vi "ScriptedStateMachine.vi"(8 "ErrorArray In":errorcluster[](array[cluster]), 9 "Data in":variant, 10 "Script":string[](array[string])=["Test,1,2,3", "stop"], 11 "Bus":refnum<class "Bus.lvclass">) -> (0 "ErrorArray Out":errorcluster[](array[cluster]), 2 "Data out":variant, 3 "Bus":refnum<class "Bus.lvclass">)   [LabVIEW 2017, in "Bus_class.lvlib" / "Bus.lvclass"]
uses:
  Bus.lvclass
  Public/TypeDefs/clBusData.ctl
  FrontPanel/TypeDefs/clEventConfig.ctl
  Modules/PmuImpairPlugins/PmuImpairPluginBase_class/TypeDefs/clImpairConfig.ctl
  Modules/EventPlugins/EventPluginBaseClass/TypeDefs/clEvtReportArray.ctl
  Modules/EventPlugins/EventPluginBaseClass/TypeDefs/clEvtReport.ctl
  Modules/EventPlugins/EventPluginBaseClass/TypeDefs/dblEvtSignalArray.ctl
  Modules/NetworkImpairmentModule/PublicAPI/Arguments/Broadcasts/dblNetworkTime.ctl
  Modules/NetworkImpairmentModule/PublicAPI/Arguments/Broadcasts/dblPktLoss.ctl
  Modules/FlagImpairModule/PublicAPI/Arguments/Broadcasts/ui32FlagImpairmentArray.ctl
  Modules/OutputToFilePlugins/OutputToFileBasePlugin/Typedefs/PmuCfgOpt.ctl
  Bus.lvclass/Bus.ctl
  BdcstInfo.ctl
  ModuleType.ctl
  FrontPanel/TypeDefs/clFrontPanelControlRefs.ctl
  Modules/PmuImpairModule/PublicAPI/Arguments/Broadcasts/clErrorRpt.ctl
  Modules/EventPlugins/EventPluginBaseClass/TypeDefs/clEvtConfig.ctl
  Accessors/Read AppModuleID.vi
  Accessors/Read OutputToFileModuleID.vi
  <vilib>/Utility/error.llb/Error Cluster From Error Code.vi
  <vilib>/Analysis/1siggen.llb/Ramp Pattern by Delta.vi
  <vilib>/ErrorRing/Error Ring.xnode
  <userlib>/NIST/NISTErrorLib/NISTErrorLib.lvlib
  Framework.lvlib
  Modules/EventModule/EventModule.lvlib
  Modules/EventPlugins/EventPluginBaseClass/EventPluginBaseClass.lvclass
  <vilib>/Analysis/NI_AALBase.lvlib
  Modules/PmuImpairModule/PmuImpairModule.lvlib
  Modules/NetworkImpairmentModule/NetworkImpairmentModule.lvlib
  Modules/FlagImpairModule/FlagImpairModule.lvlib
  Modules/PmuImpairPlugins/PmuImpairPluginBase_class/PmuImpairPluginBase.lvclass
  Modules/OutputToFilePlugins/OutputToFileBasePlugin/OutputToFileBasePlugin.lvclass
  Modules/OutputToFileModule/OutputToFileModule.lvlib
  Modules/AppModule/AppModule.lvlib
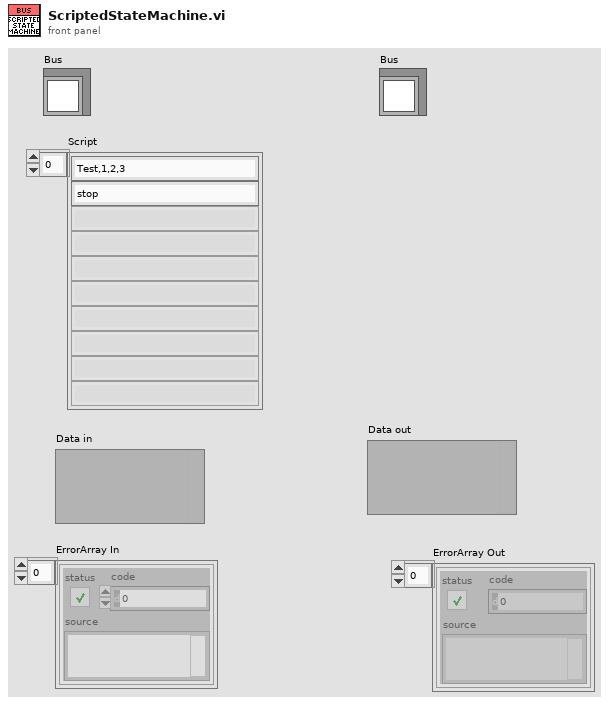
[diagram p1: front panel]
types:
  T1 = typedef "Bus_class.lvlib/Bus.lvclass/clBusData.ctl" = cluster{"BusNumber":u8, "EvtPluginINIFilePath":path, "EvtParams":string[][], "EvtConfig":T2, "Start Time":dbl, "End Time":dbl, "PmuImpairPluginINIFilePath":path, "PmuImpairParams ":string[][], "PmuImpairConfig":T3, "NetImpPluginINIFilePath":path, "NetImpParams":string[][], "FlagImpPluginINIFilePath":path, "FlagImpParams":string[][], "EvtReportArray":T4, "EventSignalArray":T6, "ImpairReportArray":T4, "NetworkTime":T7, "PktLoss":T8, "FlagImpArray":T9, "OutputToFilePluginINIFilePath":path, "Output File Path":path, "clConfigOptions":T10, "AppPluginINIFilePath":path, "AppConfig":variant, "AppOutput":variant}
  T2 = typedef "Framework.lvlib/clEventConfig.ctl" = cluster{"UTC Time 0":timestamp, "Nominal Frequency":u16, "Reporting Rate":u16, "Fsamp":u32, "PosSeq":bool}
  T3 = typedef "PmuImpairPlugins.lvlib/PmuImpairPluginBase.lvclass/clImpairConfig.ctl" = cluster{"FilterType":string, "bPosSeq":bool}
  T4 = typedef "EventPlugins.lvlib/EventPluginBaseClass.lvclass/clEvtReportArray.ctl" = T5[]
  T5 = typedef "EventPlugins.lvlib/EventPluginBaseClass.lvclass/clEvtReport.ctl" = cluster{"Timestamp":dbl, "Synx":cdb[], "Freq":dbl, "ROCOF":dbl, "ID":i16}
  T6 = typedef "EventPlugins.lvlib/EventPluginBaseClass.lvclass/dblEvtSignalArray.ctl" = dbl[][]
  T7 = typedef "NetworkImpairmentModule.lvlib/dblNetworkTime.ctl" = dbl[]
  T8 = typedef "NetworkImpairmentModule.lvlib/dblPktLoss.ctl" = dbl[]
  T9 = typedef "FlagImpairModule.lvlib/ui32FlagImpairmentArray.ctl" = u32[]
  T10 = typedef "OutputToFilePlugins.lvlib/OutputToFileBasePlugin.lvclass/PmuCfgOpt.ctl" = cluster{"TIME_BASE":u64, "STN":string, "IDCODE":u16, "rdoPolRect":enum32{"Rectangular", "Polar"}, "rdoFloatInt":enum32{"Float", "Integer"}, "PHUNIT":u64, "rdoFreqDfreq":enum32{"Float", "Integer"}, "CHNAM":string[], "chkCfg2Prefix":bool}
  T11 = typedef "Bus_class.lvlib/Bus.lvclass/ModuleType.ctl" = enum16{"PMU", "Event", "Network", "Flag", "App", "OutToFile"}
  T12 = typedef "Bus_class.lvlib/Bus.lvclass/BdcstInfo.ctl" = cluster{"ModuleType":T11, "ModuleID":i32, "UsrEvtRef":variant, "ScriptCmd":string}
  T13 = typedef "Framework.lvlib/clFrontPanelControlRefs.ctl" = cluster{"TestFilePathRef":refnum<vi>, "BusNumberRef":refnum<vi>, "NumberOfBusesRef":refnum<vi>, "EvtTypeRef":refnum<vi>, "EvtParamsRef":refnum<vi>, "EvtConfigRef":refnum<vi>, "StartTimeRef":refnum<vi>, "EndTimeRef":refnum<vi>, "PmuImpairTypeRef":refnum<vi>, "PmuImpairParamsRef":refnum<vi>, "NetImpairParamsRef":refnum<vi>, "FlagImpairTypeRef":refnum<vi>, "FlagImpairParamsRef":refnum<vi>, "NetImpairTypeRef":refnum<vi>, "OutputFileType":refnum<vi>, "PmuImpairConfigRef":refnum<vi>, "AppTypeRef":refnum<vi>, "ScriptPathRef":refnum<vi>, "ShowPanels?":refnum<vi>}
  T14 = typedef "PmuImpairModule.lvlib/clErrorRpt.ctl" = cluster{"error":errorcluster, "AdditionalInfo":string}
  T15 = typedef "EventPlugins.lvlib/EventPluginBaseClass.lvclass/clEvtConfig.ctl" = cluster{"T0(UTC)":dbl, "F0":dbl, "Fs":i32, "FSamp":u32, "bPosSeq":bool}
  T16 = typedef "EventModule.lvlib/clBroadcastEvents.ctl" = cluster{"DidInit":refnum<user-event>, "StatusUpdate":refnum<user-event>, "ErrorReport":refnum<user-event>, "DidStop":refnum<user-event>, "ReadEvtConfig":refnum<user-event>, "ReadTimeArray":refnum<user-event>, "ReadEvtParams":refnum<user-event>, "GetEvtReportArray":refnum<user-event>, "ReadPathToPlugin":refnum<user-event>, "GetEvtSignal":refnum<user-event>, "ReadBusNumber":refnum<user-event>}
  T17 = typedef "PmuImpairModule.lvlib/clBroadcastEvents.ctl" = cluster{"DidInit":refnum<user-event>, "StatusUpdate":refnum<user-event>, "ErrorReport":refnum<user-event>, "DidStop":refnum<user-event>, "ImpairConfig":refnum<user-event>, "ImpairParams":refnum<user-event>, "ImpairReports":refnum<user-event>, "PathToPlugin":refnum<user-event>, "BusNumber":refnum<user-event>}
  T18 = typedef "NetworkImpairmentModule.lvlib/clBroadcastEvents.ctl" = cluster{"DidInit":refnum<user-event>, "StatusUpdate":refnum<user-event>, "ErrorReport":refnum<user-event>, "DidStop":refnum<user-event>, "ReadNetImpParams":refnum<user-event>, "ReadLossThreshold":refnum<user-event>, "GetNetworkTime":refnum<user-event>, "GetPktLoss":refnum<user-event>, "ReadPathToPlugin":refnum<user-event>}
  T19 = typedef "FlagImpairModule.lvlib/clBroadcastEvents.ctl" = cluster{"DidInit":refnum<user-event>, "StatusUpdate":refnum<user-event>, "ErrorReport":refnum<user-event>, "DidStop":refnum<user-event>, "ReadFlagImpairConfig":refnum<user-event>, "ReadPluginINIFilePath":refnum<user-event>, "ReadFlagImpairParams":refnum<user-event>, "ReadTimeArray":refnum<user-event>, "GetFlagImpairment":refnum<user-event>}
  T20 = typedef "OutputToFileModule.lvlib/clBroadcastEvents.ctl" = cluster{"DidInit":refnum<user-event>, "StatusUpdate":refnum<user-event>, "ErrorReport":refnum<user-event>, "DidStop":refnum<user-event>, "PathToPlugin":refnum<user-event>, "PmuConfig":refnum<user-event>, "OutputPath":refnum<user-event>}
  T21 = typedef "AppModule.lvlib/clBroadcastEvents.ctl" = cluster{"DidInit":refnum<user-event>, "StatusUpdate":refnum<user-event>, "ErrorReport":refnum<user-event>, "DidStop":refnum<user-event>, "PathToINI":refnum<user-event>, "InputData":refnum<user-event>, "OutputData":refnum<user-event>, "BcAppInfo":refnum<user-event>, "ConfigData":refnum<user-event>}
  T22 = typedef "Framework.lvlib/clFrameworkData.ctl" = cluster{"EvtINIFilePaths":path[], "BusClassInstances":refnum<class "Bus.lvclass">[], "PmuImpairINIFilePaths":path[], "FlagImpairINIFilePaths":path[], "NetImpairINIFilePaths":path[], "OutputToFileINIFilePaths":path[], "AppINIFilePaths":path[], "AppModuleID":i32, "OutputToFileID":i32}
  T23 = typedef "Framework.lvlib/QueRef.ctl" = refnum<queue>
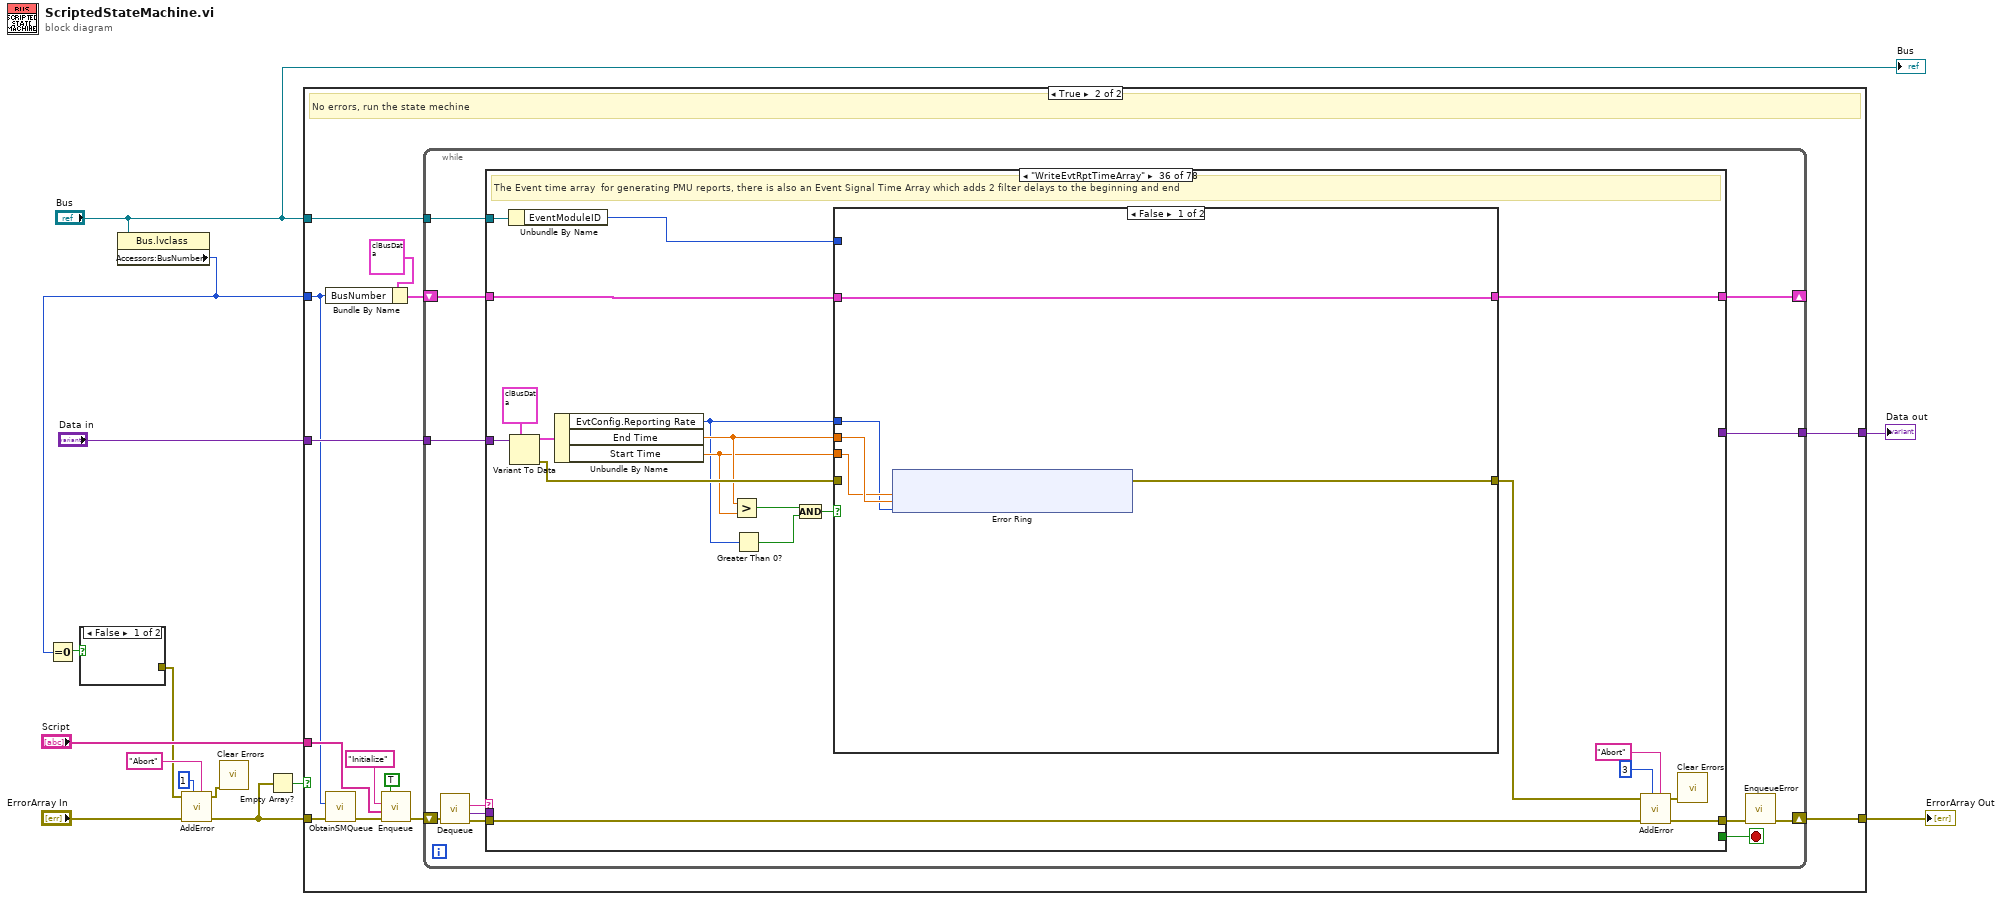
[diagram p0: block diagram]
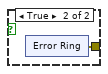
[diagram p2: hidden frame]
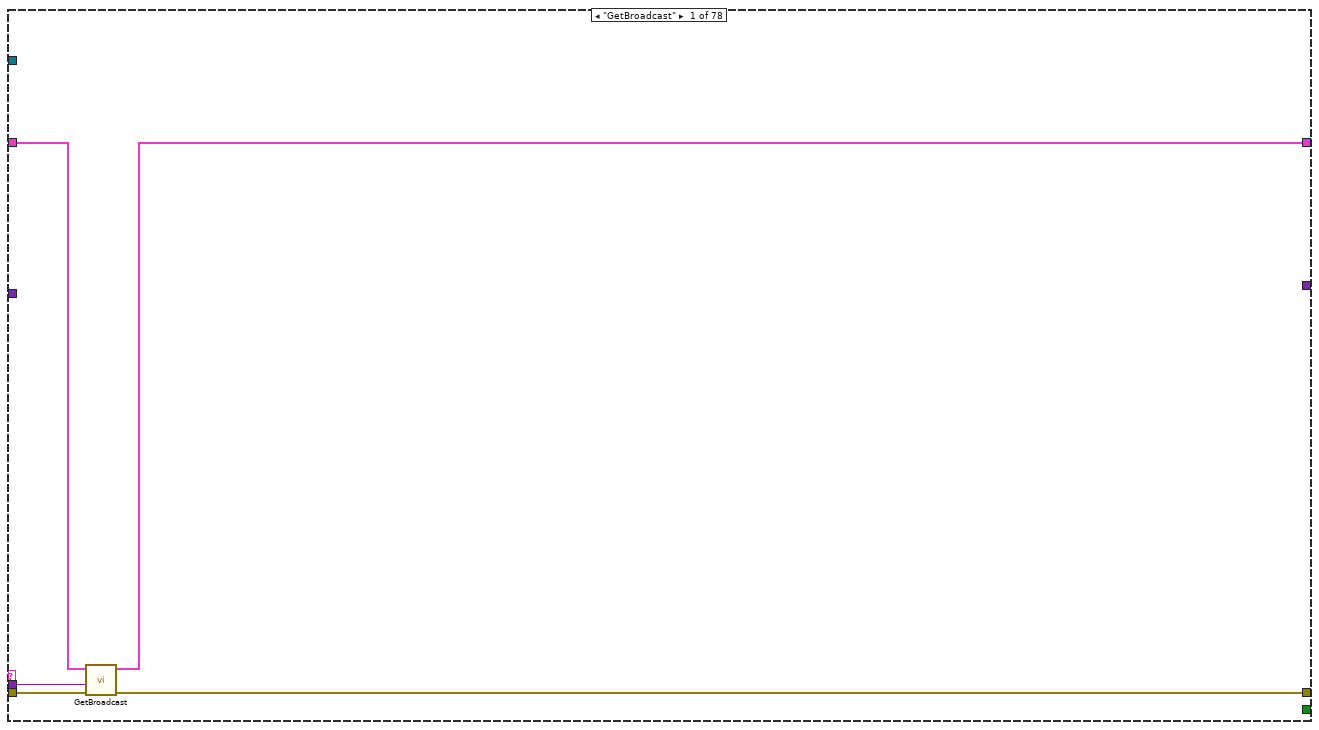
[diagram p4: hidden frame]
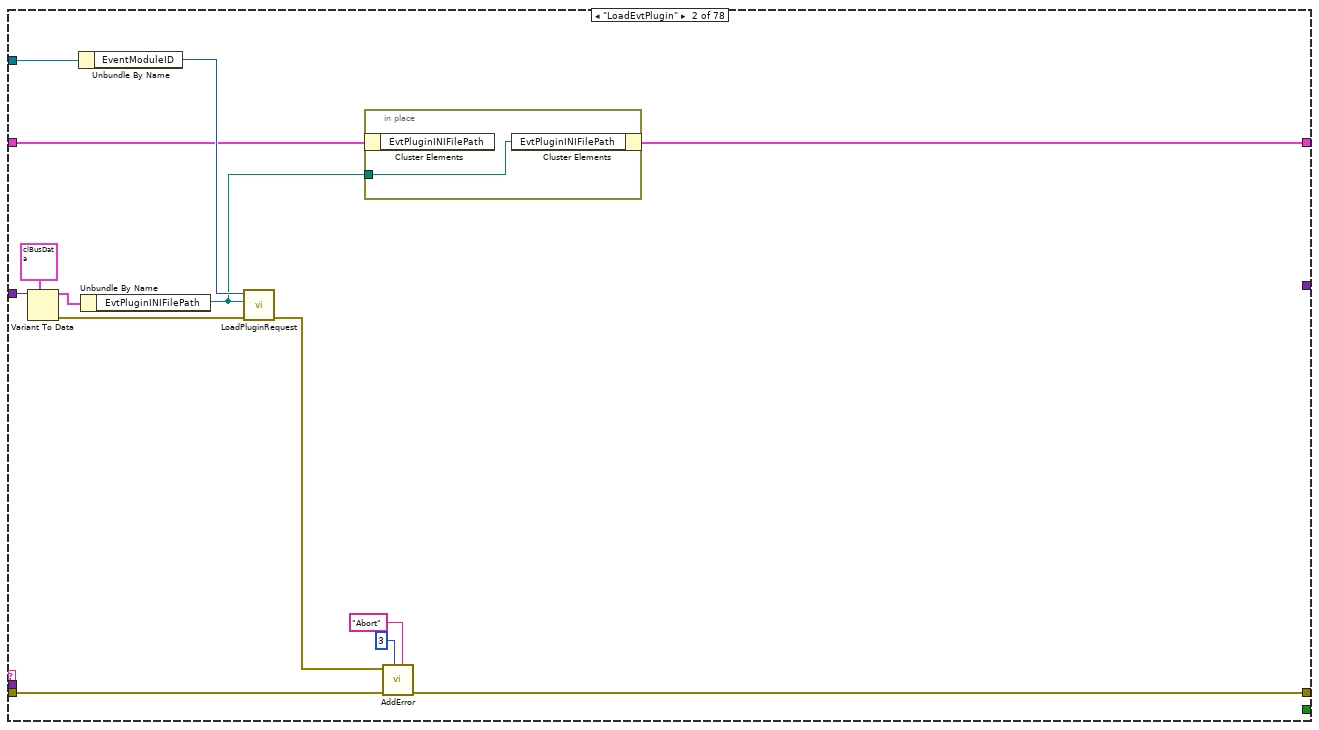
[diagram p5: hidden frame]
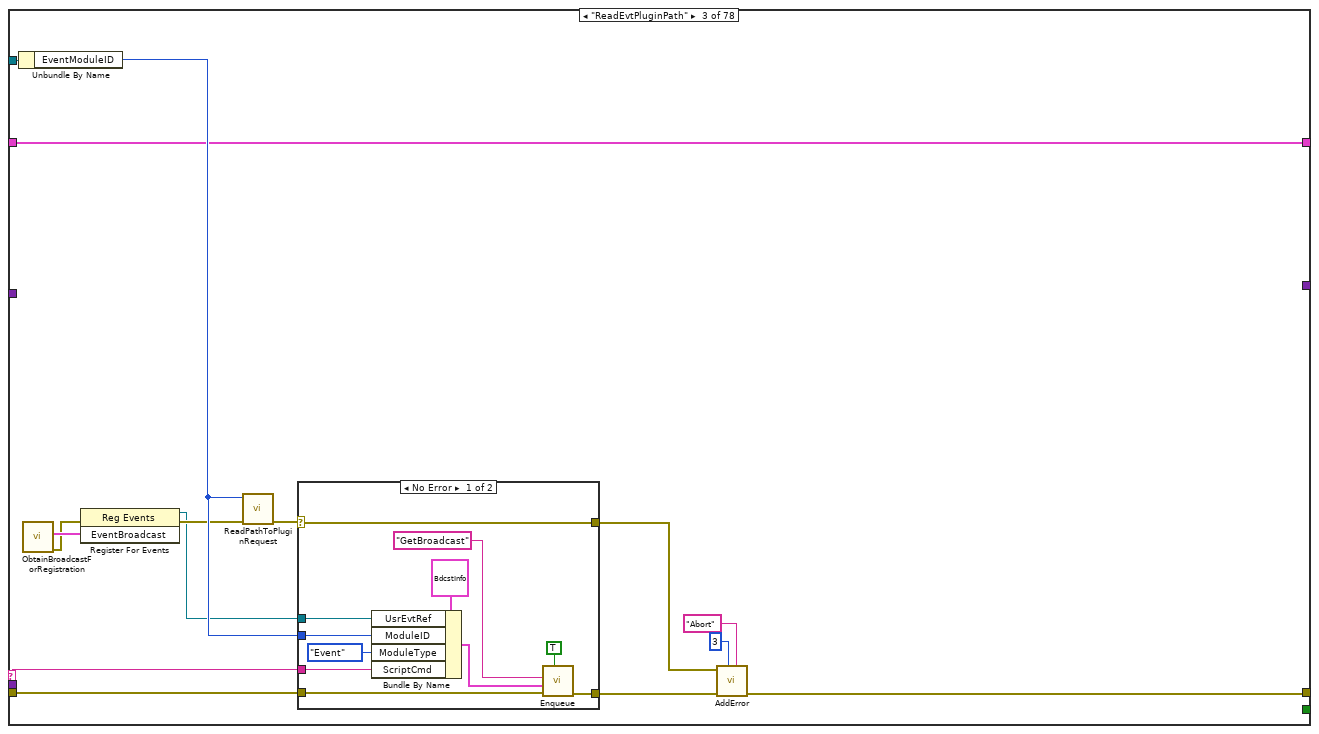
[diagram p6: hidden frame]
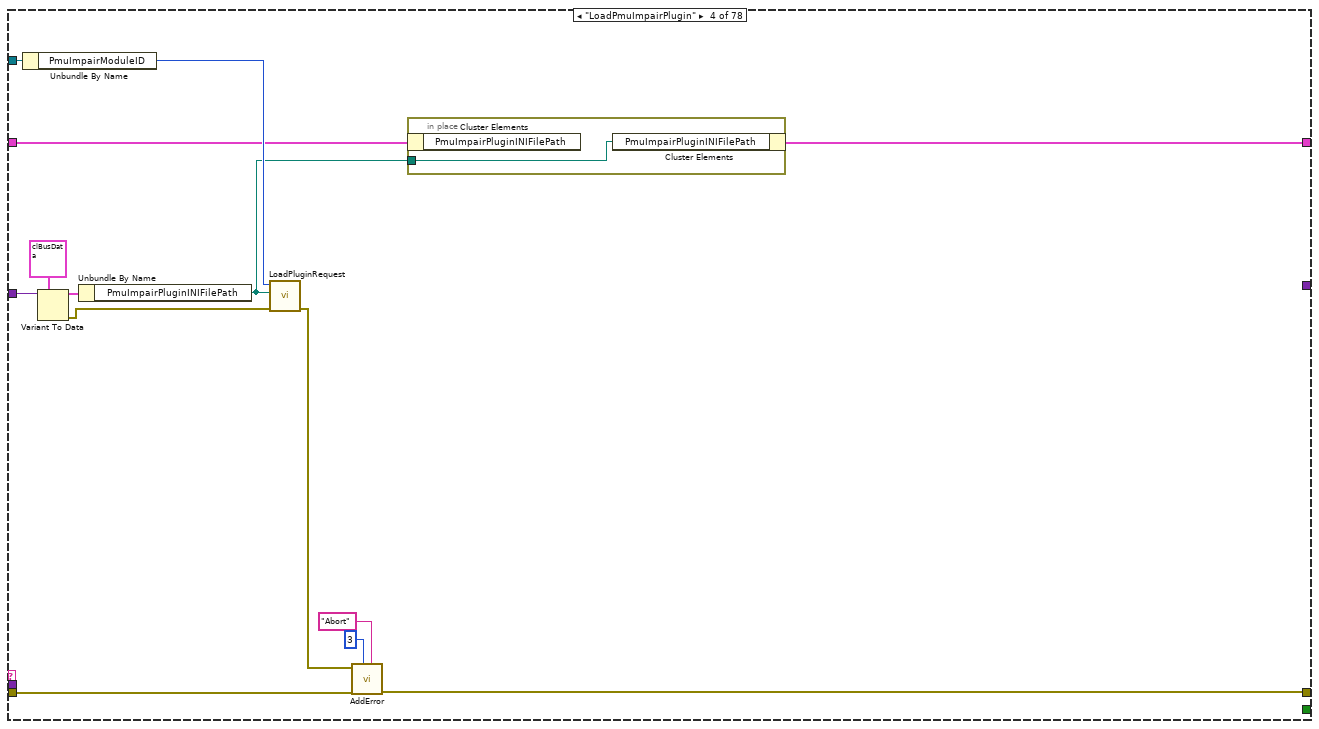
[diagram p8: hidden frame]
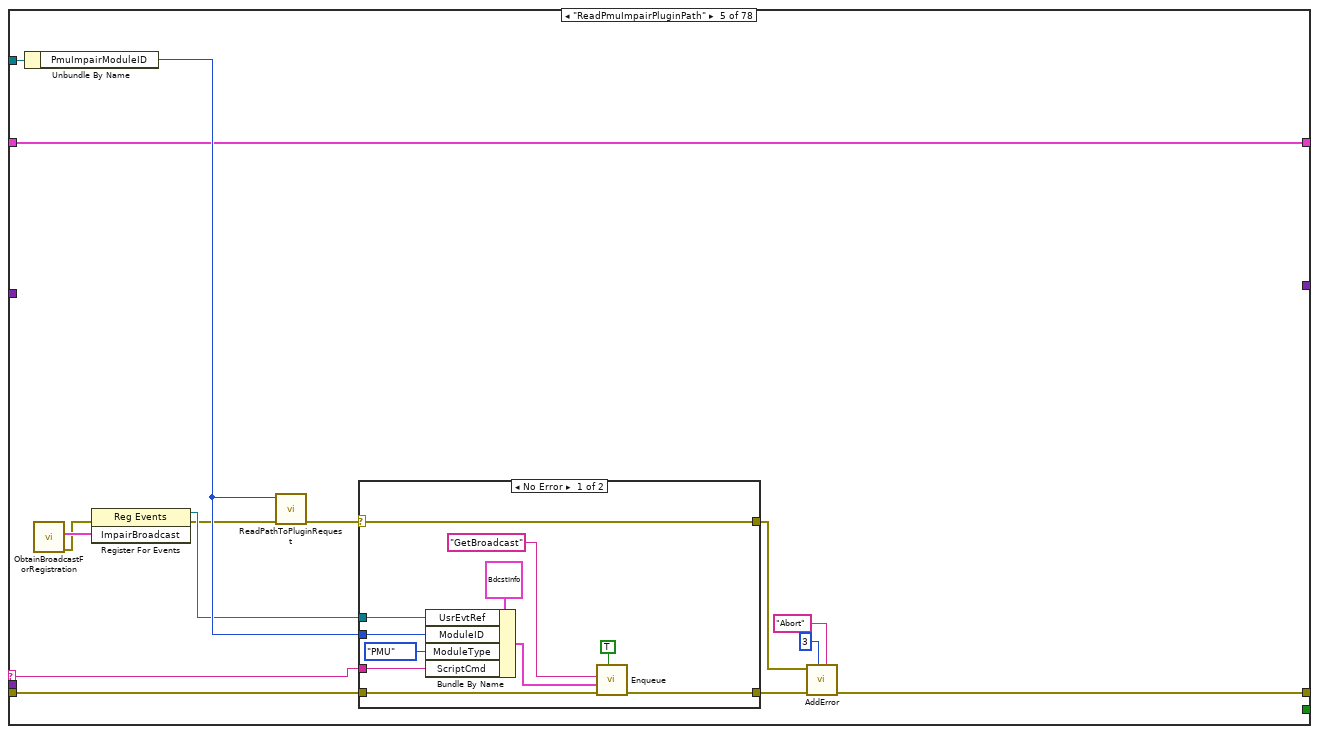
[diagram p9: hidden frame]
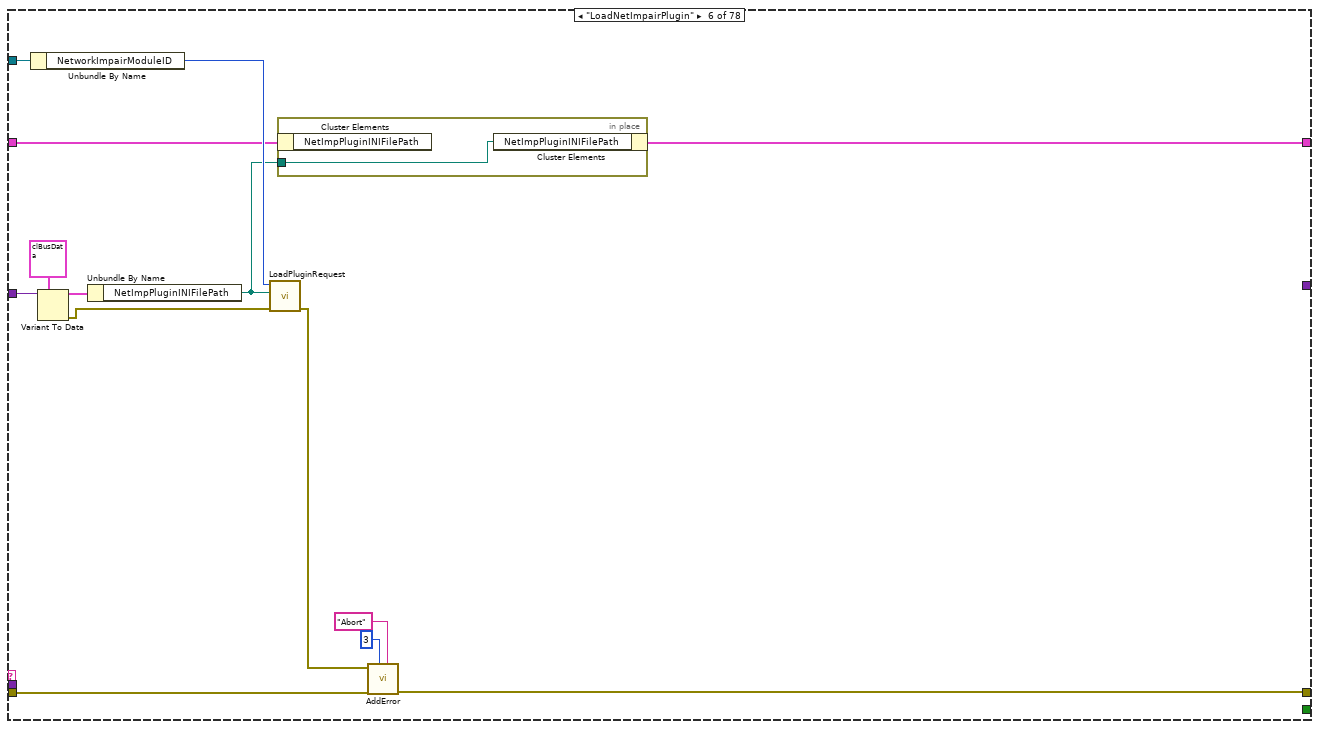
[diagram p11: hidden frame]
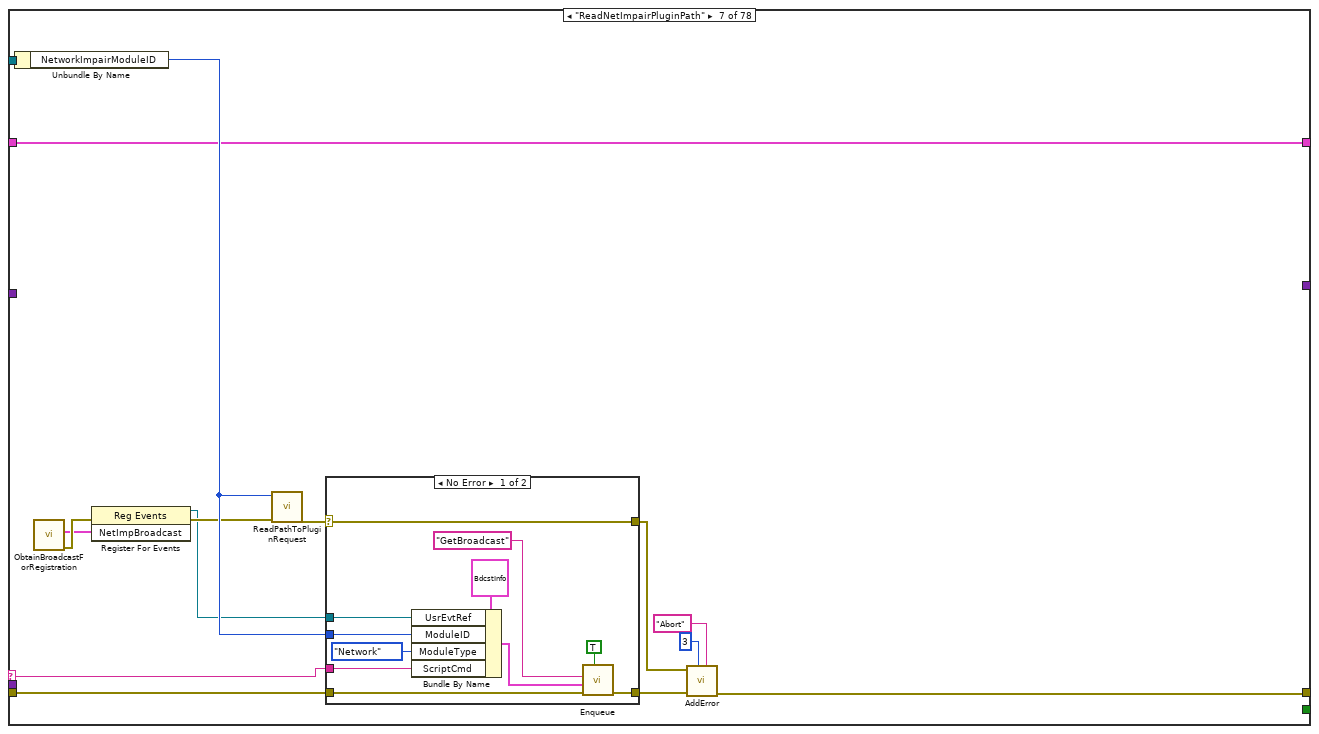
[diagram p12: hidden frame]
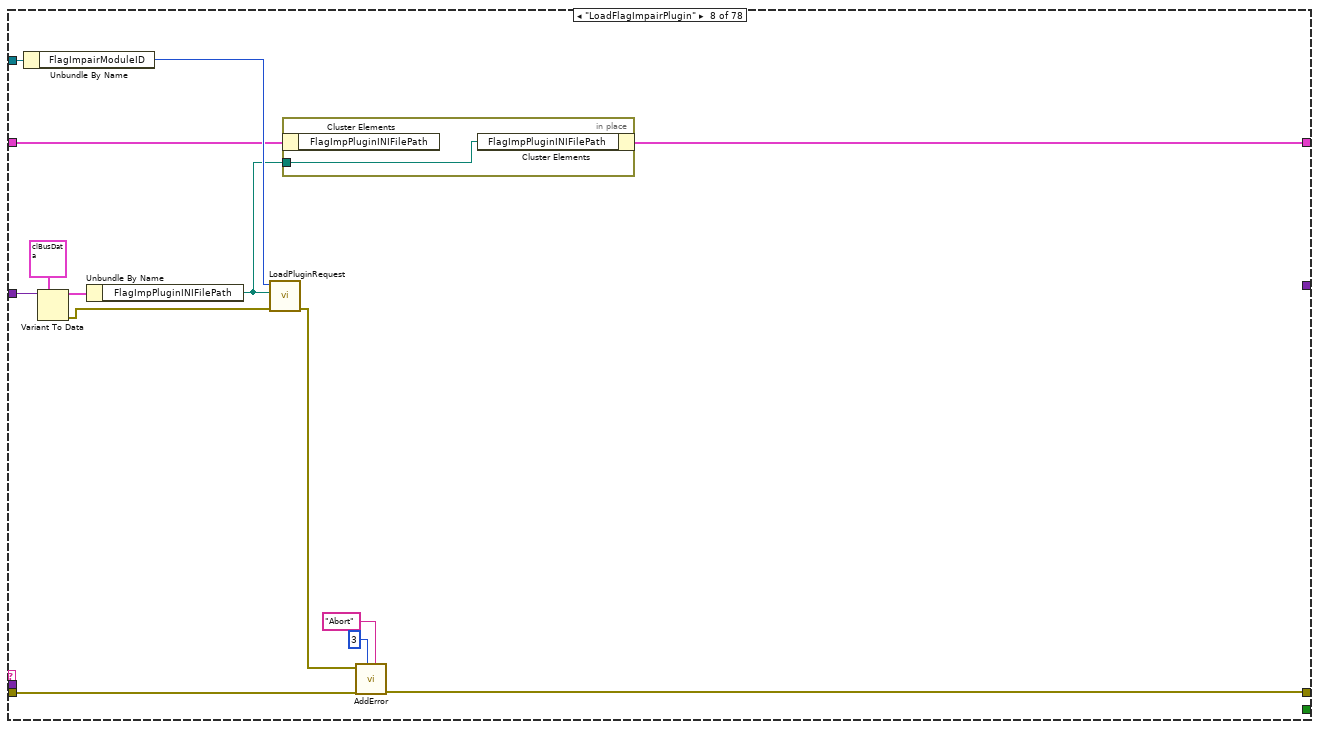
[diagram p14: hidden frame]
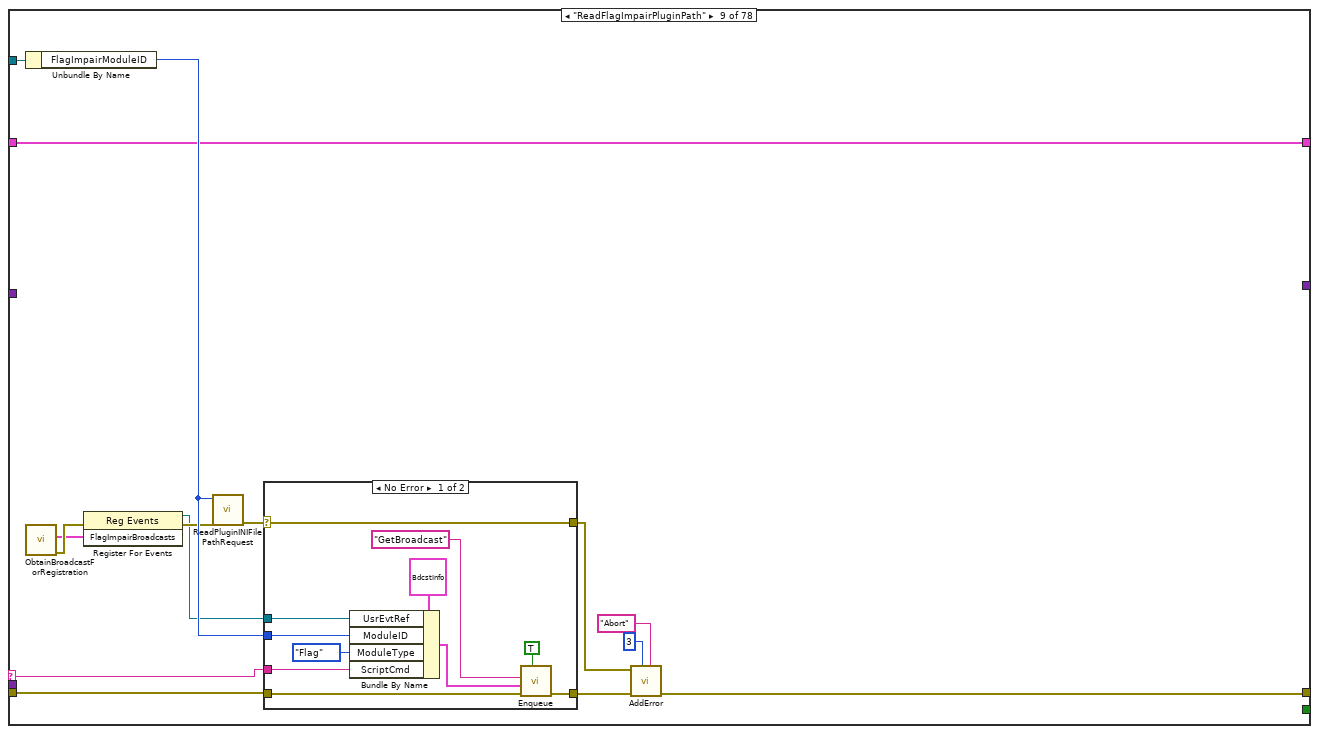
[diagram p15: hidden frame]
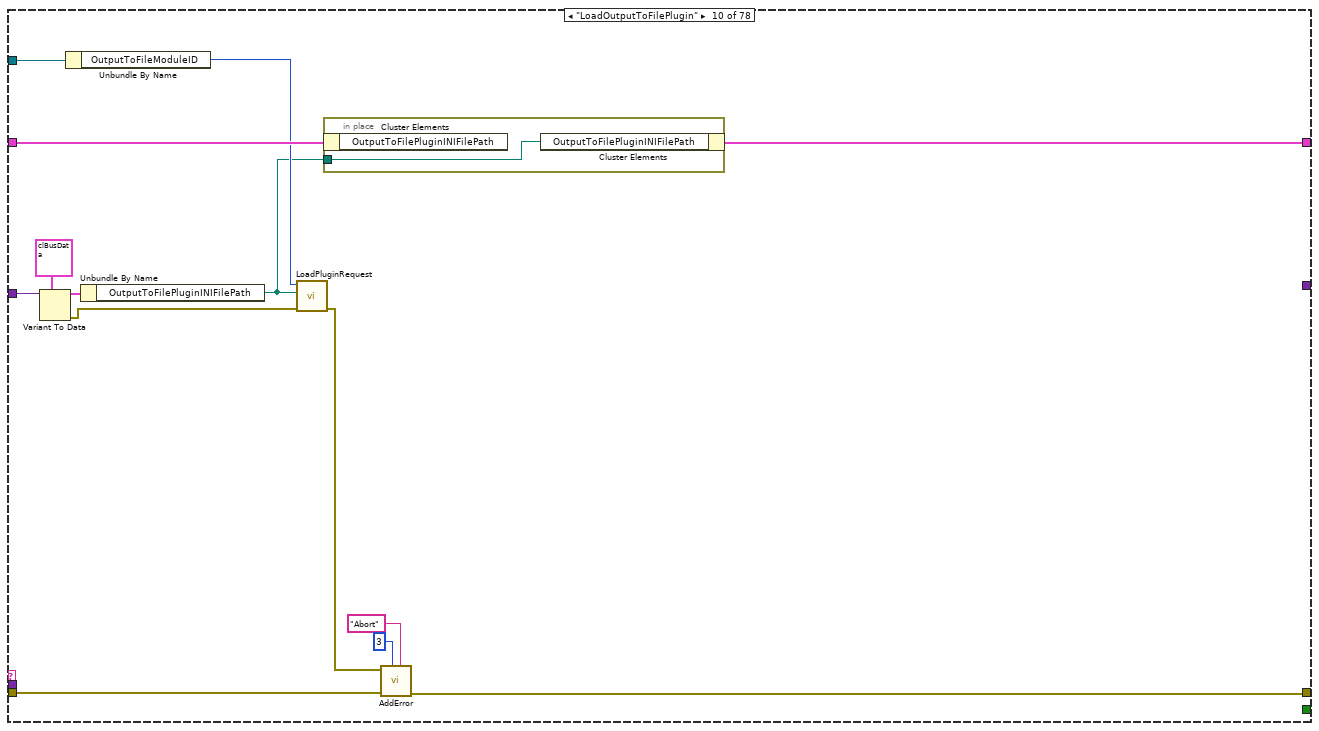
[diagram p17: hidden frame]
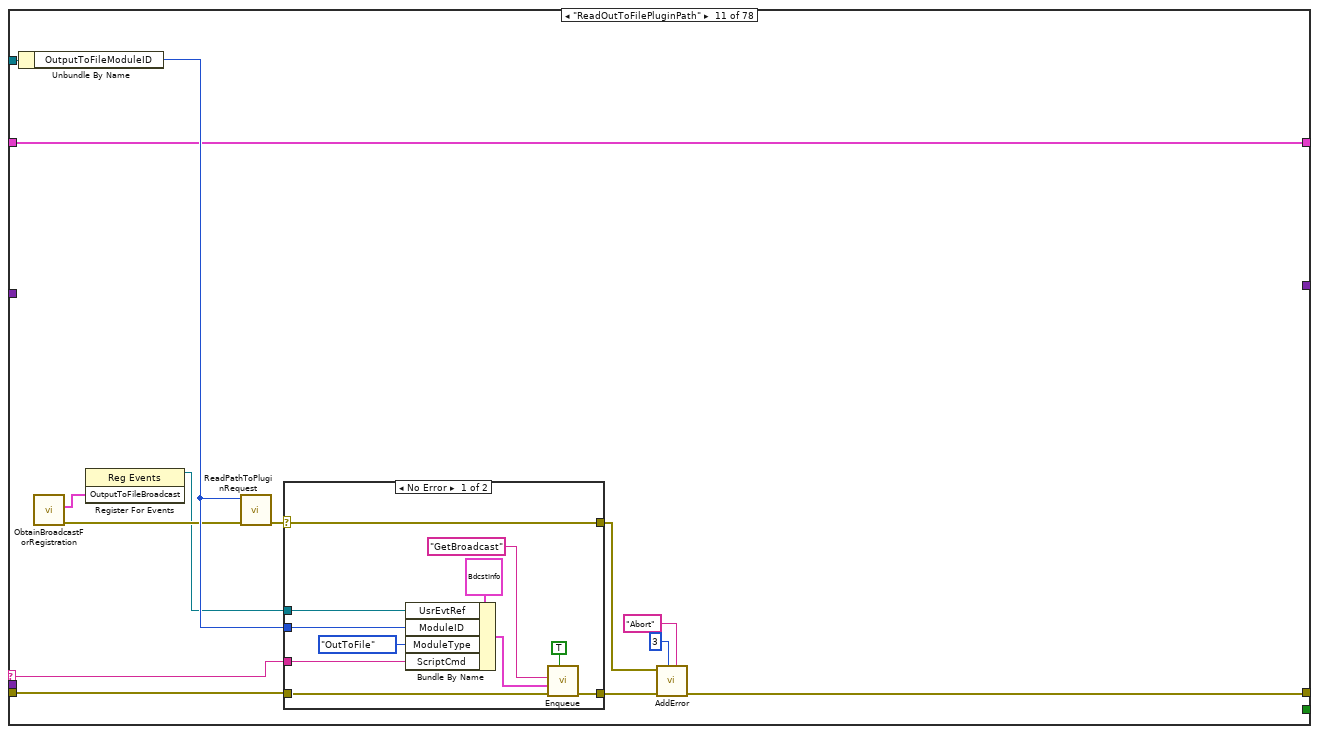
[diagram p18: hidden frame]
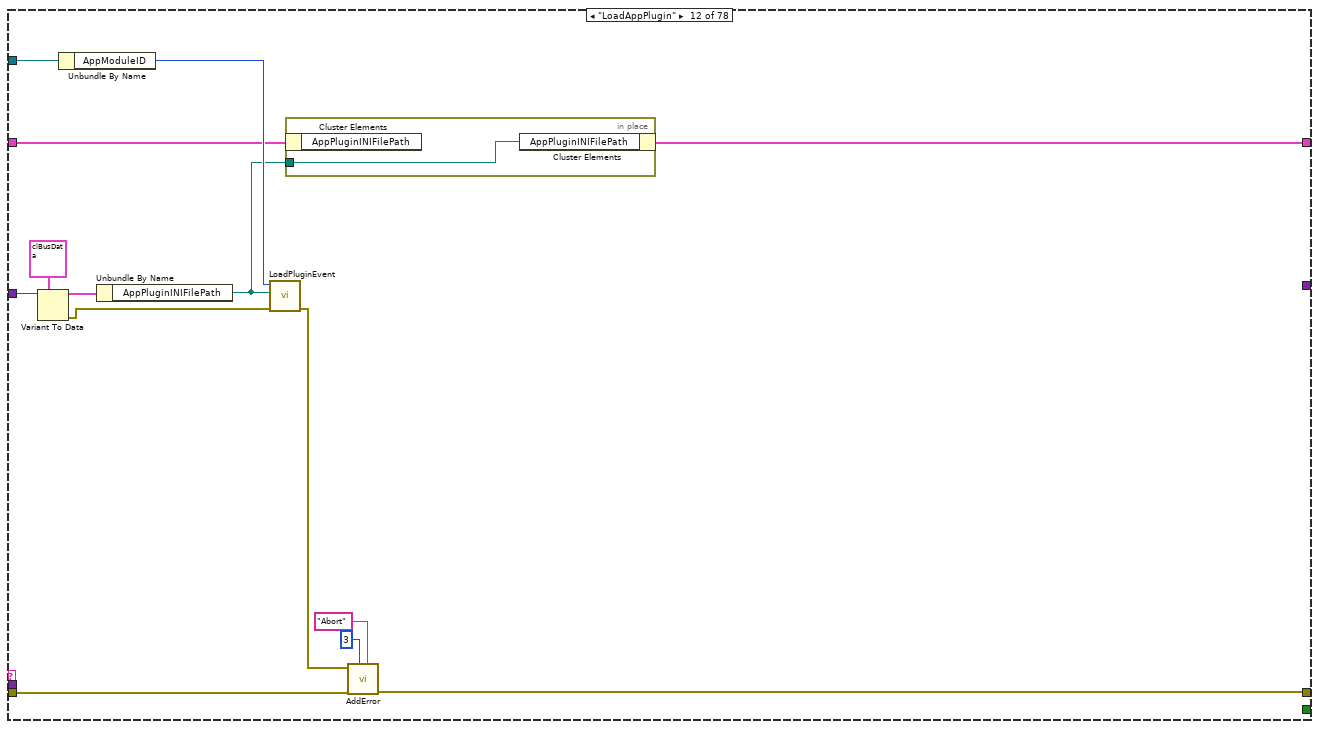
[diagram p20: hidden frame]
diagram:
  n1 = property class="Bus.lvclass"(reference="Bus") -> ("Accessors:BusNumber"=w2:u8)  [unwired: 1 in, 2 out]
  n2 = Equal To 0?(x=w2) -> (x = 0?=w5:bool)
  n3 = case shown="False" w5 {
    tunnel: [_ w15] -> w4
    frame False {
    }
    frame True {
      n4 = xnode "Error Ring"() -> ("error out"=w15:errorcluster)
    }
  }
  n5 = call <userlib>:"AddError.vi"("Severity"="Abort" ("String"), "Priority"=u8 1, "ErrorArray"="ErrorArray In", "error in (no error)"=w4) -> ("ErrorArray"=w8:errorcluster[], "error out"=w3:errorcluster)  [unwired: 6 in]
  n6 = call <vilib>:"Clear Errors.vi"("error in (no error)"=w3) -> ()  [unwired: 5 in, 2 out]
  n7 = Empty Array?(array=w8) -> (empty?=w14:bool)
  n8 = case shown="True" w14 {
    tunnel: w8 -> [w17 w30]
    tunnel: [w17 w25] -> w13
    tunnel: "Bus" -> [_ w24]
    tunnel: "Script" -> [_ w23]
    tunnel: "Data in" -> [_ w22]
    tunnel: [_ w21] -> w10
    tunnel: w2 -> [_ w18]
    frame False {
      # "Errors coming into the state machine, don't run it."
    }
    frame True {
      # "No errors, run the state mechine"
      n9 = Bundle By Name(cluster=T1 {"BusNumber"=0, "EvtPluginINIFilePath"=path "", "EvtParams"=[], "EvtConfig"={"UTC Time 0"=timestamp(0 s since 1904-01-01), "Nominal Frequency"=60, "Reporting Rate"=60, "Fsamp"=960, "PosSeq"=FALSE}, "Start Time"=0.0, "End Time"=0.0, "PmuImpairPluginINIFilePath"=path "", "PmuImpairParams "=[["960"], ["8.19"], ["164"]], "PmuImpairConfig"={"FilterType"="", "bPosSeq"=TRUE}, "NetImpPluginINIFilePath"=path "", "NetImpParams"=[], "FlagImpPluginINIFilePath"=path "", "FlagImpParams"=[], "EvtReportArray"=[], "EventSignalArray"=[], "ImpairReportArray"=[], "NetworkTime"=[], "PktLoss"=[], "FlagImpArray"=[], "OutputToFilePluginINIFilePath"=path "", "Output File Path"=path "", "clConfigOptions"={"TIME_BASE"=1000000, "STN"="Bus_1", "IDCODE"=0, "rdoPolRect"=enum."Rectangular", "rdoFloatInt"=enum."Float", "PHUNIT"=1000000, "rdoFreqDfreq"=enum."Float", "CHNAM"=["VA", "VB", "VC", "V+", "IA", "IB", "IC", "I+"], "chkCfg2Prefix"=TRUE}, "AppPluginINIFilePath"=path "", "AppConfig"=variant, "AppOutput"=variant} ("clBusData"), "BusNumber"=w18) -> (w19:T1)
      n10 = call "ObtainSMQueue.vi"("ErrorArray"=w30, "BusNumber"=w18) -> ("ErrorArray"=w29:errorcluster[])  [unwired: 8 in, 1 out]
      n11 = call "Enqueue.vi"("Priority (f)"=TRUE, "ErrorArray"=w29, "Data"=w23, "Msg"="Initialize") -> ("ErrorArray"=w26:errorcluster[])  [unwired: 7 in]
      n12 = while {
        shift-right: [w37] -> w25
        shift-left: w26 -> [w42]
        tunnel: w24 -> [w35]
        tunnel: w22 -> [w34]
        tunnel: [w33] -> w21
        shift-right: [w32] -> _
        shift-left: w19 -> [w31]
        stop <- w38 stop-if-true
        n13 = call "Dequeue.vi"("ErrorArray"=w42) -> ("ErrorArray"=w40:errorcluster[], "Data"=w39:variant, "Msg"=w41:string)  [unwired: 8 in]
        n14 = case shown="\"WriteEvtRptTimeArray\"" w41 {
          selector: w41 -> [_ _ w70 _ w114 _ w156 _ w199 _ w241 _ w283 _ _ _ _ _ _ _ w480 _ w524 w556 _ w602 w629 _ w671 _ w708 _ w754 _ w808 _ w883 w913 _ _ _ w998 _ w1048 _ w1093 _ _ w1149 _ _ _ _ _ _ _ _ _ _ _ _ w1359 _ _ w1420 _ _ _ _ _ w1543 _ w1594 w1623 _ w1666 w1714 w1751]
          tunnel: w40 -> [w44 w53 w69 w96 w112 w139 w155 w182 w198 w221 w240 w267 w282 w331 w339 w369 w385 w404 w416 w429 w478 w520 w529 w555 w586 w601 w628 w652 w670 w701 w715 w742 w761 w796 w815 w845 w890 w918 w957 w973 w984 w1005 w1033 w1046 w1073 w1091 w1119 w1133 w1147 w1227 w1237 w1247 w1257 w1267 w1278 w1288 w1298 w1314 w1323 w1333 w1347 w1367 w1389 w1408 w1428 w1450 w1467 w1485 w1521 w1536 w1542 _ w1599 w1628 w1652 w1672 w1711 w1757]
          tunnel: w39 -> [w43 _ _ _ _ _ _ _ _ _ _ _ _ _ _ _ _ _ _ _ _ _ _ _ _ _ _ _ _ _ _ _ _ _ _ _ _ _ _ _ _ _ _ _ _ _ _ _ _ _ _ _ _ _ _ _ _ _ _ _ _ _ _ _ _ _ _ w1483 _ _ _ w1562 _ _ _ _ _ _]
          tunnel: [w45 w55 w73 w97 w116 w140 w159 w183 w202 w223 w244 w268 w286 w305 w343 w376 w386 w407 w419 w429 w474 w515 w531 w559 w588 w605 w632 w654 w674 w703 w717 w744 w763 w798 w817 w846 w894 w920 w940 w974 w986 w1007 w1035 w1049 w1075 w1094 w1121 w1141 w1150 w1233 w1239 w1249 w1259 w1269 w1280 w1290 w1300 w1316 w1325 w1335 w1349 w1369 w1390 w1410 w1430 w1452 w1470 w1486 w1524 w1528 w1541 w1556 w1603 w1632 w1653 w1676 w1696 w1761] -> w36
          tunnel: [_ _ _ _ _ _ _ _ _ _ _ _ _ _ _ _ _ _ _ _ _ _ _ _ _ _ _ _ _ _ _ _ _ _ _ _ _ _ _ _ _ _ _ _ _ _ _ _ _ _ _ _ _ _ _ _ _ _ _ _ _ _ _ _ _ _ _ _ _ TRUE _ _ _ _ _ _ _ _] -> w38
          tunnel: w35 -> [_ w59 w77 w104 w120 w147 w163 w190 w206 w233 w248 w275 w290 _ _ _ _ _ _ _ w486 w522 w536 w563 w585 w609 w636 w659 w678 w700 w721 w741 w767 w805 w822 w855 w897 w925 _ w983 _ w1010 w1032 w1054 w1083 w1099 w1128 w1140 w1157 w1232 w1245 w1255 w1265 w1275 w1285 w1295 w1305 w1321 w1330 w1340 w1357 w1373 w1400 w1418 w1434 w1458 w1473 _ _ _ _ w1555 w1608 w1637 w1663 w1681 _ w1766]
          tunnel: w34 -> [_ w61 _ w102 _ w145 _ w188 _ w231 _ w273 _ w337 w361 w382 w402 w414 w426 _ _ _ _ _ w593 _ _ w663 _ w698 _ w750 _ w803 _ w854 _ _ _ _ _ _ w1028 _ w1081 _ w1126 w1138 _ w1230 _ _ _ _ _ _ _ _ _ _ w1355 _ _ w1416 _ w1463 _ _ _ _ _ _ _ _ _ _ _ _]
          tunnel: [_ _ _ _ _ _ _ _ _ _ _ _ _ _ _ _ _ _ _ _ _ _ _ _ _ _ _ _ _ _ _ _ _ _ _ _ _ _ _ _ _ _ _ _ _ _ _ _ _ _ _ _ _ _ _ _ _ _ _ _ _ _ _ _ _ _ _ _ _ w1526 variant ("Data in") _ _ _ _ _ _ _] -> w33
          tunnel: [w46 w48 w71 w91 w115 w134 w157 w178 w200 w226 w242 w262 w284 w304 w341 w374 w384 w406 w418 w427 w479 w516 w530 w557 w582 w603 w630 w651 w672 w692 w716 w736 w762 w783 w816 w842 w892 w919 w939 w960 w990 w1006 w1025 w1052 w1068 w1097 w1115 w1130 w1154 w1215 w1246 w1256 w1266 w1276 w1286 w1296 w1306 w1322 w1331 w1341 w1343 w1368 w1399 w1404 w1429 w1449 w1472 w1474 w1520 w1525 w1538 w1554 w1600 w1631 w1662 w1675 w1708 w1760] -> w32
          tunnel: w31 -> [w47 w49 w71 w92 w115 w136 w157 w179 w200 w232 w242 w264 w284 w304 w341 w374 w384 w406 w418 w428 w479 w516 w530 w557 w583 w603 w630 w661 w672 w694 w716 w737 w762 w784 w816 w843 w892 w919 w939 w960 w990 w1006 w1027 w1052 w1069 w1097 w1116 w1132 w1155 w1215 w1246 w1256 w1266 w1276 w1286 w1296 w1306 w1322 w1331 w1341 w1344 w1368 w1399 w1405 w1429 w1461 w1472 w1474 w1520 w1525 w1538 w1554 w1600 w1631 w1662 w1675 w1709 w1760]
          frame "GetBroadcast" {
            n15 = call "GetBroadcast.vi"("Error In"=w44, "BdcstInfo"=w43, "clBusData In"=w47) -> ("Error Out"=w45:errorcluster[], "clBusData Out"=w46:T1)  [unwired: 7 in]
          }
          frame "LoadEvtPlugin" {
            n16 = Variant To Data(type=T1 {"BusNumber"=0, "EvtPluginINIFilePath"=path "", "EvtParams"=[], "EvtConfig"={"UTC Time 0"=timestamp(0 s since 1904-01-01), "Nominal Frequency"=60, "Reporting Rate"=60, "Fsamp"=960, "PosSeq"=FALSE}, "Start Time"=0.0, "End Time"=0.0, "PmuImpairPluginINIFilePath"=path "", "PmuImpairParams "=[["960"], ["8.19"], ["164"]], "PmuImpairConfig"={"FilterType"="", "bPosSeq"=TRUE}, "NetImpPluginINIFilePath"=path "", "NetImpParams"=[], "FlagImpPluginINIFilePath"=path "", "FlagImpParams"=[], "EvtReportArray"=[], "EventSignalArray"=[], "ImpairReportArray"=[], "NetworkTime"=[], "PktLoss"=[], "FlagImpArray"=[], "OutputToFilePluginINIFilePath"=path "", "Output File Path"=path "", "clConfigOptions"={"TIME_BASE"=1000000, "STN"="Bus_1", "IDCODE"=0, "rdoPolRect"=enum."Rectangular", "rdoFloatInt"=enum."Float", "PHUNIT"=1000000, "rdoFreqDfreq"=enum."Float", "CHNAM"=["VA", "VB", "VC", "V+", "IA", "IB", "IC", "I+"], "chkCfg2Prefix"=TRUE}, "AppPluginINIFilePath"=path "", "AppConfig"=variant, "AppOutput"=variant} ("clBusData"), Variant=w61) -> (data=w51:T1, error out=w52:errorcluster)  [unwired: 1 in]
            n17 = Unbundle By Name(w59) -> ("EventModuleID"=w58:i32)
            n18 = Unbundle By Name(w51) -> ("EvtPluginINIFilePath"=w50:path)
            n19 = call "LoadPluginRequest.vi"("error in (no error)"=w52, "PathToPlugin"=w50, "ModuleID"=w58) -> ("error out"=w54:errorcluster)  [unwired: 8 in]
            n20 = in-place {
              in-place-border: w50 -> [w62]
              n21 = in-place-cluster #1(w49) -> ()  [unwired: 1 out]
              n22 = in-place-cluster #1("EvtPluginINIFilePath"=w62) -> (w48:T1)
            }
            n23 = call <userlib>:"AddError.vi"("Severity"="Abort" ("String"), "Priority"=u8 3, "ErrorArray"=w53, "error in (no error)"=w54) -> ("ErrorArray"=w55:errorcluster[])  [unwired: 6 in, 1 out]
          }
          frame "ReadEvtPluginPath" {
            n24 = Unbundle By Name(w77) -> ("EventModuleID"=w76:i32)
            n25 = call "ObtainBroadcastForRegistration.vi"() -> ("error out"=w65:errorcluster, "EventBroadcast"=w66:T16)  [unwired: 10 in]
            n26 = register-events(error in=w65, w66) -> (reference out=w63:refnum<event-registration>, error out=w64:errorcluster)  [unwired: 1 in]
            n27 = call "ReadPathToPluginRequest.vi"("error in (no error)"=w64, "ModuleID"=w76) -> ("error out"=w67:errorcluster)  [unwired: 9 in]
            n28 = case shown="No Error" w67 {
              selector: w67 -> [w80 w89]
              tunnel: w69 -> [w88 w90]
              tunnel: w76 -> [w85 _]
              tunnel: [w83 w90] -> w68
              tunnel: [w80 w89] -> w72
              tunnel: w70 -> [w79 _]
              tunnel: w63 -> [w78 _]
              frame No Error {
                n29 = Bundle By Name(cluster=T12 {"ModuleType"=enum."PMU", "ModuleID"=0, "UsrEvtRef"=variant, "ScriptCmd"=""} ("GetBdcstData"), "UsrEvtRef"=w78, "ModuleID"=w85, "ModuleType"=ModuleType."Event", "ScriptCmd"=w79) -> (w84:T12)
                n30 = call "Enqueue.vi"("Priority (f)"=TRUE, "ErrorArray"=w88, "Data"=w84, "Msg"="GetBroadcast") -> ("ErrorArray"=w83:errorcluster[])  [unwired: 7 in]
              }
              frame Error {
              }
            }
            n31 = call <userlib>:"AddError.vi"("Severity"="Abort" ("String"), "Priority"=u8 3, "ErrorArray"=w68, "error in (no error)"=w72) -> ("ErrorArray"=w73:errorcluster[])  [unwired: 6 in, 1 out]
          }
          frame "LoadPmuImpairPlugin" {
            n32 = Unbundle By Name(w104) -> ("PmuImpairModuleID"=w100:i32)
            n33 = Variant To Data(type=T1 {"BusNumber"=0, "EvtPluginINIFilePath"=path "", "EvtParams"=[], "EvtConfig"={"UTC Time 0"=timestamp(0 s since 1904-01-01), "Nominal Frequency"=60, "Reporting Rate"=60, "Fsamp"=960, "PosSeq"=FALSE}, "Start Time"=0.0, "End Time"=0.0, "PmuImpairPluginINIFilePath"=path "", "PmuImpairParams "=[["960"], ["8.19"], ["164"]], "PmuImpairConfig"={"FilterType"="", "bPosSeq"=TRUE}, "NetImpPluginINIFilePath"=path "", "NetImpParams"=[], "FlagImpPluginINIFilePath"=path "", "FlagImpParams"=[], "EvtReportArray"=[], "EventSignalArray"=[], "ImpairReportArray"=[], "NetworkTime"=[], "PktLoss"=[], "FlagImpArray"=[], "OutputToFilePluginINIFilePath"=path "", "Output File Path"=path "", "clConfigOptions"={"TIME_BASE"=1000000, "STN"="Bus_1", "IDCODE"=0, "rdoPolRect"=enum."Rectangular", "rdoFloatInt"=enum."Float", "PHUNIT"=1000000, "rdoFreqDfreq"=enum."Float", "CHNAM"=["VA", "VB", "VC", "V+", "IA", "IB", "IC", "I+"], "chkCfg2Prefix"=TRUE}, "AppPluginINIFilePath"=path "", "AppConfig"=variant, "AppOutput"=variant} ("clBusData"), Variant=w102) -> (data=w101:T1, error out=w95:errorcluster)  [unwired: 1 in]
            n34 = Unbundle By Name(w101) -> ("PmuImpairPluginINIFilePath"=w93:path)
            n35 = call "LoadPluginRequest.vi"("error in (no error)"=w95, "PathToPlugin"=w93, "ModuleID"=w100) -> ("error out"=w94:errorcluster)  [unwired: 8 in]
            n36 = call <userlib>:"AddError.vi"("Severity"="Abort" ("String"), "Priority"=u8 3, "ErrorArray"=w96, "error in (no error)"=w94) -> ("ErrorArray"=w97:errorcluster[])  [unwired: 6 in, 1 out]
            n37 = in-place {
              in-place-border: w93 -> [w105]
              n38 = in-place-cluster #2(w92) -> ()  [unwired: 1 out]
              n39 = in-place-cluster #2("PmuImpairPluginINIFilePath"=w105) -> (w91:T1)
            }
          }
          frame "ReadPmuImpairPluginPath" {
            n40 = Unbundle By Name(w120) -> ("PmuImpairModuleID"=w119:i32)
            n41 = call "ObtainBroadcastForRegistration.vi"() -> ("error out"=w108:errorcluster, "ImpairBroadcast"=w109:T17)  [unwired: 10 in]
            n42 = register-events(error in=w108, w109) -> (reference out=w107:refnum<event-registration>, error out=w106:errorcluster)  [unwired: 1 in]
            n43 = call "ReadPathToPluginRequest.vi"("error in (no error)"=w106, "ModuleID"=w119) -> ("error out"=w110:errorcluster)  [unwired: 9 in]
            n44 = case shown="No Error" w110 {
              selector: w110 -> [w125 w133]
              tunnel: [w128 w132] -> w111
              tunnel: [w125 w133] -> w113
              tunnel: w112 -> [w124 w132]
              tunnel: w119 -> [w123 _]
              tunnel: w114 -> [w122 _]
              tunnel: w107 -> [w121 _]
              frame No Error {
                n45 = Bundle By Name(cluster=T12 {"ModuleType"=enum."PMU", "ModuleID"=0, "UsrEvtRef"=variant, "ScriptCmd"=""} ("GetBdcstData"), "UsrEvtRef"=w121, "ModuleID"=w123, "ModuleType"=ModuleType."PMU", "ScriptCmd"=w122) -> (w129:T12)
                n46 = call "Enqueue.vi"("Priority (f)"=TRUE, "ErrorArray"=w124, "Data"=w129, "Msg"="GetBroadcast") -> ("ErrorArray"=w128:errorcluster[])  [unwired: 7 in]
              }
              frame Error {
              }
            }
            n47 = call <userlib>:"AddError.vi"("Severity"="Abort" ("String"), "Priority"=u8 3, "ErrorArray"=w111, "error in (no error)"=w113) -> ("ErrorArray"=w116:errorcluster[])  [unwired: 6 in, 1 out]
          }
          frame "LoadNetImpairPlugin" {
            n48 = Unbundle By Name(w147) -> ("NetworkImpairModuleID"=w143:i32)
            n49 = Variant To Data(type=T1 {"BusNumber"=0, "EvtPluginINIFilePath"=path "", "EvtParams"=[], "EvtConfig"={"UTC Time 0"=timestamp(0 s since 1904-01-01), "Nominal Frequency"=60, "Reporting Rate"=60, "Fsamp"=960, "PosSeq"=FALSE}, "Start Time"=0.0, "End Time"=0.0, "PmuImpairPluginINIFilePath"=path "", "PmuImpairParams "=[["960"], ["8.19"], ["164"]], "PmuImpairConfig"={"FilterType"="", "bPosSeq"=TRUE}, "NetImpPluginINIFilePath"=path "", "NetImpParams"=[], "FlagImpPluginINIFilePath"=path "", "FlagImpParams"=[], "EvtReportArray"=[], "EventSignalArray"=[], "ImpairReportArray"=[], "NetworkTime"=[], "PktLoss"=[], "FlagImpArray"=[], "OutputToFilePluginINIFilePath"=path "", "Output File Path"=path "", "clConfigOptions"={"TIME_BASE"=1000000, "STN"="Bus_1", "IDCODE"=0, "rdoPolRect"=enum."Rectangular", "rdoFloatInt"=enum."Float", "PHUNIT"=1000000, "rdoFreqDfreq"=enum."Float", "CHNAM"=["VA", "VB", "VC", "V+", "IA", "IB", "IC", "I+"], "chkCfg2Prefix"=TRUE}, "AppPluginINIFilePath"=path "", "AppConfig"=variant, "AppOutput"=variant} ("clBusData"), Variant=w145) -> (data=w144:T1, error out=w138:errorcluster)  [unwired: 1 in]
            n50 = Unbundle By Name(w144) -> ("NetImpPluginINIFilePath"=w135:path)
            n51 = call "LoadPluginRequest.vi"("error in (no error)"=w138, "PathToPlugin"=w135, "ModuleID"=w143) -> ("error out"=w137:errorcluster)  [unwired: 8 in]
            n52 = in-place {
              in-place-border: w135 -> [w148]
              n53 = in-place-cluster #3(w136) -> ()  [unwired: 1 out]
              n54 = in-place-cluster #3("NetImpPluginINIFilePath"=w148) -> (w134:T1)
            }
            n55 = call <userlib>:"AddError.vi"("Severity"="Abort" ("String"), "Priority"=u8 3, "ErrorArray"=w139, "error in (no error)"=w137) -> ("ErrorArray"=w140:errorcluster[])  [unwired: 6 in, 1 out]
          }
          frame "ReadNetImpairPluginPath" {
            n56 = Unbundle By Name(w163) -> ("NetworkImpairModuleID"=w162:i32)
            n57 = call "ObtainBroadcastForRegistration.vi"() -> ("error out"=w152:errorcluster, "NetImpBroadcast"=w151:T18)  [unwired: 10 in]
            n58 = register-events(error in=w152, w151) -> (reference out=w149:refnum<event-registration>, error out=w150:errorcluster)  [unwired: 1 in]
            n59 = call "ReadPathToPluginRequest.vi"("error in (no error)"=w150, "ModuleID"=w162) -> ("error out"=w153:errorcluster)  [unwired: 9 in]
            n60 = case shown="No Error" w153 {
              selector: w153 -> [w168 w176]
              tunnel: [w171 w175] -> w154
              tunnel: [w168 w176] -> w158
              tunnel: w155 -> [w167 w175]
              tunnel: w162 -> [w166 _]
              tunnel: w156 -> [w165 _]
              tunnel: w149 -> [w164 _]
              frame No Error {
                n61 = Bundle By Name(cluster=T12 {"ModuleType"=enum."PMU", "ModuleID"=0, "UsrEvtRef"=variant, "ScriptCmd"=""} ("GetBdcstData"), "UsrEvtRef"=w164, "ModuleID"=w166, "ModuleType"=ModuleType."Network", "ScriptCmd"=w165) -> (w172:T12)
                n62 = call "Enqueue.vi"("Priority (f)"=TRUE, "ErrorArray"=w167, "Data"=w172, "Msg"="GetBroadcast") -> ("ErrorArray"=w171:errorcluster[])  [unwired: 7 in]
              }
              frame Error {
              }
            }
            n63 = call <userlib>:"AddError.vi"("Severity"="Abort" ("String"), "Priority"=u8 3, "ErrorArray"=w154, "error in (no error)"=w158) -> ("ErrorArray"=w159:errorcluster[])  [unwired: 6 in, 1 out]
          }
          frame "LoadFlagImpairPlugin" {
            n64 = Unbundle By Name(w190) -> ("FlagImpairModuleID"=w186:i32)
            n65 = Variant To Data(type=T1 {"BusNumber"=0, "EvtPluginINIFilePath"=path "", "EvtParams"=[], "EvtConfig"={"UTC Time 0"=timestamp(0 s since 1904-01-01), "Nominal Frequency"=60, "Reporting Rate"=60, "Fsamp"=960, "PosSeq"=FALSE}, "Start Time"=0.0, "End Time"=0.0, "PmuImpairPluginINIFilePath"=path "", "PmuImpairParams "=[["960"], ["8.19"], ["164"]], "PmuImpairConfig"={"FilterType"="", "bPosSeq"=TRUE}, "NetImpPluginINIFilePath"=path "", "NetImpParams"=[], "FlagImpPluginINIFilePath"=path "", "FlagImpParams"=[], "EvtReportArray"=[], "EventSignalArray"=[], "ImpairReportArray"=[], "NetworkTime"=[], "PktLoss"=[], "FlagImpArray"=[], "OutputToFilePluginINIFilePath"=path "", "Output File Path"=path "", "clConfigOptions"={"TIME_BASE"=1000000, "STN"="Bus_1", "IDCODE"=0, "rdoPolRect"=enum."Rectangular", "rdoFloatInt"=enum."Float", "PHUNIT"=1000000, "rdoFreqDfreq"=enum."Float", "CHNAM"=["VA", "VB", "VC", "V+", "IA", "IB", "IC", "I+"], "chkCfg2Prefix"=TRUE}, "AppPluginINIFilePath"=path "", "AppConfig"=variant, "AppOutput"=variant} ("clBusData"), Variant=w188) -> (data=w187:T1, error out=w181:errorcluster)  [unwired: 1 in]
            n66 = Unbundle By Name(w187) -> ("FlagImpPluginINIFilePath"=w177:path)
            n67 = call "LoadPluginRequest.vi"("error in (no error)"=w181, "PathToPlugin"=w177, "ModuleID"=w186) -> ("error out"=w180:errorcluster)  [unwired: 8 in]
            n68 = in-place {
              in-place-border: w177 -> [w191]
              n69 = in-place-cluster #4(w179) -> ()  [unwired: 1 out]
              n70 = in-place-cluster #4("FlagImpPluginINIFilePath"=w191) -> (w178:T1)
            }
            n71 = call <userlib>:"AddError.vi"("Severity"="Abort" ("String"), "Priority"=u8 3, "ErrorArray"=w182, "error in (no error)"=w180) -> ("ErrorArray"=w183:errorcluster[])  [unwired: 6 in, 1 out]
          }
          frame "ReadFlagImpairPluginPath" {
            n72 = Unbundle By Name(w206) -> ("FlagImpairModuleID"=w205:i32)
            n73 = call "ObtainBroadcastForRegistration.vi"() -> ("error out"=w195:errorcluster, "FlagImpairBroadcasts"=w194:T19)  [unwired: 10 in]
            n74 = register-events(error in=w195, w194) -> (reference out=w192:refnum<event-registration>, error out=w193:errorcluster)  [unwired: 1 in]
            n75 = call "ReadPluginINIFilePathRequest.vi"("error in (no error)"=w193, "ModuleID"=w205) -> ("error out"=w196:errorcluster)  [unwired: 9 in]
            n76 = case shown="No Error" w196 {
              selector: w196 -> [w211 w219]
              tunnel: [w214 w218] -> w197
              tunnel: [w211 w219] -> w201
              tunnel: w198 -> [w210 w218]
              tunnel: w205 -> [w209 _]
              tunnel: w199 -> [w208 _]
              tunnel: w192 -> [w207 _]
              frame No Error {
                n77 = Bundle By Name(cluster=T12 {"ModuleType"=enum."PMU", "ModuleID"=0, "UsrEvtRef"=variant, "ScriptCmd"=""} ("GetBdcstData"), "UsrEvtRef"=w207, "ModuleID"=w209, "ModuleType"=ModuleType."Flag", "ScriptCmd"=w208) -> (w215:T12)
                n78 = call "Enqueue.vi"("Priority (f)"=TRUE, "ErrorArray"=w210, "Data"=w215, "Msg"="GetBroadcast") -> ("ErrorArray"=w214:errorcluster[])  [unwired: 7 in]
              }
              frame Error {
              }
            }
            n79 = call <userlib>:"AddError.vi"("Severity"="Abort" ("String"), "Priority"=u8 3, "ErrorArray"=w197, "error in (no error)"=w201) -> ("ErrorArray"=w202:errorcluster[])  [unwired: 6 in, 1 out]
          }
          frame "LoadOutputToFilePlugin" {
            n80 = Variant To Data(type=T1 {"BusNumber"=0, "EvtPluginINIFilePath"=path "", "EvtParams"=[], "EvtConfig"={"UTC Time 0"=timestamp(0 s since 1904-01-01), "Nominal Frequency"=60, "Reporting Rate"=60, "Fsamp"=960, "PosSeq"=FALSE}, "Start Time"=0.0, "End Time"=0.0, "PmuImpairPluginINIFilePath"=path "", "PmuImpairParams "=[["960"], ["8.19"], ["164"]], "PmuImpairConfig"={"FilterType"="", "bPosSeq"=TRUE}, "NetImpPluginINIFilePath"=path "", "NetImpParams"=[], "FlagImpPluginINIFilePath"=path "", "FlagImpParams"=[], "EvtReportArray"=[], "EventSignalArray"=[], "ImpairReportArray"=[], "NetworkTime"=[], "PktLoss"=[], "FlagImpArray"=[], "OutputToFilePluginINIFilePath"=path "", "Output File Path"=path "", "clConfigOptions"={"TIME_BASE"=1000000, "STN"="Bus_1", "IDCODE"=0, "rdoPolRect"=enum."Rectangular", "rdoFloatInt"=enum."Float", "PHUNIT"=1000000, "rdoFreqDfreq"=enum."Float", "CHNAM"=["VA", "VB", "VC", "V+", "IA", "IB", "IC", "I+"], "chkCfg2Prefix"=TRUE}, "AppPluginINIFilePath"=path "", "AppConfig"=variant, "AppOutput"=variant} ("clBusData"), Variant=w231) -> (data=w229:T1, error out=w227:errorcluster)  [unwired: 1 in]
            n81 = Unbundle By Name(w233) -> ("OutputToFileModuleID"=w228:i32)
            n82 = Unbundle By Name(w229) -> ("OutputToFilePluginINIFilePath"=w220:path)
            n83 = call "LoadPluginRequest.vi"("error in (no error)"=w227, "PathToPlugin"=w220, "Numeric"=w228) -> ("error out"=w222:errorcluster)  [unwired: 8 in]
            n84 = in-place {
              in-place-border: w220 -> [w234]
              n85 = in-place-cluster #5(w232) -> ()  [unwired: 1 out]
              n86 = in-place-cluster #5("OutputToFilePluginINIFilePath"=w234) -> (w226:T1)
            }
            n87 = call <userlib>:"AddError.vi"("Severity"="Abort" ("String"), "Priority"=u8 3, "ErrorArray"=w221, "error in (no error)"=w222) -> ("ErrorArray"=w223:errorcluster[])  [unwired: 6 in, 1 out]
          }
          frame "ReadOutToFilePluginPath" {
            n88 = Unbundle By Name(w248) -> ("OutputToFileModuleID"=w247:i32)
            n89 = call "ObtainBroadcastForRegistration.vi"() -> ("error out"=w237:errorcluster, "OutputToFileBroadcast"=w236:T20)  [unwired: 10 in]
            n90 = register-events(w236) -> (reference out=w235:refnum<event-registration>)  [unwired: 2 in, 1 out]
            n91 = call "ReadPathToPluginRequest.vi"("error in (no error)"=w237, "ModuleID"=w247) -> ("error out"=w238:errorcluster)  [unwired: 9 in]
            n92 = case shown="No Error" w238 {
              selector: w238 -> [w253 w261]
              tunnel: [w256 w260] -> w239
              tunnel: [w253 w261] -> w243
              tunnel: w240 -> [w252 w260]
              tunnel: w247 -> [w251 _]
              tunnel: w235 -> [w250 _]
              tunnel: w241 -> [w249 _]
              frame No Error {
                n93 = Bundle By Name(cluster=T12 {"ModuleType"=enum."PMU", "ModuleID"=0, "UsrEvtRef"=variant, "ScriptCmd"=""} ("GetBdcstData"), "UsrEvtRef"=w250, "ModuleID"=w251, "ModuleType"=ModuleType."OutToFile", "ScriptCmd"=w249) -> (w257:T12)
                n94 = call "Enqueue.vi"("Priority (f)"=TRUE, "ErrorArray"=w252, "Data"=w257, "Msg"="GetBroadcast") -> ("ErrorArray"=w256:errorcluster[])  [unwired: 7 in]
              }
              frame Error {
              }
            }
            n95 = call <userlib>:"AddError.vi"("Severity"="Abort" ("String"), "Priority"=u8 3, "ErrorArray"=w239, "error in (no error)"=w243) -> ("ErrorArray"=w244:errorcluster[])  [unwired: 6 in, 1 out]
          }
          frame "LoadAppPlugin" {
            n96 = Variant To Data(type=T1 {"BusNumber"=0, "EvtPluginINIFilePath"=path "", "EvtParams"=[], "EvtConfig"={"UTC Time 0"=timestamp(0 s since 1904-01-01), "Nominal Frequency"=60, "Reporting Rate"=60, "Fsamp"=960, "PosSeq"=FALSE}, "Start Time"=0.0, "End Time"=0.0, "PmuImpairPluginINIFilePath"=path "", "PmuImpairParams "=[["960"], ["8.19"], ["164"]], "PmuImpairConfig"={"FilterType"="", "bPosSeq"=TRUE}, "NetImpPluginINIFilePath"=path "", "NetImpParams"=[], "FlagImpPluginINIFilePath"=path "", "FlagImpParams"=[], "EvtReportArray"=[], "EventSignalArray"=[], "ImpairReportArray"=[], "NetworkTime"=[], "PktLoss"=[], "FlagImpArray"=[], "OutputToFilePluginINIFilePath"=path "", "Output File Path"=path "", "clConfigOptions"={"TIME_BASE"=1000000, "STN"="Bus_1", "IDCODE"=0, "rdoPolRect"=enum."Rectangular", "rdoFloatInt"=enum."Float", "PHUNIT"=1000000, "rdoFreqDfreq"=enum."Float", "CHNAM"=["VA", "VB", "VC", "V+", "IA", "IB", "IC", "I+"], "chkCfg2Prefix"=TRUE}, "AppPluginINIFilePath"=path "", "AppConfig"=variant, "AppOutput"=variant} ("clBusData"), Variant=w273) -> (data=w272:T1, error out=w266:errorcluster)  [unwired: 1 in]
            n97 = Unbundle By Name(w275) -> ("AppModuleID"=w271:i32)
            n98 = Unbundle By Name(w272) -> ("AppPluginINIFilePath"=w263:path)
            n99 = call "LoadPluginEvent.vi"("error in (no error)"=w266, "PathToPlugin"=w263, "ModuleID"=w271) -> ("error out"=w265:errorcluster)  [unwired: 8 in]
            n100 = in-place {
              in-place-border: w263 -> [w276]
              n101 = in-place-cluster #6(w264) -> ()  [unwired: 1 out]
              n102 = in-place-cluster #6("AppPluginINIFilePath"=w276) -> (w262:T1)
            }
            n103 = call <userlib>:"AddError.vi"("Severity"="Abort" ("String"), "Priority"=u8 3, "ErrorArray"=w267, "error in (no error)"=w265) -> ("ErrorArray"=w268:errorcluster[])  [unwired: 6 in, 1 out]
          }
          frame "ReadAppPluginPath" {
            n104 = call "ObtainBroadcastForRegistration.vi"() -> ("error out"=w279:errorcluster, "AppModuleBroadcast"=w278:T21)  [unwired: 10 in]
            n105 = Unbundle By Name(w290) -> ("AppModuleID"=w289:i32)
            n106 = register-events(w278) -> (reference out=w277:refnum<event-registration>)  [unwired: 2 in, 1 out]
            n107 = call "ReadPathToIniRequest.vi"("error in (no error)"=w279, "ModuleID"=w289) -> ("error out"=w280:errorcluster)  [unwired: 9 in]
            n108 = case shown="No Error" w280 {
              selector: w280 -> [w295 w303]
              tunnel: [w298 w302] -> w281
              tunnel: [w295 w303] -> w285
              tunnel: w282 -> [w294 w302]
              tunnel: w289 -> [w293 _]
              tunnel: w277 -> [w292 _]
              tunnel: w283 -> [w291 _]
              frame No Error {
                n109 = Bundle By Name(cluster=T12 {"ModuleType"=enum."PMU", "ModuleID"=0, "UsrEvtRef"=variant, "ScriptCmd"=""} ("GetBdcstData"), "UsrEvtRef"=w292, "ModuleID"=w293, "ModuleType"=ModuleType."App", "ScriptCmd"=w291) -> (w299:T12)
                n110 = call "Enqueue.vi"("Priority (f)"=TRUE, "ErrorArray"=w294, "Data"=w299, "Msg"="GetBroadcast") -> ("ErrorArray"=w298:errorcluster[])  [unwired: 7 in]
              }
              frame Error {
              }
            }
            n111 = call <userlib>:"AddError.vi"("Severity"="Abort" ("String"), "Priority"=u8 3, "ErrorArray"=w281, "error in (no error)"=w285) -> ("ErrorArray"=w286:errorcluster[])  [unwired: 6 in, 1 out]
          }
          frame "PopulateEvtFrontPanel" {
            n112 = Unbundle By Name(w304) -> ("EvtPluginINIFilePath"=w326:path)
            n113 = Variant To Data(type=T13 {"TestFilePathRef"=refnum, "BusNumberRef"=refnum, "NumberOfBusesRef"=refnum, "EvtTypeRef"=refnum, "EvtParamsRef"=refnum, "EvtConfigRef"=refnum, "StartTimeRef"=refnum, "EndTimeRef"=refnum, "PmuImpairTypeRef"=refnum, "PmuImpairParamsRef"=refnum, "NetImpairParamsRef"=refnum, "FlagImpairTypeRef"=refnum, "FlagImpairParamsRef"=refnum, "NetImpairTypeRef"=refnum, "OutputFileType"=refnum, "PmuImpairConfigRef"=refnum, "AppTypeRef"=refnum, "ScriptPathRef"=refnum, "ShowPanels?"=refnum} ("clFrontPanelControlRefs"), Variant=w337) -> (data=w318:T13, error out=w332:errorcluster)  [unwired: 1 in]
            n114 = Unbundle By Name(w318) -> ("EvtParamsRef"=w328:refnum<vi>, "EvtTypeRef"=w335:refnum<vi>)
            n115 = call <userlib>:"AddError.vi"("Severity"="Abort" ("String"), "Priority"=u8 3, "ErrorArray"=w331, "error in (no error)"=w332) -> ("ErrorArray"=w330:errorcluster[])  [unwired: 6 in, 1 out]
            n116 = call "GetSetFrameworkData.vi"("Set (F)"=FALSE ("Set/Get")) -> ("clFrameworkData Out"=w324:T22)  [unwired: 10 in]
            n117 = Unbundle By Name(w324) -> ("EvtINIFilePaths"=w323:path[])
            n118 = Unbundle By Name(w304) -> ("EvtParams"=w322:string[][])
            n119 = call "SetFrontPanelTypeRingFromPluginINIFile.vi"("ErrorArray In"=w330, "INIFilePath"=w326, "TypeRef In"=w335) -> ("ErrorArray Out"=w327:errorcluster[], "TypeRef Out"=w329:refnum<vi>)  [unwired: 7 in]
            n120 = call "UpdateParamsHeaders.vi"("ErrorArray In"=w327, "INIFilePaths (from Framework Data)"=w323, "ParamsRef In"=w328, "TypeRef"=w329) -> ("ErrorArray Out"=w307:errorcluster[], "ParamsRef Out"=w321:refnum<vi>)  [unwired: 6 in]
            n121 = Unbundle By Name(w304) -> ("EvtConfig"=w319:T2)
            n122 = Unbundle By Name(w318) -> ("EvtConfigRef"=w320:refnum<vi>)
            n123 = property class="Tbl (strict)"(reference=w321, "Value"=w322) -> (error out=w310:errorcluster)  [unwired: 1 in, 1 out]
            n124 = property class="Clust (strict)"(reference=w320, "Value"=w319) -> (error out=w311:errorcluster)  [unwired: 1 in, 1 out]
            n125 = Unbundle By Name(w318) -> ("StartTimeRef"=w317:refnum<vi>, "EndTimeRef"=w316:refnum<vi>)
            n126 = Unbundle By Name(w304) -> ("Start Time"=w315:dbl, "End Time"=w314:dbl)
            n127 = property class="DigNum (strict)"(reference=w317, "Value"=w315) -> (error out=w312:errorcluster)  [unwired: 1 in, 1 out]
            n128 = property class="DigNum (strict)"(reference=w316, "Value"=w314) -> (error out=w313:errorcluster)  [unwired: 1 in, 1 out]
            n129 = Merge Errors(w312, w313, w311, w310) -> (w306:errorcluster)
            n130 = call <userlib>:"AddError.vi"("Severity"="Abort" ("String"), "Priority"=u8 3, "ErrorArray"=w307, "error in (no error)"=w306) -> ("ErrorArray"=w305:errorcluster[])  [unwired: 6 in, 1 out]
          }
          frame "PopulatePmuImpairFrontPanel" {
            # "Get the path to the module's plugin's .ini file.\nThen, set the event type from the .ini file and\nupdate the Params row and column headers."
            n131 = Unbundle By Name(w341) -> ("PmuImpairConfig"=w349:T3, "PmuImpairParams"=w351:string[][], "PmuImpairPluginINIFilePath"=w357:path)
            n132 = Variant To Data(type=T13 {"TestFilePathRef"=refnum, "BusNumberRef"=refnum, "NumberOfBusesRef"=refnum, "EvtTypeRef"=refnum, "EvtParamsRef"=refnum, "EvtConfigRef"=refnum, "StartTimeRef"=refnum, "EndTimeRef"=refnum, "PmuImpairTypeRef"=refnum, "PmuImpairParamsRef"=refnum, "NetImpairParamsRef"=refnum, "FlagImpairTypeRef"=refnum, "FlagImpairParamsRef"=refnum, "NetImpairTypeRef"=refnum, "OutputFileType"=refnum, "PmuImpairConfigRef"=refnum, "AppTypeRef"=refnum, "ScriptPathRef"=refnum, "ShowPanels?"=refnum} ("clFrontPanelControlRefs"), Variant=w361) -> (data=w359:T13, error out=w348:errorcluster)  [unwired: 1 in]
            n133 = Unbundle By Name(w359) -> ("PmuImpairConfigRef"=w350:refnum<vi>, "PmuImpairTypeRef"=w358:refnum<vi>, "PmuImpairParamsRef"=w353:refnum<vi>)
            n134 = call "GetSetFrameworkData.vi"("Set (F)"=FALSE ("Set/Get")) -> ("clFrameworkData Out"=w356:T22)  [unwired: 10 in]
            n135 = Unbundle By Name(w356) -> ("PmuImpairINIFilePaths"=w354:path[])
            n136 = call "SetFrontPanelTypeRingFromPluginINIFile.vi"("ErrorArray In"=w339, "INIFilePath"=w357, "TypeRef In"=w358) -> ("ErrorArray Out"=w340:errorcluster[], "TypeRef Out"=w355:refnum<vi>)  [unwired: 7 in]
            n137 = call "UpdateParamsHeaders.vi"("ErrorArray In"=w340, "INIFilePaths (from Framework Data)"=w354, "ParamsRef In"=w353, "TypeRef"=w355) -> ("ErrorArray Out"=w338:errorcluster[], "ParamsRef Out"=w352:refnum<vi>)  [unwired: 6 in]
            n138 = property class="Tbl (strict)"(reference=w352, error in=w348, "Value"=w351) -> (error out=w347:errorcluster)  [unwired: 1 out]
            n139 = property class="Clust (strict)"(reference=w350, error in=w347, "Value"=w349) -> (error out=w342:errorcluster)  [unwired: 1 out]
            n140 = call <userlib>:"AddError.vi"("Severity"="Abort" ("String"), "Priority"=u8 3, "ErrorArray"=w338, "error in (no error)"=w342) -> ("ErrorArray"=w343:errorcluster[])  [unwired: 6 in, 1 out]
          }
          frame "PopulateNetImpairFrontPanel" {
            n141 = Unbundle By Name(w374) -> ("NetImpParams"=w379:string[][], "NetImpPluginINIFilePath"=w371:path)
            n142 = Variant To Data(type=T13 {"TestFilePathRef"=refnum, "BusNumberRef"=refnum, "NumberOfBusesRef"=refnum, "EvtTypeRef"=refnum, "EvtParamsRef"=refnum, "EvtConfigRef"=refnum, "StartTimeRef"=refnum, "EndTimeRef"=refnum, "PmuImpairTypeRef"=refnum, "PmuImpairParamsRef"=refnum, "NetImpairParamsRef"=refnum, "FlagImpairTypeRef"=refnum, "FlagImpairParamsRef"=refnum, "NetImpairTypeRef"=refnum, "OutputFileType"=refnum, "PmuImpairConfigRef"=refnum, "AppTypeRef"=refnum, "ScriptPathRef"=refnum, "ShowPanels?"=refnum} ("clFrontPanelControlRefs"), Variant=w382) -> (data=w380:T13, error out=w370:errorcluster)  [unwired: 1 in]
            n143 = call "GetSetFrameworkData.vi"("Set (F)"=FALSE) -> ("clFrameworkData Out"=w373:T22)  [unwired: 10 in]
            n144 = Unbundle By Name(w380) -> ("NetImpairParamsRef"=w364:refnum<vi>, "NetImpairTypeRef"=w372:refnum<vi>)
            n145 = Unbundle By Name(w373) -> ("NetImpairINIFilePaths"=w365:path[])
            n146 = call "SetFrontPanelTypeRingFromPluginINIFile.vi"("ErrorArray In"=w369, "INIFilePath"=w371, "TypeRef In"=w372) -> ("ErrorArray Out"=w367:errorcluster[], "TypeRef Out"=w368:refnum<vi>)  [unwired: 7 in]
            n147 = call "UpdateParamsHeaders.vi"("ErrorArray In"=w367, "INIFilePaths (from Framework Data)"=w365, "ParamsRef In"=w364, "TypeRef"=w368) -> ("ErrorArray Out"=w366:errorcluster[], "ParamsRef Out"=w363:refnum<vi>)  [unwired: 6 in]
            n148 = property class="Tbl (strict)"(reference=w363, error in=w370, "Value"=w379) -> (error out=w375:errorcluster)  [unwired: 1 out]
            n149 = call <userlib>:"AddError.vi"("Severity"="Abort" ("String"), "Priority"=u8 3, "ErrorArray"=w366, "error in (no error)"=w375) -> ("ErrorArray"=w376:errorcluster[])  [unwired: 6 in, 1 out]
          }
          frame "PopulateFlagImpairFrontPanel" {
            # "Get the path to the module's plugin's .ini file.\nThen, set the event type from the .ini file and\nupdate the Params row and column headers."
            n150 = Variant To Data(type=T13 {"TestFilePathRef"=refnum, "BusNumberRef"=refnum, "NumberOfBusesRef"=refnum, "EvtTypeRef"=refnum, "EvtParamsRef"=refnum, "EvtConfigRef"=refnum, "StartTimeRef"=refnum, "EndTimeRef"=refnum, "PmuImpairTypeRef"=refnum, "PmuImpairParamsRef"=refnum, "NetImpairParamsRef"=refnum, "FlagImpairTypeRef"=refnum, "FlagImpairParamsRef"=refnum, "NetImpairTypeRef"=refnum, "OutputFileType"=refnum, "PmuImpairConfigRef"=refnum, "AppTypeRef"=refnum, "ScriptPathRef"=refnum, "ShowPanels?"=refnum} ("clFrontPanelControlRefs"), Variant=w402) -> (data=w400:T13, error out=w391:errorcluster)  [unwired: 1 in]
            n151 = Unbundle By Name(w384) -> ("FlagImpParams"=w392:string[][], "FlagImpPluginINIFilePath"=w398:path)
            n152 = Unbundle By Name(w400) -> ("FlagImpairTypeRef"=w399:refnum<vi>, "FlagImpairParamsRef"=w394:refnum<vi>)
            n153 = call "GetSetFrameworkData.vi"("Set (F)"=FALSE ("Set/Get")) -> ("clFrameworkData Out"=w397:T22)  [unwired: 10 in]
            n154 = Unbundle By Name(w397) -> ("FlagImpairINIFilePaths"=w395:path[])
            n155 = call "SetFrontPanelTypeRingFromPluginINIFile.vi"("INIFilePath"=w398, "TypeRef In"=w399) -> ("TypeRef Out"=w396:refnum<vi>)  [unwired: 8 in, 1 out]
            n156 = call "UpdateParamsHeaders.vi"("INIFilePaths (from Framework Data)"=w395, "ParamsRef In"=w394, "TypeRef"=w396) -> ("ParamsRef Out"=w393:refnum<vi>)  [unwired: 7 in, 1 out]
            n157 = property class="Tbl (strict)"(reference=w393, error in=w391, "Value"=w392) -> (error out=w383:errorcluster)  [unwired: 1 out]
            n158 = call <userlib>:"AddError.vi"("Severity"="Abort" ("String"), "Priority"=u8 3, "ErrorArray"=w385, "error in (no error)"=w383) -> ("ErrorArray"=w386:errorcluster[], "error out"=w387:errorcluster)  [unwired: 6 in]
            n159 = call <vilib>:"Clear Errors.vi"("error in (no error)"=w387) -> ()  [unwired: 5 in, 2 out]
          }
          frame "PopulateAppFrontPanel" {
            n160 = Variant To Data(type=T13 {"TestFilePathRef"=refnum, "BusNumberRef"=refnum, "NumberOfBusesRef"=refnum, "EvtTypeRef"=refnum, "EvtParamsRef"=refnum, "EvtConfigRef"=refnum, "StartTimeRef"=refnum, "EndTimeRef"=refnum, "PmuImpairTypeRef"=refnum, "PmuImpairParamsRef"=refnum, "NetImpairParamsRef"=refnum, "FlagImpairTypeRef"=refnum, "FlagImpairParamsRef"=refnum, "NetImpairTypeRef"=refnum, "OutputFileType"=refnum, "PmuImpairConfigRef"=refnum, "AppTypeRef"=refnum, "ScriptPathRef"=refnum, "ShowPanels?"=refnum} ("clFrontPanelControlRefs"), Variant=w414) -> (data=w412:T13, error out=w405:errorcluster)  [unwired: 1 in]
            n161 = Unbundle By Name(w406) -> ("AppPluginINIFilePath"=w410:path)
            n162 = Unbundle By Name(w412) -> ("AppTypeRef"=w411:refnum<vi>)
            n163 = call "SetFrontPanelTypeRingFromPluginINIFile.vi"("ErrorArray In"=w404, "INIFilePath"=w410, "TypeRef In"=w411) -> ("ErrorArray Out"=w403:errorcluster[])  [unwired: 7 in, 1 out]
            n164 = call <userlib>:"AddError.vi"("Severity"="Abort" ("String"), "Priority"=u8 3, "ErrorArray"=w403, "error in (no error)"=w405) -> ("ErrorArray"=w407:errorcluster[])  [unwired: 6 in, 1 out]
          }
          frame "PopulateOutToFileFrontPanel" {
            n165 = Unbundle By Name(w418) -> ("OutputToFilePluginINIFilePath"=w422:path)
            n166 = Variant To Data(type=T13 {"TestFilePathRef"=refnum, "BusNumberRef"=refnum, "NumberOfBusesRef"=refnum, "EvtTypeRef"=refnum, "EvtParamsRef"=refnum, "EvtConfigRef"=refnum, "StartTimeRef"=refnum, "EndTimeRef"=refnum, "PmuImpairTypeRef"=refnum, "PmuImpairParamsRef"=refnum, "NetImpairParamsRef"=refnum, "FlagImpairTypeRef"=refnum, "FlagImpairParamsRef"=refnum, "NetImpairTypeRef"=refnum, "OutputFileType"=refnum, "PmuImpairConfigRef"=refnum, "AppTypeRef"=refnum, "ScriptPathRef"=refnum, "ShowPanels?"=refnum} ("clFrontPanelControlRefs"), Variant=w426) -> (data=w424:T13, error out=w417:errorcluster)  [unwired: 1 in]
            n167 = Unbundle By Name(w424) -> ("OutputFileType"=w423:refnum<vi>)
            n168 = call "SetFrontPanelTypeRingFromPluginINIFile.vi"("ErrorArray In"=w416, "INIFilePath"=w422, "TypeRef In"=w423) -> ("ErrorArray Out"=w415:errorcluster[])  [unwired: 7 in, 1 out]
            n169 = call <userlib>:"AddError.vi"("Severity"="Abort" ("String"), "Priority"=u8 3, "ErrorArray"=w415, "error in (no error)"=w417) -> ("ErrorArray"=w419:errorcluster[])  [unwired: 6 in, 1 out]
          }
          frame "StripIniPaths" {
            n170 = in-place {
              n171 = in-place-cluster #7(w428) -> ("EvtPluginINIFilePath"=w459:path, "PmuImpairPluginINIFilePath"=w461:path, "NetImpPluginINIFilePath"=w463:path, "FlagImpPluginINIFilePath"=w465:path, "OutputToFilePluginINIFilePath"=w471:path, "AppPluginINIFilePath"=w434:path)
              n172 = Strip Path(path=w471) -> (stripped path=w469:path, name=w467:string)
              n173 = Strip Path(path=w434) -> (stripped path=w430:path, name=w436:string)
              n174 = Strip Path(path=w459) -> (stripped path=w460:path, name=w442:string)
              n175 = Strip Path(path=w465) -> (stripped path=w466:path, name=w448:string)
              n176 = Strip Path(path=w461) -> (stripped path=w462:path, name=w444:string)
              n177 = Strip Path(path=w463) -> (stripped path=w464:path, name=w446:string)
              n178 = Strip Path(path=w469) -> (name=w458:string)  [unwired: 1 out]
              n179 = Strip Path(path=w430) -> (name=w433:string)  [unwired: 1 out]
              n180 = Strip Path(path=w460) -> (name=w441:string)  [unwired: 1 out]
              n181 = Strip Path(path=w466) -> (name=w447:string)  [unwired: 1 out]
              n182 = Strip Path(path=w462) -> (name=w443:string)  [unwired: 1 out]
              n183 = Strip Path(path=w464) -> (name=w445:string)  [unwired: 1 out]
              n184 = Concatenate Strings(w458, "\\" ("string"), w467) -> (w468:string)
              n185 = Concatenate Strings(w433, "\\" ("string"), w436) -> (w435:string)
              n186 = Concatenate Strings(w445, "\\" ("string"), w446) -> (w454:string)
              n187 = Concatenate Strings(w447, "\\" ("string"), w448) -> (w455:string)
              n188 = Concatenate Strings(w443, "\\" ("string"), w444) -> (w451:string)
              n189 = Concatenate Strings(w441, "\\" ("string"), w442) -> (w450:string)
              n190 = String To Path(string=w468) -> (path=w470:path)
              n191 = String To Path(string=w435) -> (path=w432:path)
              n192 = String To Path(string=w454) -> (path=w439:path)
              n193 = String To Path(string=w455) -> (path=w440:path)
              n194 = String To Path(string=w451) -> (path=w438:path)
              n195 = String To Path(string=w450) -> (path=w437:path)
              n196 = in-place-cluster #7("EvtPluginINIFilePath"=w437, "PmuImpairPluginINIFilePath"=w438, "NetImpPluginINIFilePath"=w439, "FlagImpPluginINIFilePath"=w440, "OutputToFilePluginINIFilePath"=w470, "AppPluginINIFilePath"=w432) -> (w427:T1)
            }
          }
          frame "Aggregate" {
            n197 = call "ObtainBroadcastForRegistration.vi"() -> ("error out"=w485:errorcluster, "AppModuleBroadcast"=w484:T21)  [unwired: 10 in]
            n198 = Unbundle By Name(w486) -> ("AppModuleID"=w481:i32)
            n199 = register-events(w484) -> (reference out=w483:refnum<event-registration>)  [unwired: 2 in, 1 out]
            n200 = call "AggregateRequest.vi"("error in (no error)"=w485, "ModuleID"=w481) -> ("error out"=w482:errorcluster)  [unwired: 9 in]
            n201 = while {
              tunnel: w483 -> [w497]
              tunnel: w480 -> [w494]
              tunnel: w482 -> [w496]
              shift-right: [w489] -> w476
              shift-left: w478 -> [w491]
              tunnel: [w487] -> w477
              stop <- w488 stop-if-true
              # "Loop waits for Errors, Completion Msg, or Timeout"
              n202 = event shown="[0] <AppModuleBroadcast.StatusUpdate>: User Event" {
                selector: w497 -> [_ _ _]
                dyn-events: [_ _ _] -> w487
                timeout: 10000 -> [_ _ _]
                tunnel: w496 -> [_ _ w504]
                tunnel: [_ w499 w505] -> w490
                tunnel: w494 -> [_ _ w506]
                tunnel: [TRUE _ TRUE] -> w488
                event User Event {
                  n203 = event-data() -> ()  [unwired: 1 in, 1 out]
                }
                event User Event {
                  n204 = event-data() -> ("Data"=w500:variant)  [unwired: 1 in]
                  n205 = Variant To Data(type=T14 {"error"={"status"=FALSE, "code"=0, "source"=""}, "AdditionalInfo"=""} ("Cluster"), Variant=w500) -> (data=w501:T14)  [unwired: 1 in, 1 out]
                  n206 = Unbundle By Name(w501) -> ("error"=w499:errorcluster)
                }
                event Timeout {
                  n207 = event-data() -> ()  [unwired: 1 in, 1 out]
                  n208 = xnode "Error Ring"("parameter 0"=w506) -> ("error out"=w507:errorcluster)
                  n209 = Merge Errors(w504, w507) -> (w505:errorcluster)
                }
              }
              n210 = call <userlib>:"AddError.vi"("Severity"="Abort" ("String"), "Priority"=u8 3, "ErrorArray"=w491, "error in (no error)"=w490) -> ("ErrorArray"=w489:errorcluster[])  [unwired: 6 in, 1 out]
            }
            n211 = Unregister For Events(event registration refnum=w477) -> (error out=w475:errorcluster)  [unwired: 1 in]
            n212 = call <userlib>:"AddError.vi"("Severity"="Inform", "Priority"=u8 4, "ErrorArray"=w476, "error in (no error)"=w475) -> ("ErrorArray"=w474:errorcluster[])  [unwired: 6 in, 1 out]
          }
          frame "CalcAppOutput" {
            n213 = property class="Bus.lvclass"(reference=w522) -> ("Accessors:AppModuleID"=w521:i32)  [unwired: 1 in, 2 out]
            n214 = call "CalcAppOutputRequest.vi"("ModuleID"=w521) -> ("error out"=w519:errorcluster)  [unwired: 10 in]
            n215 = call <userlib>:"AddError.vi"("Severity"="Abort", "Priority"=u8 3, "ErrorArray"=w520, "error in (no error)"=w519) -> ("ErrorArray"=w515:errorcluster[])  [unwired: 6 in, 1 out]
          }
          frame "GetAppOutput" {
            n216 = call "ObtainBroadcastForRegistration.vi"() -> ("error out"=w535:errorcluster, "AppModuleBroadcast"=w534:T21)  [unwired: 10 in]
            n217 = Unbundle By Name(w536) -> ("AppModuleID"=w525:i32)
            n218 = register-events(w534) -> (reference out=w526:refnum<event-registration>)  [unwired: 2 in, 1 out]
            n219 = call "GetAppOutputRequest.vi"("error in (no error)"=w535, "ModuleID"=w525) -> ("error out"=w527:errorcluster)  [unwired: 9 in]
            n220 = case shown="No Error" w527 {
              selector: w527 -> [w541 w549]
              tunnel: [w544 w548] -> w528
              tunnel: [w541 w549] -> w523
              tunnel: w529 -> [w540 w548]
              tunnel: w525 -> [w539 _]
              tunnel: w526 -> [w538 _]
              tunnel: w524 -> [w537 _]
              frame No Error {
                n221 = Bundle By Name(cluster=T12 {"ModuleType"=enum."PMU", "ModuleID"=0, "UsrEvtRef"=variant, "ScriptCmd"=""} ("GetBdcstData"), "UsrEvtRef"=w538, "ModuleID"=w539, "ModuleType"=ModuleType."App", "ScriptCmd"=w537) -> (w545:T12)
                n222 = call "Enqueue.vi"("Priority (f)"=TRUE, "ErrorArray"=w540, "Data"=w545, "Msg"="GetBroadcast") -> ("ErrorArray"=w544:errorcluster[])  [unwired: 7 in]
              }
              frame Error {
              }
            }
            n223 = call <userlib>:"AddError.vi"("Severity"="Abort" ("String"), "Priority"=u8 3, "ErrorArray"=w528, "error in (no error)"=w523) -> ("ErrorArray"=w531:errorcluster[])  [unwired: 6 in, 1 out]
          }
          frame "ReadAppInputData" {
            n224 = Unbundle By Name(w563) -> ("AppModuleID"=w562:i32)
            n225 = call "ObtainBroadcastForRegistration.vi"() -> ("error out"=w552:errorcluster, "AppModuleBroadcast"=w551:T21)  [unwired: 10 in]
            n226 = register-events(w551) -> (reference out=w550:refnum<event-registration>)  [unwired: 2 in, 1 out]
            n227 = call "ReadAppInputDataRequest.vi"("error in (no error)"=w552, "ModuleID"=w562) -> ("error out"=w553:errorcluster)  [unwired: 9 in]
            n228 = case shown="No Error" w553 {
              selector: w553 -> [w568 w576]
              tunnel: [w571 w575] -> w554
              tunnel: [w568 w576] -> w558
              tunnel: w555 -> [w567 w575]
              tunnel: w562 -> [w566 _]
              tunnel: w550 -> [w565 _]
              tunnel: w556 -> [w564 _]
              frame No Error {
                n229 = Bundle By Name(cluster=T12 {"ModuleType"=enum."PMU", "ModuleID"=0, "UsrEvtRef"=variant, "ScriptCmd"=""} ("GetBdcstData"), "UsrEvtRef"=w565, "ModuleID"=w566, "ModuleType"=ModuleType."App", "ScriptCmd"=w564) -> (w572:T12)
                n230 = call "Enqueue.vi"("Priority (f)"=TRUE, "ErrorArray"=w567, "Data"=w572, "Msg"="GetBroadcast") -> ("ErrorArray"=w571:errorcluster[])  [unwired: 7 in]
              }
              frame Error {
              }
            }
            n231 = call <userlib>:"AddError.vi"("Severity"="Abort" ("String"), "Priority"=u8 3, "ErrorArray"=w554, "error in (no error)"=w558) -> ("ErrorArray"=w559:errorcluster[])  [unwired: 6 in, 1 out]
          }
          frame "WriteAppConfig" {
            # "Write the App Config XML to the App"
            n232 = Variant To Data(type=T1 {"BusNumber"=0, "EvtPluginINIFilePath"=path "", "EvtParams"=[], "EvtConfig"={"UTC Time 0"=timestamp(0 s since 1904-01-01), "Nominal Frequency"=60, "Reporting Rate"=60, "Fsamp"=960, "PosSeq"=FALSE}, "Start Time"=0.0, "End Time"=0.0, "PmuImpairPluginINIFilePath"=path "", "PmuImpairParams "=[["960"], ["8.19"], ["164"]], "PmuImpairConfig"={"FilterType"="", "bPosSeq"=TRUE}, "NetImpPluginINIFilePath"=path "", "NetImpParams"=[], "FlagImpPluginINIFilePath"=path "", "FlagImpParams"=[], "EvtReportArray"=[], "EventSignalArray"=[], "ImpairReportArray"=[], "NetworkTime"=[], "PktLoss"=[], "FlagImpArray"=[], "OutputToFilePluginINIFilePath"=path "", "Output File Path"=path "", "clConfigOptions"={"TIME_BASE"=1000000, "STN"="Bus_1", "IDCODE"=0, "rdoPolRect"=enum."Rectangular", "rdoFloatInt"=enum."Float", "PHUNIT"=1000000, "rdoFreqDfreq"=enum."Float", "CHNAM"=["VA", "VB", "VC", "V+", "IA", "IB", "IC", "I+"], "chkCfg2Prefix"=TRUE}, "AppPluginINIFilePath"=path "", "AppConfig"=variant, "AppOutput"=variant} ("clBusData"), Variant=w593) -> (data=w592:T1, error out=w580:errorcluster)  [unwired: 1 in]
            n233 = Unbundle By Name(w585) -> ("AppModuleID"=w584:i32)
            n234 = Unbundle By Name(w592) -> ("AppConfig"=w577:variant)
            n235 = Variant To Data(error in=w580, type="", Variant=w577) -> (data=w581:string, error out=w579:errorcluster)
            n236 = call "WriteAppConfigRequest.vi"("error in (no error)"=w579, "AppConfigXML"=w581, "ModuleID"=w584) -> ("error out"=w587:errorcluster)  [unwired: 8 in]
            n237 = in-place {
              in-place-border: w577 -> [w595]
              n238 = in-place-cluster #8(w583) -> ()  [unwired: 1 out]
              n239 = in-place-cluster #8("AppConfig"=w595) -> (w582:T1)
            }
            n240 = call <userlib>:"AddError.vi"("Severity"="Abort" ("String"), "Priority"=u8 3, "ErrorArray"=w586, "error in (no error)"=w587) -> ("ErrorArray"=w588:errorcluster[], "error out"=w589:errorcluster)  [unwired: 6 in]
            n241 = call <vilib>:"Clear Errors.vi"("error in (no error)"=w589) -> ()  [unwired: 5 in, 2 out]
          }
          frame "ReadAppConfig" {
            n242 = Unbundle By Name(w609) -> ("AppModuleID"=w608:i32)
            n243 = call "ObtainBroadcastForRegistration.vi"() -> ("error out"=w598:errorcluster, "AppModuleBroadcast"=w597:T21)  [unwired: 10 in]
            n244 = register-events(w597) -> (reference out=w596:refnum<event-registration>)  [unwired: 2 in, 1 out]
            n245 = call "ReadAppConfigRequest.vi"("error in (no error)"=w598, "ModuleID"=w608) -> ("error out"=w599:errorcluster)  [unwired: 9 in]
            n246 = case shown="No Error" w599 {
              selector: w599 -> [w614 w622]
              tunnel: [w617 w621] -> w600
              tunnel: [w614 w622] -> w604
              tunnel: w601 -> [w613 w621]
              tunnel: w608 -> [w612 _]
              tunnel: w596 -> [w611 _]
              tunnel: w602 -> [w610 _]
              frame No Error {
                n247 = Bundle By Name(cluster=T12 {"ModuleType"=enum."PMU", "ModuleID"=0, "UsrEvtRef"=variant, "ScriptCmd"=""} ("GetBdcstData"), "UsrEvtRef"=w611, "ModuleID"=w612, "ModuleType"=ModuleType."App", "ScriptCmd"=w610) -> (w618:T12)
                n248 = call "Enqueue.vi"("Priority (f)"=TRUE, "ErrorArray"=w613, "Data"=w618, "Msg"="GetBroadcast") -> ("ErrorArray"=w617:errorcluster[])  [unwired: 7 in]
              }
              frame Error {
              }
            }
            n249 = call <userlib>:"AddError.vi"("Severity"="Abort" ("String"), "Priority"=u8 3, "ErrorArray"=w600, "error in (no error)"=w604) -> ("ErrorArray"=w605:errorcluster[])  [unwired: 6 in, 1 out]
          }
          frame "ReadOutputFilePath" {
            n250 = Unbundle By Name(w636) -> ("OutputToFileModuleID"=w635:i32)
            n251 = call "ObtainBroadcastForRegistration.vi"() -> ("error out"=w625:errorcluster, "OutputToFileBroadcast"=w624:T20)  [unwired: 10 in]
            n252 = register-events(w624) -> (reference out=w623:refnum<event-registration>)  [unwired: 2 in, 1 out]
            n253 = call "ReadOutputPathRequest.vi"("error in (no error)"=w625, "ModuleID"=w635) -> ("error out"=w626:errorcluster)  [unwired: 9 in]
            n254 = case shown="No Error" w626 {
              selector: w626 -> [w641 w649]
              tunnel: [w644 w648] -> w627
              tunnel: [w641 w649] -> w631
              tunnel: w628 -> [w640 w648]
              tunnel: w635 -> [w639 _]
              tunnel: w623 -> [w638 _]
              tunnel: w629 -> [w637 _]
              frame No Error {
                n255 = Bundle By Name(cluster=T12 {"ModuleType"=enum."PMU", "ModuleID"=0, "UsrEvtRef"=variant, "ScriptCmd"=""} ("GetBdcstData"), "UsrEvtRef"=w638, "ModuleID"=w639, "ModuleType"=ModuleType."OutToFile", "ScriptCmd"=w637) -> (w645:T12)
                n256 = call "Enqueue.vi"("Priority (f)"=TRUE, "ErrorArray"=w640, "Data"=w645, "Msg"="GetBroadcast") -> ("ErrorArray"=w644:errorcluster[])  [unwired: 7 in]
              }
              frame Error {
              }
            }
            n257 = call <userlib>:"AddError.vi"("Severity"="Abort" ("String"), "Priority"=u8 3, "ErrorArray"=w627, "error in (no error)"=w631) -> ("ErrorArray"=w632:errorcluster[])  [unwired: 6 in, 1 out]
          }
          frame "WriteOutputFilePath" {
            n258 = property class="Bus.lvclass"(reference=w659) -> ("Accessors:OutputToFileModuleID"=w658:i32)  [unwired: 1 in, 2 out]
            n259 = Variant To Data(type=T1 {"BusNumber"=0, "EvtPluginINIFilePath"=path "", "EvtParams"=[], "EvtConfig"={"UTC Time 0"=timestamp(0 s since 1904-01-01), "Nominal Frequency"=60, "Reporting Rate"=60, "Fsamp"=960, "PosSeq"=FALSE}, "Start Time"=0.0, "End Time"=0.0, "PmuImpairPluginINIFilePath"=path "", "PmuImpairParams "=[["960"], ["8.19"], ["164"]], "PmuImpairConfig"={"FilterType"="", "bPosSeq"=TRUE}, "NetImpPluginINIFilePath"=path "", "NetImpParams"=[], "FlagImpPluginINIFilePath"=path "", "FlagImpParams"=[], "EvtReportArray"=[], "EventSignalArray"=[], "ImpairReportArray"=[], "NetworkTime"=[], "PktLoss"=[], "FlagImpArray"=[], "OutputToFilePluginINIFilePath"=path "", "Output File Path"=path "", "clConfigOptions"={"TIME_BASE"=1000000, "STN"="Bus_1", "IDCODE"=0, "rdoPolRect"=enum."Rectangular", "rdoFloatInt"=enum."Float", "PHUNIT"=1000000, "rdoFreqDfreq"=enum."Float", "CHNAM"=["VA", "VB", "VC", "V+", "IA", "IB", "IC", "I+"], "chkCfg2Prefix"=TRUE}, "AppPluginINIFilePath"=path "", "AppConfig"=variant, "AppOutput"=variant} ("clBusData"), Variant=w663) -> (data=w660:T1, error out=w657:errorcluster)  [unwired: 1 in]
            n260 = Unbundle By Name(w660) -> ("Output File Path"=w650:path)
            n261 = in-place {
              in-place-border: w650 -> [w664]
              n262 = in-place-cluster #9(w661) -> ()  [unwired: 1 out]
              n263 = in-place-cluster #9("Output File Path"=w664) -> (w651:T1)
            }
            n264 = call "WriteOutputPathRequest.vi"("error in (no error)"=w657, "OutPath"=w650, "ModuleID"=w658) -> ("error out"=w653:errorcluster)  [unwired: 8 in]
            n265 = call <userlib>:"AddError.vi"("Severity"="Abort" ("String"), "Priority"=u8 3, "ErrorArray"=w652, "error in (no error)"=w653) -> ("ErrorArray"=w654:errorcluster[])  [unwired: 6 in, 1 out]
          }
          frame "ReadOutToFileConfig" {
            n266 = Unbundle By Name(w678) -> ("OutputToFileModuleID"=w677:i32)
            n267 = call "ObtainBroadcastForRegistration.vi"() -> ("error out"=w667:errorcluster, "OutputToFileBroadcast"=w666:T20)  [unwired: 10 in]
            n268 = register-events(w666) -> (reference out=w665:refnum<event-registration>)  [unwired: 2 in, 1 out]
            n269 = call "ReadPmuConfigRequest.vi"("error in (no error)"=w667, "ModuleID"=w677) -> ("error out"=w668:errorcluster)  [unwired: 9 in]
            n270 = case shown="No Error" w668 {
              selector: w668 -> [w683 w691]
              tunnel: [w686 w690] -> w669
              tunnel: [w683 w691] -> w673
              tunnel: w670 -> [w682 w690]
              tunnel: w677 -> [w681 _]
              tunnel: w665 -> [w680 _]
              tunnel: w671 -> [w679 _]
              frame No Error {
                n271 = Bundle By Name(cluster=T12 {"ModuleType"=enum."PMU", "ModuleID"=0, "UsrEvtRef"=variant, "ScriptCmd"=""} ("GetBdcstData"), "UsrEvtRef"=w680, "ModuleID"=w681, "ModuleType"=ModuleType."OutToFile", "ScriptCmd"=w679) -> (w687:T12)
                n272 = call "Enqueue.vi"("Priority (f)"=TRUE, "ErrorArray"=w682, "Data"=w687, "Msg"="GetBroadcast") -> ("ErrorArray"=w686:errorcluster[])  [unwired: 7 in]
              }
              frame Error {
              }
            }
            n273 = call <userlib>:"AddError.vi"("Severity"="Abort" ("String"), "Priority"=u8 3, "ErrorArray"=w669, "error in (no error)"=w673) -> ("ErrorArray"=w674:errorcluster[])  [unwired: 6 in, 1 out]
          }
          frame "WriteEvtBusNumber" {
            # "Write the event parameters to the event module"
            n274 = Variant To Data(type=T1 {"BusNumber"=0, "EvtPluginINIFilePath"=path "", "EvtParams"=[], "EvtConfig"={"UTC Time 0"=timestamp(0 s since 1904-01-01), "Nominal Frequency"=60, "Reporting Rate"=60, "Fsamp"=960, "PosSeq"=FALSE}, "Start Time"=0.0, "End Time"=0.0, "PmuImpairPluginINIFilePath"=path "", "PmuImpairParams "=[["960"], ["8.19"], ["164"]], "PmuImpairConfig"={"FilterType"="", "bPosSeq"=TRUE}, "NetImpPluginINIFilePath"=path "", "NetImpParams"=[], "FlagImpPluginINIFilePath"=path "", "FlagImpParams"=[], "EvtReportArray"=[], "EventSignalArray"=[], "ImpairReportArray"=[], "NetworkTime"=[], "PktLoss"=[], "FlagImpArray"=[], "OutputToFilePluginINIFilePath"=path "", "Output File Path"=path "", "clConfigOptions"={"TIME_BASE"=1000000, "STN"="Bus_1", "IDCODE"=0, "rdoPolRect"=enum."Rectangular", "rdoFloatInt"=enum."Float", "PHUNIT"=1000000, "rdoFreqDfreq"=enum."Float", "CHNAM"=["VA", "VB", "VC", "V+", "IA", "IB", "IC", "I+"], "chkCfg2Prefix"=TRUE}, "AppPluginINIFilePath"=path "", "AppConfig"=variant, "AppOutput"=variant} ("clBusData"), Variant=w698) -> (data=w696:T1, error out=w695:errorcluster)  [unwired: 1 in]
            n275 = Unbundle By Name(w700) -> ("EventModuleID"=w699:i32)
            n276 = Unbundle By Name(w696) -> ("BusNumber"=w693:u8)
            n277 = call "WriteBusNumberRequest.vi"("error in (no error)"=w695, "BusNumber"=w693, "ModuleID"=w699) -> ("error out"=w702:errorcluster)  [unwired: 8 in]
            n278 = in-place {
              in-place-border: w693 -> [w706]
              n279 = in-place-cluster #10(w694) -> ()  [unwired: 1 out]
              n280 = in-place-cluster #10("BusNumber"=w706) -> (w692:T1)
            }
            n281 = call <userlib>:"AddError.vi"("Severity"="Abort" ("String"), "Priority"=u8 3, "ErrorArray"=w701, "error in (no error)"=w702) -> ("ErrorArray"=w703:errorcluster[])  [unwired: 6 in, 1 out]
          }
          frame "ReadEvtBusNumber" {
            n282 = call "ObtainBroadcastForRegistration.vi"() -> ("error out"=w713:errorcluster, "EventBroadcast"=w722:T16)  [unwired: 10 in]
            n283 = Unbundle By Name(w721) -> ("EventModuleID"=w709:i32)
            n284 = register-events(error in=w713, w722) -> (reference out=w710:refnum<event-registration>, error out=w712:errorcluster)  [unwired: 1 in]
            n285 = call "ReadBusNumberRequest.vi"("error in (no error)"=w712, "ModuleID"=w709) -> ("error out"=w711:errorcluster)  [unwired: 9 in]
            n286 = case shown="No Error" w711 {
              selector: w711 -> [w727 w735]
              tunnel: [w730 w734] -> w714
              tunnel: [w727 w735] -> w707
              tunnel: w715 -> [w726 w734]
              tunnel: w710 -> [w725 _]
              tunnel: w709 -> [w724 _]
              tunnel: w708 -> [w723 _]
              frame No Error {
                n287 = Bundle By Name(cluster=T12 {"ModuleType"=enum."PMU", "ModuleID"=0, "UsrEvtRef"=variant, "ScriptCmd"=""} ("GetBdcstData"), "UsrEvtRef"=w725, "ModuleID"=w724, "ModuleType"=ModuleType."Event", "ScriptCmd"=w723) -> (w731:T12)
                n288 = call "Enqueue.vi"("Priority (f)"=TRUE, "ErrorArray"=w726, "Data"=w731, "Msg"="GetBroadcast") -> ("ErrorArray"=w730:errorcluster[])  [unwired: 7 in]
              }
              frame Error {
              }
            }
            n289 = call <userlib>:"AddError.vi"("Severity"="Abort" ("String"), "Priority"=u8 3, "ErrorArray"=w714, "error in (no error)"=w707) -> ("ErrorArray"=w717:errorcluster[], "error out"=w718:errorcluster)  [unwired: 6 in]
            n290 = call <vilib>:"Clear Errors.vi"("error in (no error)"=w718) -> ()  [unwired: 5 in, 2 out]
          }
          frame "WriteEvtParams" {
            # "Write the event parameters to the event module"
            n291 = Variant To Data(type=T1 {"BusNumber"=0, "EvtPluginINIFilePath"=path "", "EvtParams"=[], "EvtConfig"={"UTC Time 0"=timestamp(0 s since 1904-01-01), "Nominal Frequency"=60, "Reporting Rate"=60, "Fsamp"=960, "PosSeq"=FALSE}, "Start Time"=0.0, "End Time"=0.0, "PmuImpairPluginINIFilePath"=path "", "PmuImpairParams "=[["960"], ["8.19"], ["164"]], "PmuImpairConfig"={"FilterType"="", "bPosSeq"=TRUE}, "NetImpPluginINIFilePath"=path "", "NetImpParams"=[], "FlagImpPluginINIFilePath"=path "", "FlagImpParams"=[], "EvtReportArray"=[], "EventSignalArray"=[], "ImpairReportArray"=[], "NetworkTime"=[], "PktLoss"=[], "FlagImpArray"=[], "OutputToFilePluginINIFilePath"=path "", "Output File Path"=path "", "clConfigOptions"={"TIME_BASE"=1000000, "STN"="Bus_1", "IDCODE"=0, "rdoPolRect"=enum."Rectangular", "rdoFloatInt"=enum."Float", "PHUNIT"=1000000, "rdoFreqDfreq"=enum."Float", "CHNAM"=["VA", "VB", "VC", "V+", "IA", "IB", "IC", "I+"], "chkCfg2Prefix"=TRUE}, "AppPluginINIFilePath"=path "", "AppConfig"=variant, "AppOutput"=variant} ("clBusData"), Variant=w750) -> (data=w749:T1, error out=w739:errorcluster)  [unwired: 1 in]
            n292 = Unbundle By Name(w741) -> ("EventModuleID"=w740:i32)
            n293 = Unbundle By Name(w749) -> ("EvtParams"=w738:string[][])
            n294 = call "2DstrTableTodblArray.vi"("strTable"=w738) -> ("dbl2DArray"=w748:dbl[][])  [unwired: 10 in]
            n295 = call "WriteEvtParamsRequest.vi"("error in (no error)"=w739, "EvtParams"=w748, "ModuleID"=w740) -> ("error out"=w743:errorcluster)  [unwired: 8 in]
            n296 = in-place {
              in-place-border: w738 -> [w752]
              n297 = in-place-cluster #11(w737) -> ()  [unwired: 1 out]
              n298 = in-place-cluster #11("EvtParams"=w752) -> (w736:T1)
            }
            n299 = call <userlib>:"AddError.vi"("Severity"="Abort" ("String"), "Priority"=u8 3, "ErrorArray"=w742, "error in (no error)"=w743) -> ("ErrorArray"=w744:errorcluster[], "error out"=w745:errorcluster)  [unwired: 6 in]
            n300 = call <vilib>:"Clear Errors.vi"("error in (no error)"=w745) -> ()  [unwired: 5 in, 2 out]
          }
          frame "ReadEvtParams" {
            n301 = call "ObtainBroadcastForRegistration.vi"() -> ("error out"=w759:errorcluster, "EventBroadcast"=w768:T16)  [unwired: 10 in]
            n302 = Unbundle By Name(w767) -> ("EventModuleID"=w755:i32)
            n303 = register-events(error in=w759, w768) -> (reference out=w756:refnum<event-registration>, error out=w758:errorcluster)  [unwired: 1 in]
            n304 = call "ReadEvtParamsRequest.vi"("error in (no error)"=w758, "ModuleID"=w755) -> ("error out"=w757:errorcluster)  [unwired: 9 in]
            n305 = case shown="No Error" w757 {
              selector: w757 -> [w773 w781]
              tunnel: [w776 w780] -> w760
              tunnel: [w773 w781] -> w753
              tunnel: w761 -> [w772 w780]
              tunnel: w756 -> [w771 _]
              tunnel: w755 -> [w770 _]
              tunnel: w754 -> [w769 _]
              frame No Error {
                n306 = Bundle By Name(cluster=T12 {"ModuleType"=enum."PMU", "ModuleID"=0, "UsrEvtRef"=variant, "ScriptCmd"=""} ("GetBdcstData"), "UsrEvtRef"=w771, "ModuleID"=w770, "ModuleType"=ModuleType."Event", "ScriptCmd"=w769) -> (w777:T12)
                n307 = call "Enqueue.vi"("Priority (f)"=TRUE, "ErrorArray"=w772, "Data"=w777, "Msg"="GetBroadcast") -> ("ErrorArray"=w776:errorcluster[])  [unwired: 7 in]
              }
              frame Error {
              }
            }
            n308 = call <userlib>:"AddError.vi"("Severity"="Abort" ("String"), "Priority"=u8 3, "ErrorArray"=w760, "error in (no error)"=w753) -> ("ErrorArray"=w763:errorcluster[], "error out"=w764:errorcluster)  [unwired: 6 in]
            n309 = call <vilib>:"Clear Errors.vi"("error in (no error)"=w764) -> ()  [unwired: 5 in, 2 out]
          }
          frame "WriteEvtConfig" {
            # "Write the event parameters to the event module"
            n310 = Variant To Data(type=T1 {"BusNumber"=0, "EvtPluginINIFilePath"=path "", "EvtParams"=[], "EvtConfig"={"UTC Time 0"=timestamp(0 s since 1904-01-01), "Nominal Frequency"=60, "Reporting Rate"=60, "Fsamp"=960, "PosSeq"=FALSE}, "Start Time"=0.0, "End Time"=0.0, "PmuImpairPluginINIFilePath"=path "", "PmuImpairParams "=[["960"], ["8.19"], ["164"]], "PmuImpairConfig"={"FilterType"="", "bPosSeq"=TRUE}, "NetImpPluginINIFilePath"=path "", "NetImpParams"=[], "FlagImpPluginINIFilePath"=path "", "FlagImpParams"=[], "EvtReportArray"=[], "EventSignalArray"=[], "ImpairReportArray"=[], "NetworkTime"=[], "PktLoss"=[], "FlagImpArray"=[], "OutputToFilePluginINIFilePath"=path "", "Output File Path"=path "", "clConfigOptions"={"TIME_BASE"=1000000, "STN"="Bus_1", "IDCODE"=0, "rdoPolRect"=enum."Rectangular", "rdoFloatInt"=enum."Float", "PHUNIT"=1000000, "rdoFreqDfreq"=enum."Float", "CHNAM"=["VA", "VB", "VC", "V+", "IA", "IB", "IC", "I+"], "chkCfg2Prefix"=TRUE}, "AppPluginINIFilePath"=path "", "AppConfig"=variant, "AppOutput"=variant} ("clBusData"), Variant=w803) -> (data=w785:T1, error out=w786:errorcluster)  [unwired: 1 in]
            n311 = Unbundle By Name(w805) -> ("EventModuleID"=w802:i32)
            n312 = Unbundle By Name(w785) -> ("EvtConfig.UTC Time 0"=w793:timestamp, "EvtConfig.Nominal Frequency"=w791:u16, "EvtConfig.Reporting Rate"=w789:u16, "EvtConfig.Fsamp"=w788:u32, "EvtConfig.PosSeq"=w782:bool)
            n313 = To Double Precision Float(number=w793) -> (double precision float=w792:dbl)
            n314 = To Double Precision Float(number=w791) -> (double precision float=w790:dbl)
            n315 = To Long Integer(number=w789) -> (32bit integer=w794:i32)
            n316 = Bundle By Name(cluster=T15 {"T0(UTC)"=0.0, "F0"=0.0, "Fs"=0, "FSamp"=0, "bPosSeq"=FALSE} ("clEvtConfig"), "T0(UTC)"=w792, "F0"=w790, "Fs"=w794, "FSamp"=w788, "bPosSeq"=w782) -> (w787:T15)
            n317 = call "WriteEvtConfigRequest.vi"("error in (no error)"=w786, "clEvtConfig"=w787, "ModuleID"=w802) -> ("error out"=w797:errorcluster)  [unwired: 8 in]
            n318 = in-place {
              n319 = in-place-cluster #12(w784) -> ()  [unwired: 1 out]
              n320 = in-place-cluster #13(w785) -> ("EvtConfig"=w806:T2)
              n321 = in-place-cluster #12("EvtConfig"=w806) -> (w783:T1)
              n322 = in-place-cluster #13("EvtConfig"=w806) -> ()  [unwired: 1 out]
            }
            n323 = call <userlib>:"AddError.vi"("Severity"="Abort" ("String"), "Priority"=u8 3, "ErrorArray"=w796, "error in (no error)"=w797) -> ("ErrorArray"=w798:errorcluster[], "error out"=w799:errorcluster)  [unwired: 6 in]
            n324 = call <vilib>:"Clear Errors.vi"("error in (no error)"=w799) -> ()  [unwired: 5 in, 2 out]
          }
          frame "ReadEvtConfig" {
            n325 = Unbundle By Name(w822) -> ("EventModuleID"=w810:i32)
            n326 = call "ObtainBroadcastForRegistration.vi"() -> ("error out"=w813:errorcluster, "EventBroadcast"=w821:T16)  [unwired: 10 in]
            n327 = register-events(error in=w813, w821) -> (reference out=w809:refnum<event-registration>, error out=w812:errorcluster)  [unwired: 1 in]
            n328 = call "ReadEvtConfigRequest.vi"("error in (no error)"=w812, "ModuleID"=w810) -> ("error out"=w811:errorcluster)  [unwired: 9 in]
            n329 = case shown="No Error" w811 {
              selector: w811 -> [w827 w835]
              tunnel: [w830 w834] -> w814
              tunnel: [w827 w835] -> w807
              tunnel: w815 -> [w826 w834]
              tunnel: w809 -> [w825 _]
              tunnel: w810 -> [w824 _]
              tunnel: w808 -> [w823 _]
              frame No Error {
                n330 = Bundle By Name(cluster=T12 {"ModuleType"=enum."PMU", "ModuleID"=0, "UsrEvtRef"=variant, "ScriptCmd"=""} ("GetBdcstData"), "UsrEvtRef"=w825, "ModuleID"=w824, "ModuleType"=ModuleType."Event", "ScriptCmd"=w823) -> (w831:T12)
                n331 = call "Enqueue.vi"("Priority (f)"=TRUE, "ErrorArray"=w826, "Data"=w831, "Msg"="GetBroadcast") -> ("ErrorArray"=w830:errorcluster[])  [unwired: 7 in]
              }
              frame Error {
              }
            }
            n332 = call <userlib>:"AddError.vi"("Severity"="Abort" ("String"), "Priority"=u8 3, "ErrorArray"=w814, "error in (no error)"=w807) -> ("ErrorArray"=w817:errorcluster[], "error out"=w818:errorcluster)  [unwired: 6 in]
            n333 = call <vilib>:"Clear Errors.vi"("error in (no error)"=w818) -> ()  [unwired: 5 in, 2 out]
          }
          frame "WriteEvtRptTimeArray" {
            # "The Event time array  for generating PMU reports, there is also an Event Signal Time Array which adds 2 filter delays to the beginning and end"
            n334 = Unbundle By Name(w855) -> ("EventModuleID"=w851:i32)
            n335 = Variant To Data(type=T1 {"BusNumber"=0, "EvtPluginINIFilePath"=path "", "EvtParams"=[], "EvtConfig"={"UTC Time 0"=timestamp(0 s since 1904-01-01), "Nominal Frequency"=60, "Reporting Rate"=60, "Fsamp"=960, "PosSeq"=FALSE}, "Start Time"=0.0, "End Time"=0.0, "PmuImpairPluginINIFilePath"=path "", "PmuImpairParams "=[["960"], ["8.19"], ["164"]], "PmuImpairConfig"={"FilterType"="", "bPosSeq"=TRUE}, "NetImpPluginINIFilePath"=path "", "NetImpParams"=[], "FlagImpPluginINIFilePath"=path "", "FlagImpParams"=[], "EvtReportArray"=[], "EventSignalArray"=[], "ImpairReportArray"=[], "NetworkTime"=[], "PktLoss"=[], "FlagImpArray"=[], "OutputToFilePluginINIFilePath"=path "", "Output File Path"=path "", "clConfigOptions"={"TIME_BASE"=1000000, "STN"="Bus_1", "IDCODE"=0, "rdoPolRect"=enum."Rectangular", "rdoFloatInt"=enum."Float", "PHUNIT"=1000000, "rdoFreqDfreq"=enum."Float", "CHNAM"=["VA", "VB", "VC", "V+", "IA", "IB", "IC", "I+"], "chkCfg2Prefix"=TRUE}, "AppPluginINIFilePath"=path "", "AppConfig"=variant, "AppOutput"=variant} ("clBusData"), Variant=w854) -> (data=w853:T1, error out=w850:errorcluster)  [unwired: 1 in]
            n336 = Unbundle By Name(w853) -> ("EvtConfig.Reporting Rate"=w839:u16, "End Time"=w841:dbl, "Start Time"=w840:dbl)
            n337 = Greater?(x=w841, y=w840) -> (0:w837:bool)
            n338 = Greater Than 0?(x=w839) -> (x > 0?=w836:bool)
            n339 = And(x=w837, y=w836) -> (x .and. y?=w838:bool)
            n340 = case shown="False" w838 {
              tunnel: w839 -> [w856 w880]
              tunnel: w851 -> [_ w879]
              tunnel: w850 -> [_ w877]
              tunnel: [w857 w876] -> w844
              tunnel: w841 -> [w859 w875]
              tunnel: w840 -> [w858 w874]
              tunnel: w843 -> [w860 w873]
              tunnel: [w860 w872] -> w842
              frame False {
                n341 = xnode "Error Ring"("parameter 0"=w858, "parameter 1"=w859, "parameter 2"=w856) -> ("error out"=w857:errorcluster)
              }
              frame True {
                n342 = in-place {
                  in-place-border: w875 -> [w881]
                  in-place-border: w874 -> [w882]
                  n343 = in-place-cluster #14(w873) -> ()  [unwired: 2 out]
                  n344 = in-place-cluster #14("End Time"=w881, "Start Time"=w882) -> (w872:T1)
                }
                n345 = To Double Precision Float(number=w880) -> (double precision float=w871:dbl)
                n346 = Reciprocal(x=w871) -> (1/x=w870:dbl)
                n347 = call-poly <vilib>:"Ramp Pattern.vi"("start"=w874, "end"=w875, "delta"=w870) -> ("Ramp Pattern"=w878:dbl[])  [unwired: 6 in, 2 out]
                n348 = call "WriteTimeArrayRequest.vi"("error in (no error)"=w877, "TimeArray"=w878, "ModuleID"=w879) -> ("error out"=w876:errorcluster)  [unwired: 8 in]
              }
            }
            n349 = call <userlib>:"AddError.vi"("Severity"="Abort" ("String"), "Priority"=u8 3, "ErrorArray"=w845, "error in (no error)"=w844) -> ("ErrorArray"=w846:errorcluster[], "error out"=w847:errorcluster)  [unwired: 6 in]
            n350 = call <vilib>:"Clear Errors.vi"("error in (no error)"=w847) -> ()  [unwired: 5 in, 2 out]
          }
          frame "ReadEvtTime" {
            n351 = Unbundle By Name(w897) -> ("EventModuleID"=w884:i32)
            n352 = call "ObtainBroadcastForRegistration.vi"() -> ("error out"=w891:errorcluster, "EventBroadcast"=w898:T16)  [unwired: 10 in]
            n353 = register-events(error in=w891, w898) -> (reference out=w885:refnum<event-registration>, error out=w887:errorcluster)  [unwired: 1 in]
            n354 = call "ReadTimeArrayRequest.vi"("error in (no error)"=w887, "ModuleID"=w884) -> ("error out"=w886:errorcluster)  [unwired: 9 in]
            n355 = case shown="No Error" w886 {
              selector: w886 -> [w903 w911]
              tunnel: [w906 w910] -> w889
              tunnel: [w903 w911] -> w888
              tunnel: w890 -> [w902 w910]
              tunnel: w885 -> [w901 _]
              tunnel: w884 -> [w900 _]
              tunnel: w883 -> [w899 _]
              frame No Error {
                n356 = Bundle By Name(cluster=T12 {"ModuleType"=enum."PMU", "ModuleID"=0, "UsrEvtRef"=variant, "ScriptCmd"=""} ("GetBdcstData"), "UsrEvtRef"=w901, "ModuleID"=w900, "ModuleType"=ModuleType."Event", "ScriptCmd"=w899) -> (w907:T12)
                n357 = call "Enqueue.vi"("Priority (f)"=TRUE, "ErrorArray"=w902, "Data"=w907, "Msg"="GetBroadcast") -> ("ErrorArray"=w906:errorcluster[])  [unwired: 7 in]
              }
              frame Error {
              }
            }
            n358 = call <userlib>:"AddError.vi"("Severity"="Abort" ("String"), "Priority"=u8 3, "ErrorArray"=w889, "error in (no error)"=w888) -> ("ErrorArray"=w894:errorcluster[], "error out"=w893:errorcluster)  [unwired: 6 in]
            n359 = call <vilib>:"Clear Errors.vi"("error in (no error)"=w893) -> ()  [unwired: 5 in, 2 out]
          }
          frame "GetEvtReports" {
            n360 = call "ObtainBroadcastForRegistration.vi"() -> ("error out"=w923:errorcluster, "EventBroadcast"=w924:T16)  [unwired: 10 in]
            n361 = Unbundle By Name(w925) -> ("EventModuleID"=w914:i32)
            n362 = register-events(w924) -> (reference out=w915:refnum<event-registration>)  [unwired: 2 in, 1 out]
            n363 = call "GetEvtReportsRequest.vi"("error in (no error)"=w923, "ModuleID"=w914) -> ("error out"=w916:errorcluster)  [unwired: 9 in]
            n364 = case shown="No Error" w916 {
              selector: w916 -> [w930 w938]
              tunnel: [w933 w937] -> w917
              tunnel: [w930 w938] -> w912
              tunnel: w918 -> [w929 w937]
              tunnel: w915 -> [w928 _]
              tunnel: w914 -> [w927 _]
              tunnel: w913 -> [w926 _]
              frame No Error {
                n365 = Bundle By Name(cluster=T12 {"ModuleType"=enum."PMU", "ModuleID"=0, "UsrEvtRef"=variant, "ScriptCmd"=""} ("GetBdcstData"), "UsrEvtRef"=w928, "ModuleID"=w927, "ModuleType"=ModuleType."Event", "ScriptCmd"=w926) -> (w934:T12)
                n366 = call "Enqueue.vi"("Priority (f)"=TRUE, "ErrorArray"=w929, "Data"=w934, "Msg"="GetBroadcast") -> ("ErrorArray"=w933:errorcluster[])  [unwired: 7 in]
              }
              frame Error {
              }
            }
            n367 = call <userlib>:"AddError.vi"("Severity"="Abort" ("String"), "Priority"=u8 3, "ErrorArray"=w917, "error in (no error)"=w912) -> ("ErrorArray"=w920:errorcluster[])  [unwired: 6 in, 1 out]
          }
          frame "GetEvtSignal" {
            # "Note that these are being pushed into the front of the queue in the reverse order in which they will be executed"
            n368 = call "Enqueue.vi"("Priority (f)"=TRUE, "ErrorArray"=w957, "Msg"="TransferEvtTimeArrayToEvt") -> ("ErrorArray"=w956:errorcluster[])  [unwired: 8 in]
            n369 = call "Enqueue.vi"("Priority (f)"=TRUE, "ErrorArray"=w956, "Msg"="AquireEvtSignal") -> ("ErrorArray"=w952:errorcluster[])  [unwired: 8 in]
            n370 = call "Enqueue.vi"("Priority (f)"=TRUE, "ErrorArray"=w952, "Msg"="WriteEvtSigTimeArray") -> ("ErrorArray"=w948:errorcluster[])  [unwired: 8 in]
            n371 = call "Enqueue.vi"("Priority (f)"=TRUE, "ErrorArray"=w948, "Msg"="ReadEvtTime") -> ("ErrorArray"=w945:errorcluster[])  [unwired: 8 in]
            n372 = call "Enqueue.vi"("Priority (f)"=TRUE, "ErrorArray"=w945, "Msg"="ReadPmuImpairParams") -> ("ErrorArray"=w942:errorcluster[])  [unwired: 8 in]
            n373 = call "Enqueue.vi"("Priority (f)"=TRUE, "ErrorArray"=w942, "Msg"="ReadEvtConfig") -> ("ErrorArray"=w940:errorcluster[])  [unwired: 8 in]
          }
          frame "WriteEvtSigTimeArray" {
            # "Assumes all this has been read back from the event and PMU Impair modules\nSo before calling this, be sure to call the following:\nReadEvtConfig, ReadEvtTime, ReadPmuImpairParams.\n\nAfter getting the event signal, be sure to call RefreshEvtSTimeArray to replace the signal time array with the event reports time array"
            # "The Event time array  for generating Event signal and extends the time array by 2 filter periods at each end, There is also an Event Report Time Array."
            n374 = Unbundle By Name(w983) -> ("EventModuleID"=w979:i32)
            n375 = Unbundle By Name(w960) -> ("EvtConfig.Reporting Rate"=w982:u16, "End Time"=w966:dbl, "Start Time"=w968:dbl, "PmuImpairParams"=w971:string[][], "EvtConfig.Fsamp"=w962:u32)
            n376 = Index Array(array=w971, index (row)=1, index (col)=0 ("disabled index (col)")) -> (element=w964:string)
            n377 = Decimal String To Number(string=w964) -> (number=w963:i32)  [unwired: 2 in, 1 out]
            n378 = Compound Arithmetic op=MULTIPLY(w963, invert w962, 2.0 ("value")) -> (w961:dbl)
            n379 = Add(x=w966, y=w961) -> (x+y=w965:dbl)
            n380 = Subtract(x=w968, y=w961) -> (x-y=w967:dbl)
            n381 = To Double Precision Float(number=w982) -> (double precision float=w981:dbl)
            n382 = Reciprocal(x=w981) -> (1/x=w980:dbl)
            n383 = call-poly <vilib>:"Ramp Pattern.vi"("start"=w967, "end"=w965, "delta"=w980) -> ("Ramp Pattern"=w978:dbl[])  [unwired: 6 in, 2 out]
            n384 = call "WriteTimeArrayRequest.vi"("TimeArray"=w978, "ModuleID"=w979) -> ("error out"=w972:errorcluster)  [unwired: 9 in]
            n385 = call <userlib>:"AddError.vi"("Severity"="Abort" ("String"), "Priority"=u8 3, "ErrorArray"=w973, "error in (no error)"=w972) -> ("ErrorArray"=w974:errorcluster[], "error out"=w975:errorcluster)  [unwired: 6 in]
            n386 = call <vilib>:"Clear Errors.vi"("error in (no error)"=w975) -> ()  [unwired: 5 in, 2 out]
          }
          frame "TransferEvtTimeArrayToEvt" {
            n387 = Unbundle By Name(w990) -> ("EvtConfig.Reporting Rate"=w996:u16, "End Time"=w992:dbl, "Start Time"=w991:dbl)
            n388 = To Double Precision Float(number=w996) -> (double precision float=w995:dbl)
            n389 = Reciprocal(x=w995) -> (1/x=w994:dbl)
            n390 = call-poly <vilib>:"Ramp Pattern.vi"("start"=w991, "end"=w992, "delta"=w994) -> ("Ramp Pattern"=w993:dbl[])  [unwired: 6 in, 2 out]
            n391 = call "WriteTimeArrayRequest.vi"("TimeArray"=w993) -> ("error out"=w985:errorcluster)  [unwired: 10 in]
            n392 = call <userlib>:"AddError.vi"("Severity"="Abort" ("String"), "Priority"=u8 3, "ErrorArray"=w984, "error in (no error)"=w985) -> ("ErrorArray"=w986:errorcluster[], "error out"=w987:errorcluster)  [unwired: 6 in]
            n393 = call <vilib>:"Clear Errors.vi"("error in (no error)"=w987) -> ()  [unwired: 5 in, 2 out]
          }
          frame "AquireEvtSignal" {
            n394 = Unbundle By Name(w1010) -> ("EventModuleID"=w999:i32)
            n395 = call "ObtainBroadcastForRegistration.vi"() -> ("error out"=w1002:errorcluster, "EventBroadcast"=w1011:T16)  [unwired: 10 in]
            n396 = register-events(error in=w1002, w1011) -> (reference out=w1000:refnum<event-registration>, error out=w1001:errorcluster)  [unwired: 1 in]
            n397 = call "GetEvtSignalRequest.vi"("error in (no error)"=w1001, "ModuleID"=w999) -> ("error out"=w1003:errorcluster)  [unwired: 9 in]
            n398 = case shown="No Error" w1003 {
              selector: w1003 -> [w1016 w1024]
              tunnel: [w1019 w1023] -> w1004
              tunnel: [w1016 w1024] -> w997
              tunnel: w1005 -> [w1015 w1023]
              tunnel: w999 -> [w1014 _]
              tunnel: w998 -> [w1013 _]
              tunnel: w1000 -> [w1012 _]
              frame No Error {
                n399 = Bundle By Name(cluster=T12 {"ModuleType"=enum."PMU", "ModuleID"=0, "UsrEvtRef"=variant, "ScriptCmd"=""} ("GetBdcstData"), "UsrEvtRef"=w1012, "ModuleID"=w1014, "ModuleType"=ModuleType."Event", "ScriptCmd"=w1013) -> (w1020:T12)
                n400 = call "Enqueue.vi"("Priority (f)"=TRUE, "ErrorArray"=w1015, "Data"=w1020, "Msg"="GetBroadcast") -> ("ErrorArray"=w1019:errorcluster[])  [unwired: 7 in]
              }
              frame Error {
              }
            }
            n401 = call <userlib>:"AddError.vi"("Severity"="Abort" ("String"), "Priority"=u8 3, "ErrorArray"=w1004, "error in (no error)"=w997) -> ("ErrorArray"=w1007:errorcluster[])  [unwired: 6 in, 1 out]
          }
          frame "WritePmuImpairBusNumber" {
            # "Write the event parameters to the event module"
            n402 = Unbundle By Name(w1032) -> ("PmuImpairModuleID"=w1031:i32)
            n403 = Variant To Data(type=T1 {"BusNumber"=0, "EvtPluginINIFilePath"=path "", "EvtParams"=[], "EvtConfig"={"UTC Time 0"=timestamp(0 s since 1904-01-01), "Nominal Frequency"=60, "Reporting Rate"=60, "Fsamp"=960, "PosSeq"=FALSE}, "Start Time"=0.0, "End Time"=0.0, "PmuImpairPluginINIFilePath"=path "", "PmuImpairParams "=[["960"], ["8.19"], ["164"]], "PmuImpairConfig"={"FilterType"="", "bPosSeq"=TRUE}, "NetImpPluginINIFilePath"=path "", "NetImpParams"=[], "FlagImpPluginINIFilePath"=path "", "FlagImpParams"=[], "EvtReportArray"=[], "EventSignalArray"=[], "ImpairReportArray"=[], "NetworkTime"=[], "PktLoss"=[], "FlagImpArray"=[], "OutputToFilePluginINIFilePath"=path "", "Output File Path"=path "", "clConfigOptions"={"TIME_BASE"=1000000, "STN"="Bus_1", "IDCODE"=0, "rdoPolRect"=enum."Rectangular", "rdoFloatInt"=enum."Float", "PHUNIT"=1000000, "rdoFreqDfreq"=enum."Float", "CHNAM"=["VA", "VB", "VC", "V+", "IA", "IB", "IC", "I+"], "chkCfg2Prefix"=TRUE}, "AppPluginINIFilePath"=path "", "AppConfig"=variant, "AppOutput"=variant} ("clBusData"), Variant=w1028) -> (data=w1029:T1)  [unwired: 1 in, 1 out]
            n404 = Unbundle By Name(w1029) -> ("BusNumber"=w1026:u8)
            n405 = call "WriteBusNumberRequest.vi"("BusNumber"=w1026, "ModuleID"=w1031) -> ("error out"=w1034:errorcluster)  [unwired: 9 in]
            n406 = in-place {
              in-place-border: w1026 -> [w1039]
              n407 = in-place-cluster #15(w1027) -> ()  [unwired: 1 out]
              n408 = in-place-cluster #15("BusNumber"=w1039) -> (w1025:T1)
            }
            n409 = call <userlib>:"AddError.vi"("Severity"="Abort" ("String"), "Priority"=u8 3, "ErrorArray"=w1033, "error in (no error)"=w1034) -> ("ErrorArray"=w1035:errorcluster[], "error out"=w1036:errorcluster)  [unwired: 6 in]
            n410 = call <vilib>:"Clear Errors.vi"("error in (no error)"=w1036) -> ()  [unwired: 5 in, 2 out]
          }
          frame "ReadPmuImpairBusNumber" {
            n411 = Unbundle By Name(w1054) -> ("PmuImpairModuleID"=w1053:i32)
            n412 = call "ObtainBroadcastForRegistration.vi"() -> ("error out"=w1040:errorcluster, "ImpairBroadcast"=w1041:T17)  [unwired: 10 in]
            n413 = register-events(error in=w1040, w1041) -> (reference out=w1044:refnum<event-registration>, error out=w1043:errorcluster)  [unwired: 1 in]
            n414 = call "ReadBusNumberRequest.vi"("error in (no error)"=w1043, "ModuleID"=w1053) -> ("error out"=w1042:errorcluster)  [unwired: 9 in]
            n415 = case shown="No Error" w1042 {
              selector: w1042 -> [w1059 w1067]
              tunnel: [w1062 w1066] -> w1045
              tunnel: [w1059 w1067] -> w1047
              tunnel: w1046 -> [w1058 w1066]
              tunnel: w1053 -> [w1057 _]
              tunnel: w1048 -> [w1056 _]
              tunnel: w1044 -> [w1055 _]
              frame No Error {
                n416 = Bundle By Name(cluster=T12 {"ModuleType"=enum."PMU", "ModuleID"=0, "UsrEvtRef"=variant, "ScriptCmd"=""} ("GetBdcstData"), "UsrEvtRef"=w1055, "ModuleID"=w1057, "ModuleType"=ModuleType."PMU", "ScriptCmd"=w1056) -> (w1063:T12)
                n417 = call "Enqueue.vi"("Priority (f)"=TRUE, "ErrorArray"=w1058, "Data"=w1063, "Msg"="GetBroadcast") -> ("ErrorArray"=w1062:errorcluster[])  [unwired: 7 in]
              }
              frame Error {
              }
            }
            n418 = call <userlib>:"AddError.vi"("Severity"="Abort" ("String"), "Priority"=u8 3, "ErrorArray"=w1045, "error in (no error)"=w1047) -> ("ErrorArray"=w1049:errorcluster[])  [unwired: 6 in, 1 out]
          }
          frame "WritePMUImpairParams" {
            # "Write the event parameters to the event module"
            n419 = Variant To Data(type=T1 {"BusNumber"=0, "EvtPluginINIFilePath"=path "", "EvtParams"=[], "EvtConfig"={"UTC Time 0"=timestamp(0 s since 1904-01-01), "Nominal Frequency"=60, "Reporting Rate"=60, "Fsamp"=960, "PosSeq"=FALSE}, "Start Time"=0.0, "End Time"=0.0, "PmuImpairPluginINIFilePath"=path "", "PmuImpairParams "=[["960"], ["8.19"], ["164"]], "PmuImpairConfig"={"FilterType"="", "bPosSeq"=TRUE}, "NetImpPluginINIFilePath"=path "", "NetImpParams"=[], "FlagImpPluginINIFilePath"=path "", "FlagImpParams"=[], "EvtReportArray"=[], "EventSignalArray"=[], "ImpairReportArray"=[], "NetworkTime"=[], "PktLoss"=[], "FlagImpArray"=[], "OutputToFilePluginINIFilePath"=path "", "Output File Path"=path "", "clConfigOptions"={"TIME_BASE"=1000000, "STN"="Bus_1", "IDCODE"=0, "rdoPolRect"=enum."Rectangular", "rdoFloatInt"=enum."Float", "PHUNIT"=1000000, "rdoFreqDfreq"=enum."Float", "CHNAM"=["VA", "VB", "VC", "V+", "IA", "IB", "IC", "I+"], "chkCfg2Prefix"=TRUE}, "AppPluginINIFilePath"=path "", "AppConfig"=variant, "AppOutput"=variant} ("clBusData"), Variant=w1081) -> (data=w1080:T1, error out=w1071:errorcluster)  [unwired: 1 in]
            n420 = Unbundle By Name(w1083) -> ("PmuImpairModuleID"=w1079:i32)
            n421 = Unbundle By Name(w1080) -> ("PmuImpairParams"=w1070:string[][])
            n422 = call "2DstrTableTodblArray.vi"("strTable"=w1070) -> ("dbl2DArray"=w1072:dbl[][])  [unwired: 10 in]
            n423 = call "WriteImpairParamsRequest.vi"("error in (no error)"=w1071, "dblImpairParams"=w1072, "ModuleID"=w1079) -> ("error out"=w1074:errorcluster)  [unwired: 8 in]
            n424 = in-place {
              in-place-border: w1070 -> [w1084]
              n425 = in-place-cluster #16(w1069) -> ()  [unwired: 1 out]
              n426 = in-place-cluster #16("PmuImpairParams"=w1084) -> (w1068:T1)
            }
            n427 = call <userlib>:"AddError.vi"("Severity"="Abort" ("String"), "Priority"=u8 3, "ErrorArray"=w1073, "error in (no error)"=w1074) -> ("ErrorArray"=w1075:errorcluster[], "error out"=w1076:errorcluster)  [unwired: 6 in]
            n428 = call <vilib>:"Clear Errors.vi"("error in (no error)"=w1076) -> ()  [unwired: 5 in, 2 out]
          }
          frame "ReadPMUImpairParams" {
            n429 = Unbundle By Name(w1099) -> ("PmuImpairModuleID"=w1098:i32)
            n430 = call "ObtainBroadcastForRegistration.vi"() -> ("error out"=w1085:errorcluster, "ImpairBroadcast"=w1086:T17)  [unwired: 10 in]
            n431 = register-events(error in=w1085, w1086) -> (reference out=w1089:refnum<event-registration>, error out=w1088:errorcluster)  [unwired: 1 in]
            n432 = call "ReadImpairParamsRequest.vi"("error in (no error)"=w1088, "ModuleID"=w1098) -> ("error out"=w1087:errorcluster)  [unwired: 9 in]
            n433 = case shown="No Error" w1087 {
              selector: w1087 -> [w1104 w1112]
              tunnel: [w1107 w1111] -> w1090
              tunnel: [w1104 w1112] -> w1092
              tunnel: w1091 -> [w1103 w1111]
              tunnel: w1098 -> [w1102 _]
              tunnel: w1093 -> [w1101 _]
              tunnel: w1089 -> [w1100 _]
              frame No Error {
                n434 = Bundle By Name(cluster=T12 {"ModuleType"=enum."PMU", "ModuleID"=0, "UsrEvtRef"=variant, "ScriptCmd"=""} ("GetBdcstData"), "UsrEvtRef"=w1100, "ModuleID"=w1102, "ModuleType"=ModuleType."PMU", "ScriptCmd"=w1101) -> (w1108:T12)
                n435 = call "Enqueue.vi"("Priority (f)"=TRUE, "ErrorArray"=w1103, "Data"=w1108, "Msg"="GetBroadcast") -> ("ErrorArray"=w1107:errorcluster[])  [unwired: 7 in]
              }
              frame Error {
              }
            }
            n436 = call <userlib>:"AddError.vi"("Severity"="Abort" ("String"), "Priority"=u8 3, "ErrorArray"=w1090, "error in (no error)"=w1092) -> ("ErrorArray"=w1094:errorcluster[])  [unwired: 6 in, 1 out]
          }
          frame "WritePmuImpairEvtParams" {
            # "Write the event parameters to the event module"
            n437 = Variant To Data(type=T1 {"BusNumber"=0, "EvtPluginINIFilePath"=path "", "EvtParams"=[], "EvtConfig"={"UTC Time 0"=timestamp(0 s since 1904-01-01), "Nominal Frequency"=60, "Reporting Rate"=60, "Fsamp"=960, "PosSeq"=FALSE}, "Start Time"=0.0, "End Time"=0.0, "PmuImpairPluginINIFilePath"=path "", "PmuImpairParams "=[["960"], ["8.19"], ["164"]], "PmuImpairConfig"={"FilterType"="", "bPosSeq"=TRUE}, "NetImpPluginINIFilePath"=path "", "NetImpParams"=[], "FlagImpPluginINIFilePath"=path "", "FlagImpParams"=[], "EvtReportArray"=[], "EventSignalArray"=[], "ImpairReportArray"=[], "NetworkTime"=[], "PktLoss"=[], "FlagImpArray"=[], "OutputToFilePluginINIFilePath"=path "", "Output File Path"=path "", "clConfigOptions"={"TIME_BASE"=1000000, "STN"="Bus_1", "IDCODE"=0, "rdoPolRect"=enum."Rectangular", "rdoFloatInt"=enum."Float", "PHUNIT"=1000000, "rdoFreqDfreq"=enum."Float", "CHNAM"=["VA", "VB", "VC", "V+", "IA", "IB", "IC", "I+"], "chkCfg2Prefix"=TRUE}, "AppPluginINIFilePath"=path "", "AppConfig"=variant, "AppOutput"=variant} ("clBusData"), Variant=w1126) -> (data=w1114:T1, error out=w1117:errorcluster)  [unwired: 1 in]
            n438 = Unbundle By Name(w1128) -> ("PmuImpairModuleID"=w1125:i32)
            n439 = Unbundle By Name(w1114) -> ("EvtParams"=w1113:string[][])
            n440 = call "2DstrTableTodblArray.vi"("strTable"=w1113) -> ("dbl2DArray"=w1118:dbl[][])  [unwired: 10 in]
            n441 = call "WriteEvtParamsRequest.vi"("error in (no error)"=w1117, "EvtParams"=w1118, "ModuleID"=w1125) -> ("error out"=w1120:errorcluster)  [unwired: 8 in]
            n442 = in-place {
              in-place-border: w1113 -> [w1129]
              n443 = in-place-cluster #17(w1116) -> ()  [unwired: 1 out]
              n444 = in-place-cluster #17("EvtParams"=w1129) -> (w1115:T1)
            }
            n445 = call <userlib>:"AddError.vi"("Severity"="Abort" ("String"), "Priority"=u8 3, "ErrorArray"=w1119, "error in (no error)"=w1120) -> ("ErrorArray"=w1121:errorcluster[], "error out"=w1122:errorcluster)  [unwired: 6 in]
            n446 = call <vilib>:"Clear Errors.vi"("error in (no error)"=w1122) -> ()  [unwired: 5 in, 2 out]
          }
          frame "WritePmuImpairConfig" {
            n447 = Unbundle By Name(w1140) -> ("PmuImpairModuleID"=w1135:i32)
            n448 = Variant To Data(type=T1 {"BusNumber"=0, "EvtPluginINIFilePath"=path "", "EvtParams"=[], "EvtConfig"={"UTC Time 0"=timestamp(0 s since 1904-01-01), "Nominal Frequency"=60, "Reporting Rate"=60, "Fsamp"=960, "PosSeq"=FALSE}, "Start Time"=0.0, "End Time"=0.0, "PmuImpairPluginINIFilePath"=path "", "PmuImpairParams "=[["960"], ["8.19"], ["164"]], "PmuImpairConfig"={"FilterType"="", "bPosSeq"=TRUE}, "NetImpPluginINIFilePath"=path "", "NetImpParams"=[], "FlagImpPluginINIFilePath"=path "", "FlagImpParams"=[], "EvtReportArray"=[], "EventSignalArray"=[], "ImpairReportArray"=[], "NetworkTime"=[], "PktLoss"=[], "FlagImpArray"=[], "OutputToFilePluginINIFilePath"=path "", "Output File Path"=path "", "clConfigOptions"={"TIME_BASE"=1000000, "STN"="Bus_1", "IDCODE"=0, "rdoPolRect"=enum."Rectangular", "rdoFloatInt"=enum."Float", "PHUNIT"=1000000, "rdoFreqDfreq"=enum."Float", "CHNAM"=["VA", "VB", "VC", "V+", "IA", "IB", "IC", "I+"], "chkCfg2Prefix"=TRUE}, "AppPluginINIFilePath"=path "", "AppConfig"=variant, "AppOutput"=variant} ("clBusData"), Variant=w1138) -> (data=w1137:T1, error out=w1136:errorcluster)  [unwired: 1 in]
            n449 = Unbundle By Name(w1137) -> ("PmuImpairConfig"=w1131:T3)
            n450 = call "WriteImpairConfigRequest.vi"("error in (no error)"=w1136, "clImpairConfig"=w1131, "ModuleID"=w1135) -> ("error out"=w1134:errorcluster)  [unwired: 8 in]
            n451 = in-place {
              in-place-border: w1131 -> [w1145]
              n452 = in-place-cluster #18(w1132) -> ()  [unwired: 1 out]
              n453 = in-place-cluster #18("PmuImpairConfig"=w1145) -> (w1130:T1)
            }
            n454 = call <userlib>:"AddError.vi"("Severity"="Abort" ("String"), "Priority"=u8 3, "ErrorArray"=w1133, "error in (no error)"=w1134) -> ("ErrorArray"=w1141:errorcluster[], "error out"=w1142:errorcluster)  [unwired: 6 in]
            n455 = call <vilib>:"Clear Errors.vi"("error in (no error)"=w1142) -> ()  [unwired: 5 in, 2 out]
          }
          frame "ReadPmuImpairConfig" {
            n456 = Unbundle By Name(w1157) -> ("PmuImpairModuleID"=w1156:i32)
            n457 = disable-structure shown="Enabled" {
              disable-tunnel: w1156 -> [w1170 w1192]
              disable-tunnel: w1155 -> [w1164 w1190]
              disable-tunnel: [w1162 w1190] -> w1154
              disable-tunnel: w1149 -> [w1161 w1191]
              disable-tunnel: [w1158 w1193] -> w1148
              disable-tunnel: w1147 -> [_ w1195]
              disable-tunnel: [_ w1194] -> w1146
              frame Disabled {
                n458 = call "ObtainBroadcastForRegistration.vi"() -> ("error out"=w1165:errorcluster, "ImpairBroadcast"=w1167:T17)  [unwired: 10 in]
                n459 = register-events(w1167) -> (reference out=w1166:refnum<event-registration>)  [unwired: 2 in, 1 out]
                n460 = call "ReadImpairConfigRequest.vi"("error in (no error)"=w1165, "ModuleID"=w1170) -> ("error out"=w1168:errorcluster)  [unwired: 9 in]
                n461 = event shown="[0] <ImpairBroadcast.ImpairConfig>: User Event" {
                  selector: w1166 -> [_ _ _]
                  dyn-events: [_ _ _] -> w1160
                  timeout: 5000 -> [_ _ _]
                  tunnel: w1168 -> [w1175 _ _]
                  tunnel: [w1174 w1178 w1182] -> w1159
                  tunnel: [w1172 _ _] -> w1163
                  tunnel: w1161 -> [_ _ w1181]
                  event User Event {
                    n462 = event-data() -> ("Data"=w1176:variant)  [unwired: 1 in]
                    n463 = Variant To Data(error in=w1175, type=T3 {"FilterType"="", "bPosSeq"=TRUE} ("clImpairConfig"), Variant=w1176) -> (data=w1172:T3, error out=w1174:errorcluster)
                  }
                  event User Event {
                    n464 = event-data() -> ("Data"=w1177:variant)  [unwired: 1 in]
                    n465 = Variant To Data(type=T14 {"error"={"status"=FALSE, "code"=0, "source"=""}, "AdditionalInfo"=""} ("Cluster"), Variant=w1177) -> (data=w1179:T14)  [unwired: 1 in, 1 out]
                    n466 = Unbundle By Name(w1179) -> ("error"=w1178:errorcluster)
                  }
                  event Timeout {
                    n467 = event-data() -> ()  [unwired: 1 in, 3 out]
                    n468 = xnode "Error Ring"("parameter 0"=w1181) -> ("error out"=w1182:errorcluster)
                  }
                }
                n469 = Unregister For Events(event registration refnum=w1160, error in=w1159) -> (error out=w1158:errorcluster)
                n470 = in-place {
                  in-place-border: w1163 -> [w1171]
                  n471 = in-place-cluster #19(w1164) -> ()  [unwired: 1 out]
                  n472 = in-place-cluster #19("PmuImpairConfig"=w1171) -> (w1162:T1)
                }
              }
              frame Enabled {
                n473 = call "ObtainBroadcastForRegistration.vi"() -> ("error out"=w1199:errorcluster, "ImpairBroadcast"=w1198:T17)  [unwired: 10 in]
                n474 = register-events(error in=w1199, w1198) -> (reference out=w1200:refnum<event-registration>, error out=w1197:errorcluster)  [unwired: 1 in]
                n475 = call "ReadImpairConfigRequest.vi"("error in (no error)"=w1197, "ModuleID"=w1192) -> ("error out"=w1196:errorcluster)  [unwired: 9 in]
                n476 = case shown="No Error" w1196 {
                  selector: w1196 -> [w1205 w1213]
                  tunnel: [w1208 w1212] -> w1194
                  tunnel: [w1205 w1213] -> w1193
                  tunnel: w1195 -> [w1204 w1212]
                  tunnel: w1192 -> [w1203 _]
                  tunnel: w1191 -> [w1202 _]
                  tunnel: w1200 -> [w1201 _]
                  frame No Error {
                    n477 = Bundle By Name(cluster=T12 {"ModuleType"=enum."PMU", "ModuleID"=0, "UsrEvtRef"=variant, "ScriptCmd"=""} ("GetBdcstData"), "UsrEvtRef"=w1201, "ModuleID"=w1203, "ModuleType"=ModuleType."PMU", "ScriptCmd"=w1202) -> (w1209:T12)
                    n478 = call "Enqueue.vi"("Priority (f)"=TRUE, "ErrorArray"=w1204, "Data"=w1209, "Msg"="GetBroadcast") -> ("ErrorArray"=w1208:errorcluster[])  [unwired: 7 in]
                  }
                  frame Error {
                  }
                }
              }
            }
            n479 = call <userlib>:"AddError.vi"("Severity"="Abort" ("String"), "Priority"=u8 3, "ErrorArray"=w1146, "error in (no error)"=w1148) -> ("ErrorArray"=w1150:errorcluster[], "error out"=w1151:errorcluster)  [unwired: 6 in]
            n480 = call <vilib>:"Clear Errors.vi"("error in (no error)"=w1151) -> ()  [unwired: 5 in, 2 out]
          }
          frame "WritePmuImpairEvtConfig" {
            n481 = Unbundle By Name(w1232) -> ("PmuImpairModuleID"=w1229:i32)
            n482 = Variant To Data(type=T1 {"BusNumber"=0, "EvtPluginINIFilePath"=path "", "EvtParams"=[], "EvtConfig"={"UTC Time 0"=timestamp(0 s since 1904-01-01), "Nominal Frequency"=60, "Reporting Rate"=60, "Fsamp"=960, "PosSeq"=FALSE}, "Start Time"=0.0, "End Time"=0.0, "PmuImpairPluginINIFilePath"=path "", "PmuImpairParams "=[["960"], ["8.19"], ["164"]], "PmuImpairConfig"={"FilterType"="", "bPosSeq"=TRUE}, "NetImpPluginINIFilePath"=path "", "NetImpParams"=[], "FlagImpPluginINIFilePath"=path "", "FlagImpParams"=[], "EvtReportArray"=[], "EventSignalArray"=[], "ImpairReportArray"=[], "NetworkTime"=[], "PktLoss"=[], "FlagImpArray"=[], "OutputToFilePluginINIFilePath"=path "", "Output File Path"=path "", "clConfigOptions"={"TIME_BASE"=1000000, "STN"="Bus_1", "IDCODE"=0, "rdoPolRect"=enum."Rectangular", "rdoFloatInt"=enum."Float", "PHUNIT"=1000000, "rdoFreqDfreq"=enum."Float", "CHNAM"=["VA", "VB", "VC", "V+", "IA", "IB", "IC", "I+"], "chkCfg2Prefix"=TRUE}, "AppPluginINIFilePath"=path "", "AppConfig"=variant, "AppOutput"=variant} ("clBusData"), Variant=w1230) -> (data=w1216:T1, error out=w1217:errorcluster)  [unwired: 1 in]
            n483 = Unbundle By Name(w1216) -> ("EvtConfig.UTC Time 0"=w1224:timestamp, "EvtConfig.Nominal Frequency"=w1222:u16, "EvtConfig.Reporting Rate"=w1220:u16, "EvtConfig.Fsamp"=w1219:u32, "EvtConfig.PosSeq"=w1214:bool)
            n484 = To Double Precision Float(number=w1224) -> (double precision float=w1223:dbl)
            n485 = To Double Precision Float(number=w1222) -> (double precision float=w1221:dbl)
            n486 = To Long Integer(number=w1220) -> (32bit integer=w1225:i32)
            n487 = Bundle By Name(cluster=T15 {"T0(UTC)"=0.0, "F0"=0.0, "Fs"=0, "FSamp"=0, "bPosSeq"=FALSE} ("clEvtConfig"), "T0(UTC)"=w1223, "F0"=w1221, "Fs"=w1225, "FSamp"=w1219, "bPosSeq"=w1214) -> (w1218:T15)
            n488 = call "WriteEvtConfigRequest.vi"("error in (no error)"=w1217, "EvtConfig"=w1218, "ModuleID"=w1229) -> ("error out"=w1228:errorcluster)  [unwired: 8 in]
            n489 = call <userlib>:"AddError.vi"("Severity"="Abort" ("String"), "Priority"=u8 3, "ErrorArray"=w1227, "error in (no error)"=w1228) -> ("ErrorArray"=w1233:errorcluster[], "error out"=w1234:errorcluster)  [unwired: 6 in]
            n490 = call <vilib>:"Clear Errors.vi"("error in (no error)"=w1234) -> ()  [unwired: 5 in, 2 out]
          }
          frame "TransferEvtReportsToPmuImpair" {
            n491 = Unbundle By Name(w1245) -> ("PmuImpairModuleID"=w1243:i32)
            n492 = Unbundle By Name(w1246) -> ("EvtReportArray"=w1244:T4)
            n493 = call "WriteEvtReportsRequest.vi"("EvtReportArray"=w1244, "ModuleID"=w1243) -> ("error out"=w1238:errorcluster)  [unwired: 9 in]
            n494 = call <userlib>:"AddError.vi"("Severity"="Abort" ("String"), "Priority"=u8 3, "ErrorArray"=w1237, "error in (no error)"=w1238) -> ("ErrorArray"=w1239:errorcluster[], "error out"=w1240:errorcluster)  [unwired: 6 in]
            n495 = call <vilib>:"Clear Errors.vi"("error in (no error)"=w1240) -> ()  [unwired: 5 in, 2 out]
          }
          frame "TransferEvtReportsToOutputToFile" {
            n496 = Unbundle By Name(w1255) -> ("OutputToFileModuleID"=w1253:i32)
            n497 = Unbundle By Name(w1256) -> ("EvtReportArray"=w1254:T4)
            n498 = call "WriteEvtRptArrayRequest.vi"("EvtRptArray"=w1254, "ModuleID"=w1253) -> ("error out"=w1248:errorcluster)  [unwired: 9 in]
            n499 = call <userlib>:"AddError.vi"("Severity"="Abort" ("String"), "Priority"=u8 3, "ErrorArray"=w1247, "error in (no error)"=w1248) -> ("ErrorArray"=w1249:errorcluster[], "error out"=w1250:errorcluster)  [unwired: 6 in]
            n500 = call <vilib>:"Clear Errors.vi"("error in (no error)"=w1250) -> ()  [unwired: 5 in, 2 out]
          }
          frame "TransferPMUImpairReportsToOutputToFile" {
            n501 = Unbundle By Name(w1265) -> ("OutputToFileModuleID"=w1263:i32)
            n502 = Unbundle By Name(w1266) -> ("ImpairReportArray"=w1264:T4)
            n503 = call "WritePMUImpairRptArrayRequest.vi"("PmuImpairRptArray"=w1264, "ModuleID"=w1263) -> ("error out"=w1258:errorcluster)  [unwired: 9 in]
            n504 = call <userlib>:"AddError.vi"("Severity"="Abort" ("String"), "Priority"=u8 3, "ErrorArray"=w1257, "error in (no error)"=w1258) -> ("ErrorArray"=w1259:errorcluster[], "error out"=w1260:errorcluster)  [unwired: 6 in]
            n505 = call <vilib>:"Clear Errors.vi"("error in (no error)"=w1260) -> ()  [unwired: 5 in, 2 out]
          }
          frame "TransferPMUImpairReportsToApp" {
            n506 = Unbundle By Name(w1276) -> ("ImpairReportArray"=w1274:T4)
            n507 = Unbundle By Name(w1275) -> ("AppModuleID"=w1273:i32)
            n508 = call "WriteAppInputDataRequest.vi"("InputData"=w1274, "ModuleID"=w1273) -> ("error out"=w1268:errorcluster)  [unwired: 9 in]
            n509 = call <userlib>:"AddError.vi"("Severity"="Abort" ("String"), "Priority"=u8 3, "ErrorArray"=w1267, "error in (no error)"=w1268) -> ("ErrorArray"=w1269:errorcluster[], "error out"=w1270:errorcluster)  [unwired: 6 in]
            n510 = call <vilib>:"Clear Errors.vi"("error in (no error)"=w1270) -> ()  [unwired: 5 in, 2 out]
          }
          frame "TransferFlagsToOutputToFile" {
            n511 = Unbundle By Name(w1285) -> ("OutputToFileModuleID"=w1284:i32)
            n512 = Unbundle By Name(w1286) -> ("FlagImpArray"=w1277:T9)
            n513 = call "WriteFlagImpairArrayRequest.vi"("u32FlagImpairArray"=w1277, "ModuleID"=w1284) -> ("error out"=w1279:errorcluster)  [unwired: 9 in]
            n514 = call <userlib>:"AddError.vi"("Severity"="Abort" ("String"), "Priority"=u8 3, "ErrorArray"=w1278, "error in (no error)"=w1279) -> ("ErrorArray"=w1280:errorcluster[], "error out"=w1281:errorcluster)  [unwired: 6 in]
            n515 = call <vilib>:"Clear Errors.vi"("error in (no error)"=w1281) -> ()  [unwired: 5 in, 2 out]
          }
          frame "TransferPktDlyToOutputToFile" {
            n516 = Unbundle By Name(w1295) -> ("OutputToFileModuleID"=w1294:i32)
            n517 = Unbundle By Name(w1296) -> ("NetworkTime"=w1287:T7)
            n518 = call "WriteNetTimeArrayRequest.vi"("NetTimeArray"=w1287, "ModuleID"=w1294) -> ("error out"=w1289:errorcluster)  [unwired: 9 in]
            n519 = call <userlib>:"AddError.vi"("Severity"="Abort" ("String"), "Priority"=u8 3, "ErrorArray"=w1288, "error in (no error)"=w1289) -> ("ErrorArray"=w1290:errorcluster[], "error out"=w1291:errorcluster)  [unwired: 6 in]
            n520 = call <vilib>:"Clear Errors.vi"("error in (no error)"=w1291) -> ()  [unwired: 5 in, 2 out]
          }
          frame "TransferPtkLossToOutputToFile" {
            n521 = Unbundle By Name(w1305) -> ("OutputToFileModuleID"=w1304:i32)
            n522 = Unbundle By Name(w1306) -> ("PktLoss"=w1297:T8)
            n523 = call "WritePktLossArrayRequest.vi"("PktLossArray"=w1297, "ModuleID"=w1304) -> ("error out"=w1299:errorcluster)  [unwired: 9 in]
            n524 = call <userlib>:"AddError.vi"("Severity"="Abort" ("String"), "Priority"=u8 3, "ErrorArray"=w1298, "error in (no error)"=w1299) -> ("ErrorArray"=w1300:errorcluster[], "error out"=w1301:errorcluster)  [unwired: 6 in]
            n525 = call <vilib>:"Clear Errors.vi"("error in (no error)"=w1301) -> ()  [unwired: 5 in, 2 out]
          }
          frame "OutputErrorsToFile" {
            # "File Name:  Current Timestamp_Bus#_PMUImpairment"
            n526 = Unbundle By Name(w1321) -> ("OutputToFileModuleID"=w1320:i32)
            n527 = Get Date/Time In Seconds() -> (seconds since 1Jan1904=w1313:timestamp)
            n528 = Unbundle By Name(w1322) -> ("BusNumber"=w1309:u8)
            n529 = Format Date/Time String(time format string (%c)="%Y%m%d%H%M%S", seconds (now)=w1313) -> (date/time string=w1310:string)  [unwired: 1 in]
            n530 = Format Into String(format string="%s_Bus%d_PMUImpairment", w1310, w1309) -> (resulting string=w1308:string, error out=w1307:errorcluster)  [unwired: 2 in]
            n531 = call "OutputErrorFileRequest.vi"("error in (no error)"=w1307, "Filename"=w1308, "ModuleID"=w1320) -> ("error out"=w1315:errorcluster)  [unwired: 8 in]
            n532 = call <userlib>:"AddError.vi"("Severity"="Abort" ("String"), "Priority"=u8 3, "ErrorArray"=w1314, "error in (no error)"=w1315) -> ("ErrorArray"=w1316:errorcluster[], "error out"=w1317:errorcluster)  [unwired: 6 in]
            n533 = call <vilib>:"Clear Errors.vi"("error in (no error)"=w1317) -> ()  [unwired: 5 in, 2 out]
          }
          frame "OutputImpairedFileRequest" {
            n534 = Unbundle By Name(w1330) -> ("OutputToFileModuleID"=w1329:i32)
            n535 = call "OutputImpairFileRequest.vi"("ModuleID"=w1329) -> ("error out"=w1324:errorcluster)  [unwired: 10 in]
            n536 = call <userlib>:"AddError.vi"("Severity"="Abort" ("String"), "Priority"=u8 3, "ErrorArray"=w1323, "error in (no error)"=w1324) -> ("ErrorArray"=w1325:errorcluster[], "error out"=w1326:errorcluster)  [unwired: 6 in]
            n537 = call <vilib>:"Clear Errors.vi"("error in (no error)"=w1326) -> ()  [unwired: 5 in, 2 out]
          }
          frame "TransferEvtSignalToPmuImpair" {
            n538 = Unbundle By Name(w1340) -> ("PmuImpairModuleID"=w1339:i32)
            n539 = Unbundle By Name(w1341) -> ("EventSignalArray"=w1332:T6)
            n540 = call "WriteEvtSignalRequest.vi"("EvtSignalArray"=w1332, "ModuleID"=w1339) -> ("error out"=w1334:errorcluster)  [unwired: 9 in]
            n541 = call <userlib>:"AddError.vi"("Severity"="Abort" ("String"), "Priority"=u8 3, "ErrorArray"=w1333, "error in (no error)"=w1334) -> ("ErrorArray"=w1335:errorcluster[], "error out"=w1336:errorcluster)  [unwired: 6 in]
            n542 = call <vilib>:"Clear Errors.vi"("error in (no error)"=w1336) -> ()  [unwired: 5 in, 2 out]
          }
          frame "WriteNetImpairParams" {
            # "Write the event parameters to the event module"
            n543 = Unbundle By Name(w1357) -> ("NetworkImpairModuleID"=w1353:i32)
            n544 = Variant To Data(type=T1 {"BusNumber"=0, "EvtPluginINIFilePath"=path "", "EvtParams"=[], "EvtConfig"={"UTC Time 0"=timestamp(0 s since 1904-01-01), "Nominal Frequency"=60, "Reporting Rate"=60, "Fsamp"=960, "PosSeq"=FALSE}, "Start Time"=0.0, "End Time"=0.0, "PmuImpairPluginINIFilePath"=path "", "PmuImpairParams "=[["960"], ["8.19"], ["164"]], "PmuImpairConfig"={"FilterType"="", "bPosSeq"=TRUE}, "NetImpPluginINIFilePath"=path "", "NetImpParams"=[], "FlagImpPluginINIFilePath"=path "", "FlagImpParams"=[], "EvtReportArray"=[], "EventSignalArray"=[], "ImpairReportArray"=[], "NetworkTime"=[], "PktLoss"=[], "FlagImpArray"=[], "OutputToFilePluginINIFilePath"=path "", "Output File Path"=path "", "clConfigOptions"={"TIME_BASE"=1000000, "STN"="Bus_1", "IDCODE"=0, "rdoPolRect"=enum."Rectangular", "rdoFloatInt"=enum."Float", "PHUNIT"=1000000, "rdoFreqDfreq"=enum."Float", "CHNAM"=["VA", "VB", "VC", "V+", "IA", "IB", "IC", "I+"], "chkCfg2Prefix"=TRUE}, "AppPluginINIFilePath"=path "", "AppConfig"=variant, "AppOutput"=variant} ("clBusData"), Variant=w1355) -> (data=w1354:T1, error out=w1345:errorcluster)  [unwired: 1 in]
            n545 = Unbundle By Name(w1354) -> ("NetImpParams"=w1342:string[][])
            n546 = call "2DstrTableTodblArray.vi"("strTable"=w1342) -> ("dbl2DArray"=w1346:dbl[][])  [unwired: 10 in]
            n547 = call "WriteNetImpParamsRequest.vi"("error in (no error)"=w1345, "dblNetImpParams"=w1346, "ModuleID"=w1353) -> ("error out"=w1348:errorcluster)  [unwired: 8 in]
            n548 = in-place {
              in-place-border: w1342 -> [w1358]
              n549 = in-place-cluster #20(w1344) -> ()  [unwired: 1 out]
              n550 = in-place-cluster #20("NetImpParams"=w1358) -> (w1343:T1)
            }
            n551 = call <userlib>:"AddError.vi"("Severity"="Abort" ("String"), "Priority"=u8 3, "ErrorArray"=w1347, "error in (no error)"=w1348) -> ("ErrorArray"=w1349:errorcluster[], "error out"=w1350:errorcluster)  [unwired: 6 in]
            n552 = call <vilib>:"Clear Errors.vi"("error in (no error)"=w1350) -> ()  [unwired: 5 in, 2 out]
          }
          frame "ReadNetImpairParams" {
            n553 = Unbundle By Name(w1373) -> ("NetworkImpairModuleID"=w1360:i32)
            n554 = call "ObtainBroadcastForRegistration.vi"() -> ("error out"=w1364:errorcluster, "NetImpBroadcast"=w1374:T18)  [unwired: 10 in]
            n555 = register-events(error in=w1364, w1374) -> (reference out=w1361:refnum<event-registration>, error out=w1363:errorcluster)  [unwired: 1 in]
            n556 = call "ReadNetImpParamsRequest.vi"("error in (no error)"=w1363, "ModuleID"=w1360) -> ("error out"=w1362:errorcluster)  [unwired: 9 in]
            n557 = case shown="No Error" w1362 {
              selector: w1362 -> [w1379 w1387]
              tunnel: [w1382 w1386] -> w1366
              tunnel: [w1379 w1387] -> w1365
              tunnel: w1367 -> [w1378 w1386]
              tunnel: w1360 -> [w1377 _]
              tunnel: w1359 -> [w1376 _]
              tunnel: w1361 -> [w1375 _]
              frame No Error {
                n558 = Bundle By Name(cluster=T12 {"ModuleType"=enum."PMU", "ModuleID"=0, "UsrEvtRef"=variant, "ScriptCmd"=""} ("GetBdcstData"), "UsrEvtRef"=w1375, "ModuleID"=w1377, "ModuleType"=ModuleType."Network", "ScriptCmd"=w1376) -> (w1383:T12)
                n559 = call "Enqueue.vi"("Priority (f)"=TRUE, "ErrorArray"=w1378, "Data"=w1383, "Msg"="GetBroadcast") -> ("ErrorArray"=w1382:errorcluster[])  [unwired: 7 in]
              }
              frame Error {
              }
            }
            n560 = call <userlib>:"AddError.vi"("Severity"="Abort" ("String"), "Priority"=u8 3, "ErrorArray"=w1366, "error in (no error)"=w1365) -> ("ErrorArray"=w1369:errorcluster[], "error out"=w1370:errorcluster)  [unwired: 6 in]
            n561 = call <vilib>:"Clear Errors.vi"("error in (no error)"=w1370) -> ()  [unwired: 5 in, 2 out]
          }
          frame "TransferTimeArrayToNetImpair" {
            n562 = Unbundle By Name(w1400) -> ("NetworkImpairModuleID"=w1394:i32)
            n563 = Unbundle By Name(w1399) -> ("EvtConfig.Reporting Rate"=w1398:u16, "End Time"=w1397:dbl, "Start Time"=w1396:dbl)
            n564 = To Double Precision Float(number=w1398) -> (double precision float=w1402:dbl)
            n565 = Reciprocal(x=w1402) -> (1/x=w1401:dbl)
            n566 = call-poly <vilib>:"Ramp Pattern.vi"("start"=w1396, "end"=w1397, "delta"=w1401) -> ("Ramp Pattern"=w1395:dbl[])  [unwired: 6 in, 2 out]
            n567 = call "WriteTimeArrayRequest.vi"("TimeArray"=w1395, "Module ID"=w1394) -> ("error out"=w1388:errorcluster)  [unwired: 9 in]
            n568 = call <userlib>:"AddError.vi"("Severity"="Abort" ("String"), "Priority"=u8 3, "ErrorArray"=w1389, "error in (no error)"=w1388) -> ("ErrorArray"=w1390:errorcluster[], "error out"=w1391:errorcluster)  [unwired: 6 in]
            n569 = call <vilib>:"Clear Errors.vi"("error in (no error)"=w1391) -> ()  [unwired: 5 in, 2 out]
          }
          frame "WriteFlagImpairParams" {
            # "Write the event parameters to the event module"
            n570 = Variant To Data(type=T1 {"BusNumber"=0, "EvtPluginINIFilePath"=path "", "EvtParams"=[], "EvtConfig"={"UTC Time 0"=timestamp(0 s since 1904-01-01), "Nominal Frequency"=60, "Reporting Rate"=60, "Fsamp"=960, "PosSeq"=FALSE}, "Start Time"=0.0, "End Time"=0.0, "PmuImpairPluginINIFilePath"=path "", "PmuImpairParams "=[["960"], ["8.19"], ["164"]], "PmuImpairConfig"={"FilterType"="", "bPosSeq"=TRUE}, "NetImpPluginINIFilePath"=path "", "NetImpParams"=[], "FlagImpPluginINIFilePath"=path "", "FlagImpParams"=[], "EvtReportArray"=[], "EventSignalArray"=[], "ImpairReportArray"=[], "NetworkTime"=[], "PktLoss"=[], "FlagImpArray"=[], "OutputToFilePluginINIFilePath"=path "", "Output File Path"=path "", "clConfigOptions"={"TIME_BASE"=1000000, "STN"="Bus_1", "IDCODE"=0, "rdoPolRect"=enum."Rectangular", "rdoFloatInt"=enum."Float", "PHUNIT"=1000000, "rdoFreqDfreq"=enum."Float", "CHNAM"=["VA", "VB", "VC", "V+", "IA", "IB", "IC", "I+"], "chkCfg2Prefix"=TRUE}, "AppPluginINIFilePath"=path "", "AppConfig"=variant, "AppOutput"=variant} ("clBusData"), Variant=w1416) -> (data=w1415:T1, error out=w1406:errorcluster)  [unwired: 1 in]
            n571 = Unbundle By Name(w1418) -> ("FlagImpairModuleID"=w1414:i32)
            n572 = Unbundle By Name(w1415) -> ("FlagImpParams"=w1403:string[][])
            n573 = call "2DstrTableTodblArray.vi"("strTable"=w1403) -> ("dbl2DArray"=w1407:dbl[][])  [unwired: 10 in]
            n574 = call "WriteFlagImpairParamsRequest.vi"("error in (no error)"=w1406, "dblFlagImpairParams"=w1407, "ModuleID"=w1414) -> ("error out"=w1409:errorcluster)  [unwired: 8 in]
            n575 = in-place {
              in-place-border: w1403 -> [w1419]
              n576 = in-place-cluster #21(w1405) -> ()  [unwired: 1 out]
              n577 = in-place-cluster #21("FlagImpParams"=w1419) -> (w1404:T1)
            }
            n578 = call <userlib>:"AddError.vi"("Severity"="Abort" ("String"), "Priority"=u8 3, "ErrorArray"=w1408, "error in (no error)"=w1409) -> ("ErrorArray"=w1410:errorcluster[], "error out"=w1411:errorcluster)  [unwired: 6 in]
            n579 = call <vilib>:"Clear Errors.vi"("error in (no error)"=w1411) -> ()  [unwired: 5 in, 2 out]
          }
          frame "ReadFlagImpairParams" {
            n580 = Unbundle By Name(w1434) -> ("FlagImpairModuleID"=w1421:i32)
            n581 = call "ObtainBroadcastForRegistration.vi"() -> ("error out"=w1426:errorcluster, "FlagImpairBroadcasts"=w1435:T19)  [unwired: 10 in]
            n582 = register-events(error in=w1426, w1435) -> (reference out=w1423:refnum<event-registration>, error out=w1425:errorcluster)  [unwired: 1 in]
            n583 = call "ReadFlagImpairParamsRequest.vi"("error in (no error)"=w1425, "ModuleID"=w1421) -> ("error out"=w1424:errorcluster)  [unwired: 9 in]
            n584 = case shown="No Error" w1424 {
              selector: w1424 -> [w1440 w1448]
              tunnel: [w1443 w1447] -> w1427
              tunnel: [w1440 w1448] -> w1422
              tunnel: w1428 -> [w1439 w1447]
              tunnel: w1421 -> [w1438 _]
              tunnel: w1420 -> [w1437 _]
              tunnel: w1423 -> [w1436 _]
              frame No Error {
                n585 = Bundle By Name(cluster=T12 {"ModuleType"=enum."PMU", "ModuleID"=0, "UsrEvtRef"=variant, "ScriptCmd"=""} ("GetBdcstData"), "UsrEvtRef"=w1436, "ModuleID"=w1438, "ModuleType"=ModuleType."Flag", "ScriptCmd"=w1437) -> (w1444:T12)
                n586 = call "Enqueue.vi"("Priority (f)"=TRUE, "ErrorArray"=w1439, "Data"=w1444, "Msg"="GetBroadcast") -> ("ErrorArray"=w1443:errorcluster[])  [unwired: 7 in]
              }
              frame Error {
              }
            }
            n587 = call <userlib>:"AddError.vi"("Severity"="Abort" ("String"), "Priority"=u8 3, "ErrorArray"=w1427, "error in (no error)"=w1422) -> ("ErrorArray"=w1430:errorcluster[], "error out"=w1431:errorcluster)  [unwired: 6 in]
            n588 = call <vilib>:"Clear Errors.vi"("error in (no error)"=w1431) -> ()  [unwired: 5 in, 2 out]
          }
          frame "WritePmuConfig" {
            n589 = property class="Bus.lvclass"(reference=w1458) -> ("Accessors:PmuImpairModuleID"=w1457:i32)  [unwired: 1 in, 2 out]
            n590 = Variant To Data(type=T1 {"BusNumber"=0, "EvtPluginINIFilePath"=path "", "EvtParams"=[], "EvtConfig"={"UTC Time 0"=timestamp(0 s since 1904-01-01), "Nominal Frequency"=60, "Reporting Rate"=60, "Fsamp"=960, "PosSeq"=FALSE}, "Start Time"=0.0, "End Time"=0.0, "PmuImpairPluginINIFilePath"=path "", "PmuImpairParams "=[["960"], ["8.19"], ["164"]], "PmuImpairConfig"={"FilterType"="", "bPosSeq"=TRUE}, "NetImpPluginINIFilePath"=path "", "NetImpParams"=[], "FlagImpPluginINIFilePath"=path "", "FlagImpParams"=[], "EvtReportArray"=[], "EventSignalArray"=[], "ImpairReportArray"=[], "NetworkTime"=[], "PktLoss"=[], "FlagImpArray"=[], "OutputToFilePluginINIFilePath"=path "", "Output File Path"=path "", "clConfigOptions"={"TIME_BASE"=1000000, "STN"="Bus_1", "IDCODE"=0, "rdoPolRect"=enum."Rectangular", "rdoFloatInt"=enum."Float", "PHUNIT"=1000000, "rdoFreqDfreq"=enum."Float", "CHNAM"=["VA", "VB", "VC", "V+", "IA", "IB", "IC", "I+"], "chkCfg2Prefix"=TRUE}, "AppPluginINIFilePath"=path "", "AppConfig"=variant, "AppOutput"=variant} ("clBusData"), Variant=w1463) -> (data=w1460:T1, error out=w1456:errorcluster)  [unwired: 1 in]
            n591 = Unbundle By Name(w1460) -> ("clConfigOptions"=w1459:T10)
            n592 = in-place {
              in-place-border: w1459 -> [w1464]
              n593 = in-place-cluster #22(w1461) -> ()  [unwired: 1 out]
              n594 = in-place-cluster #22("clConfigOptions"=w1464) -> (w1449:T1)
            }
            n595 = call "WritePMUConfigRequest.vi"("error in (no error)"=w1456, "PmuConfig"=w1459, "ModuleID"=w1457) -> ("error out"=w1451:errorcluster)  [unwired: 8 in]
            n596 = call <userlib>:"AddError.vi"("Severity"="Abort" ("String"), "Priority"=u8 3, "ErrorArray"=w1450, "error in (no error)"=w1451) -> ("ErrorArray"=w1452:errorcluster[], "error out"=w1453:errorcluster)  [unwired: 6 in]
            n597 = call <vilib>:"Clear Errors.vi"("error in (no error)"=w1453) -> ()  [unwired: 5 in, 2 out]
          }
          frame "TransferEvtConfigToApp" {
            n598 = Unbundle By Name(w1473) -> ("AppModuleID"=w1471:i32)
            n599 = Unbundle By Name(w1472) -> ("EvtConfig"=w1465:T2)
            n600 = call "WriteEvtConfigRequest.vi"("InputData"=w1465, "ModuleID"=w1471) -> ("error out"=w1466:errorcluster)  [unwired: 9 in]
            n601 = call <userlib>:"AddError.vi"("Severity"="Abort", "Priority"=u8 3, "ErrorArray"=w1467, "error in (no error)"=w1466) -> ("ErrorArray"=w1470:errorcluster[])  [unwired: 6 in, 1 out]
          }
          frame "Initialize" {
            # "Error Check, the queue should be empty when this is called"
            # "The state called upon entry"
            n602 = call "ObtainSMQueue.vi"("ErrorArray"=w1485) -> ("ErrorArray"=w1478:errorcluster[], "QueRef"=w1484:T23)  [unwired: 9 in]
            n603 = Get Queue Status(queue=w1484) -> (error out=w1477:errorcluster, # elements in queue=w1482:i32)  [unwired: 2 in, 6 out]
            n604 = Equal To 0?(x=w1482) -> (x = 0?=w1476:bool)
            n605 = call <userlib>:"AddError.vi"("Severity"="Abort" ("String"), "Priority"=u8 3, "ErrorArray"=w1478, "error in (no error)"=w1477) -> ("ErrorArray"=w1475:errorcluster[], "error out"=w1479:errorcluster)  [unwired: 6 in]
            n606 = call <vilib>:"Clear Errors.vi"("error in (no error)"=w1479) -> ()  [unwired: 5 in, 2 out]
            n607 = case shown="True" w1476 {
              tunnel: [w1489 w1505] -> w1486
              tunnel: w1483 -> [_ w1504]
              tunnel: w1475 -> [w1487 w1500]
              frame False {
                # "Initialize was called with script elements still in the queue"
                n608 = xnode "Error Ring"() -> ("error out"=w1488:errorcluster)
                n609 = call <userlib>:"AddError.vi"("Severity"="Abort" ("String"), "Priority"=u8 3, "ErrorArray"=w1487, "error in (no error)"=w1488) -> ("ErrorArray"=w1489:errorcluster[], "error out"=w1490:errorcluster)  [unwired: 6 in]
                n610 = call <vilib>:"Clear Errors.vi"("error in (no error)"=w1490) -> ()  [unwired: 5 in, 2 out]
              }
              frame True {
                w1506 = string[] []
                # "Enqueue the script"
                n611 = Variant To Data(type=w1506, Variant=w1504) -> (data=w1507:string[], error out=w1498:errorcluster)  [unwired: 1 in]
                n612 = call <userlib>:"AddError.vi"("Severity"="Abort" ("String"), "Priority"=u8 3, "ErrorArray"=w1500, "error in (no error)"=w1498) -> ("ErrorArray"=w1499:errorcluster[], "error out"=w1501:errorcluster)  [unwired: 6 in]
                n613 = call <vilib>:"Clear Errors.vi"("error in (no error)"=w1501) -> ()  [unwired: 5 in, 2 out]
                n614 = for {
                  tunnel: w1507 -> [w1519] mode=indexing
                  tunnel: w1506 -> [w1518]
                  tunnel: w1499 -> [w1509]
                  tunnel: [w1508] -> w1505 mode=concatenating
                  n615 = Spreadsheet String To Array(delimiter (Tab)="," ("format string"), format string="%s", spreadsheet string=w1519, array type (2D Dbl)=w1518) -> (array=w1515:string[])
                  n616 = Split 1D Array(array=w1515, index=1) -> (first subarray=w1511:string[], second subarray=w1513:string[])
                  n617 = To Variant(anything=w1513) -> (Variant=w1512:variant)
                  n618 = Index Array(array=w1511) -> (element=w1510:string)  [unwired: 1 in]
                  n619 = call "Enqueue.vi"("ErrorArray"=w1509, "Data"=w1512, "Msg"=w1510) -> ("ErrorArray"=w1508:errorcluster[])  [unwired: 8 in]
                }
              }
            }
          }
          frame "Abort" {
            # "Note, if any cleanup is needed before stop, do it here.  \n\nOne idea would be to use the queue data to tell abort what needs to be done."
            # "Comes here if the SM is aborted by the user or a script"
            n620 = call "Enqueue.vi"("Priority (f)"=TRUE, "ErrorArray"=w1521, "Msg"="Stop") -> ("ErrorArray"=w1524:errorcluster[])  [unwired: 8 in]
          }
          frame "Stop" {
            # "Destroy the Queue"
            # "Flush the Queue"
            n621 = call "ObtainSMQueue.vi"("ErrorArray"=w1536) -> ("ErrorArray"=w1529:errorcluster[], "QueRef"=w1535:T23)  [unwired: 9 in]
            n622 = Flush Queue(queue=w1535) -> (queue out=w1534:T23, error out=w1533:errorcluster)  [unwired: 1 in, 1 out]
            n623 = Release Queue(queue=w1534, error in (no error)=w1533) -> (error out=w1527:errorcluster)  [unwired: 1 in, 2 out]
            n624 = call <userlib>:"AddError.vi"("Severity"="Abort" ("String"), "Priority"=u8 3, "ErrorArray"=w1529, "error in (no error)"=w1527) -> ("ErrorArray"=w1528:errorcluster[], "error out"=w1530:errorcluster)  [unwired: 6 in]
            n625 = To Variant(anything=w1525) -> (Variant=w1526:variant)
            n626 = call <vilib>:"Clear Errors.vi"("error in (no error)"=w1530) -> ()  [unwired: 5 in, 2 out]
          }
          frame Default {
            n627 = xnode "Error Ring"("parameter 0"=w1543) -> ("error out"=w1544:errorcluster)
            n628 = call <userlib>:"AddError.vi"("Severity"="Abort" ("String"), "Priority"=u8 3, "ErrorArray"=w1542, "error in (no error)"=w1544) -> ("ErrorArray"=w1541:errorcluster[], "error out"=w1540:errorcluster)  [unwired: 6 in]
            n629 = call <vilib>:"Clear Errors.vi"("error in (no error)"=w1540) -> ()  [unwired: 5 in, 2 out]
          }
          frame "Error" {
            n630 = Variant To Data(type=errorcluster[] [], Variant=w1562) -> (data=w1560:errorcluster[])  [unwired: 1 in, 1 out]
            n631 = call <userlib>:"ParseErrors.vi"("ErrorArray"=w1560) -> ("ErrorArray"=w1559:errorcluster[])  [unwired: 8 in, 2 out]
            n632 = for {
              tunnel: w1559 -> [w1572] mode=indexing
              tunnel: [w1564] -> w1558 mode=concatenating
              tunnel: w1555 -> [w1563]
              n633 = Unbundle By Name(w1572) -> ("source"=w1566:string)
              n634 = call <userlib>:"GeneralHandler.vi"("error in (no error)"=w1572) -> ("Severity"=w1567:string, "Stop"=w1569:bool, "Abort"=w1570:bool, "Continue"=w1571:bool)  [unwired: 7 in]
              n635 = Build Array(w1571, w1570, w1569) -> (w1568:bool[])
              n636 = Boolean Array To Number(Boolean array=w1568) -> (number=w1565:u32)
              n637 = case shown="4" w1565 {
                tunnel: w1567 -> [_ w1574 w1581 w1587]
                tunnel: [_ _ w1580 w1586] -> w1564
                tunnel: w1566 -> [_ w1573 _ _]
                tunnel: w1563 -> [_ _ _ w1585]
                frame 0, Default {
                  # "No dialogue button pressed"
                }
                frame 1 {
                  # "Continue button pressed"
                  n638 = case shown="Default" w1574 {
                    tunnel: w1573 -> [_ w1575]
                    frame Default {
                      # "Let the State machine continue."
                    }
                    frame "Log" {
                      # "TODO : this is unfinished code"
                      # "Write to log file?"
                      n639 = Get Date/Time String(want seconds? (F)=TRUE) -> (time string=w1578:string)  [unwired: 2 in, 1 out]
                      n640 = call <vilib>:"Space Constant.vi"() -> ("String"=w1577:string)
                      n641 = Concatenate Strings(w1578, w1577, w1575, "\r\n") -> ()  [unwired: 1 out]
                    }
                  }
                }
                frame 2 {
                  # "Abort Button Pressed"
                  n642 = case shown="Default" w1581 {
                    tunnel: [w1582] -> w1580
                    frame Default {
                      # "Note:  we may be able to use the queue data to tell the system if anything needs cleanup"
                      # "go to the abort state"
                      n643 = call "Enqueue.vi"("Priority (f)"=TRUE, "Msg"="Abort") -> ("ErrorArray"=w1582:errorcluster[])  [unwired: 9 in]
                    }
                  }
                }
                frame 4 {
                  # "Stop Button Pressed"
                  n644 = case shown="Default" w1587 {
                    tunnel: [w1593] -> w1586
                    tunnel: w1585 -> [w1590]
                    frame Default {
                      # "Immediatly stop the state machine and send a stop request up to the framework"
                      n645 = Unbundle By Name(w1590) -> ("BusNumber"=w1589:u8)
                      n646 = call "Enqueue.vi"("Priority (f)"=TRUE, "Msg"="Stop") -> ("ErrorArray"=w1592:errorcluster[])  [unwired: 9 in]
                      n647 = call "StopRequest.vi"("ErrorArray In"=w1592, "BusIndex"=w1589) -> ("ErrorArray Out"=w1593:errorcluster[])  [unwired: 9 in]
                    }
                  }
                }
              }
            }
            n648 = call <userlib>:"ClearErrors.vi"() -> ("ErrorArray"=w1557:errorcluster[])  [unwired: 11 in]
            n649 = Build Array (concatenate)(w1558, w1557) -> (w1556:errorcluster[])
          }
          frame "GetPmuImpairReports - unused" {
            # "This has been replaced by the bus Controller.  Gets the PMU Impaired reports from one bus"
            n650 = Unbundle By Name(w1608) -> ("PmuImpairModuleID"=w1595:i32)
            n651 = call "ObtainBroadcastForRegistration.vi"() -> ("error out"=w1602:errorcluster, "ImpairBroadcast"=w1607:T17)  [unwired: 10 in]
            n652 = register-events(error in=w1602, w1607) -> (reference out=w1596:refnum<event-registration>, error out=w1601:errorcluster)  [unwired: 1 in]
            n653 = call "GetImpairReportsRequest.vi"("error in (no error)"=w1601, "ModuleID"=w1595) -> ("error out"=w1597:errorcluster)  [unwired: 9 in]
            n654 = case shown="No Error" w1597 {
              selector: w1597 -> [w1613 w1621]
              tunnel: [w1616 w1620] -> w1598
              tunnel: [w1613 w1621] -> _
              tunnel: w1599 -> [w1612 w1620]
              tunnel: w1595 -> [w1611 _]
              tunnel: w1594 -> [w1610 _]
              tunnel: w1596 -> [w1609 _]
              frame No Error {
                n655 = Bundle By Name(cluster=T12 {"ModuleType"=enum."PMU", "ModuleID"=0, "UsrEvtRef"=variant, "ScriptCmd"=""} ("GetBdcstData"), "UsrEvtRef"=w1609, "ModuleID"=w1611, "ModuleType"=ModuleType."PMU", "ScriptCmd"=w1610) -> (w1617:T12)
                n656 = call "Enqueue.vi"("Priority (f)"=TRUE, "ErrorArray"=w1612, "Data"=w1617, "Msg"="GetBroadcast") -> ("ErrorArray"=w1616:errorcluster[])  [unwired: 7 in]
              }
              frame Error {
              }
            }
            n657 = call <userlib>:"AddError.vi"("Severity"="Abort" ("String"), "Priority"=u8 3, "ErrorArray"=w1598) -> ("ErrorArray"=w1603:errorcluster[], "error out"=w1604:errorcluster)  [unwired: 7 in]
            n658 = call <vilib>:"Clear Errors.vi"("error in (no error)"=w1604) -> ()  [unwired: 5 in, 2 out]
          }
          frame "GetNetImpairTime - unused" {
            n659 = Unbundle By Name(w1637) -> ("NetworkImpairModuleID"=w1624:i32)
            n660 = call "ObtainBroadcastForRegistration.vi"() -> ("error out"=w1630:errorcluster, "NetImpBroadcast"=w1636:T18)  [unwired: 10 in]
            n661 = register-events(error in=w1630, w1636) -> (reference out=w1625:refnum<event-registration>, error out=w1629:errorcluster)  [unwired: 1 in]
            n662 = call "GetNetTimeRequest.vi"("error in (no error)"=w1629, "ModuleID"=w1624) -> ("error out"=w1626:errorcluster)  [unwired: 9 in]
            n663 = case shown="No Error" w1626 {
              selector: w1626 -> [w1642 w1650]
              tunnel: [w1645 w1649] -> w1627
              tunnel: [w1642 w1650] -> w1622
              tunnel: w1628 -> [w1641 w1649]
              tunnel: w1624 -> [w1640 _]
              tunnel: w1623 -> [w1639 _]
              tunnel: w1625 -> [w1638 _]
              frame No Error {
                n664 = Bundle By Name(cluster=T12 {"ModuleType"=enum."PMU", "ModuleID"=0, "UsrEvtRef"=variant, "ScriptCmd"=""} ("GetBdcstData"), "UsrEvtRef"=w1638, "ModuleID"=w1640, "ModuleType"=ModuleType."Network", "ScriptCmd"=w1639) -> (w1646:T12)
                n665 = call "Enqueue.vi"("Priority (f)"=TRUE, "ErrorArray"=w1641, "Data"=w1646, "Msg"="GetBroadcast") -> ("ErrorArray"=w1645:errorcluster[])  [unwired: 7 in]
              }
              frame Error {
              }
            }
            n666 = call <userlib>:"AddError.vi"("Severity"="Abort" ("String"), "Priority"=u8 3, "ErrorArray"=w1627, "error in (no error)"=w1622) -> ("ErrorArray"=w1632:errorcluster[], "error out"=w1633:errorcluster)  [unwired: 6 in]
            n667 = call <vilib>:"Clear Errors.vi"("error in (no error)"=w1633) -> ()  [unwired: 5 in, 2 out]
          }
          frame "TransferTimeArrayToFlagImpair-unused" {
            n668 = Unbundle By Name(w1662) -> ("EvtConfig.Reporting Rate"=w1661:u16, "End Time"=w1660:dbl, "Start Time"=w1659:dbl)
            n669 = Unbundle By Name(w1663) -> ("FlagImpairModuleID"=w1657:i32)
            n670 = To Double Precision Float(number=w1661) -> (double precision float=w1665:dbl)
            n671 = Reciprocal(x=w1665) -> (1/x=w1664:dbl)
            n672 = call-poly <vilib>:"Ramp Pattern.vi"("start"=w1659, "end"=w1660, "delta"=w1664) -> ("Ramp Pattern"=w1658:dbl[])  [unwired: 6 in, 2 out]
            n673 = call "WriteTimeArrayRequest.vi"("dblTimeArray"=w1658, "ModuleID"=w1657) -> ("error out"=w1651:errorcluster)  [unwired: 9 in]
            n674 = call <userlib>:"AddError.vi"("Severity"="Abort" ("String"), "Priority"=u8 3, "ErrorArray"=w1652, "error in (no error)"=w1651) -> ("ErrorArray"=w1653:errorcluster[], "error out"=w1654:errorcluster)  [unwired: 6 in]
            n675 = call <vilib>:"Clear Errors.vi"("error in (no error)"=w1654) -> ()  [unwired: 5 in, 2 out]
          }
          frame "GetFlagImpairArray - unused" {
            n676 = Unbundle By Name(w1681) -> ("FlagImpairModuleID"=w1667:i32)
            n677 = call "ObtainBroadcastForRegistration.vi"() -> ("error out"=w1674:errorcluster, "FlagImpairBroadcasts"=w1680:T19)  [unwired: 10 in]
            n678 = register-events(error in=w1674, w1680) -> (reference out=w1668:refnum<event-registration>, error out=w1673:errorcluster)  [unwired: 1 in]
            n679 = call "GetFlagImpairmentArrayRequest.vi"("error in (no error)"=w1673, "ModuleID"=w1667) -> ("error out"=w1669:errorcluster)  [unwired: 9 in]
            n680 = case shown="No Error" w1669 {
              selector: w1669 -> [w1686 w1694]
              tunnel: [w1689 w1693] -> w1670
              tunnel: [w1686 w1694] -> w1671
              tunnel: w1672 -> [w1685 w1693]
              tunnel: w1667 -> [w1684 _]
              tunnel: w1666 -> [w1683 _]
              tunnel: w1668 -> [w1682 _]
              frame No Error {
                n681 = Bundle By Name(cluster=T12 {"ModuleType"=enum."PMU", "ModuleID"=0, "UsrEvtRef"=variant, "ScriptCmd"=""} ("GetBdcstData"), "UsrEvtRef"=w1682, "ModuleID"=w1684, "ModuleType"=ModuleType."Flag", "ScriptCmd"=w1683) -> (w1690:T12)
                n682 = call "Enqueue.vi"("Priority (f)"=TRUE, "ErrorArray"=w1685, "Data"=w1690, "Msg"="GetBroadcast") -> ("ErrorArray"=w1689:errorcluster[])  [unwired: 7 in]
              }
              frame Error {
              }
            }
            n683 = call <userlib>:"AddError.vi"("Severity"="Abort" ("String"), "Priority"=u8 3, "ErrorArray"=w1670, "error in (no error)"=w1671) -> ("ErrorArray"=w1676:errorcluster[], "error out"=w1677:errorcluster)  [unwired: 6 in]
            n684 = call <vilib>:"Clear Errors.vi"("error in (no error)"=w1677) -> ()  [unwired: 5 in, 2 out]
          }
          frame "AggregatePmuImpairRpts - unused" {
            # "This should be replaced in the script by the aggregate command Gets the PMU Impaired reports from all buses and indexes them together based on time stamp"
            n685 = call "GetSetFrameworkData.vi"() -> ("clFrameworkData Out"=w1713:T22)  [unwired: 11 in]
            n686 = call "ObtainBroadcastForRegistration.vi"() -> ("error out"=w1701:errorcluster, "ImpairBroadcast"=w1703:T17)  [unwired: 10 in]
            n687 = Unbundle By Name(w1713) -> ("BusClassInstances"=w1712:refnum<class "Bus.lvclass">[])
            n688 = register-events(w1703) -> (reference out=w1702:refnum<event-registration>)  [unwired: 2 in, 1 out]
            n689 = for {
              tunnel: w1714 -> [w1727]
              tunnel: w1712 -> [w1726] mode=indexing
              shift-right: [w1723] -> w1697
              shift-left: w1711 -> [w1722]
              shift-right: [w1720] -> w1707
              shift-left: T4 [{"Timestamp"=0.0, "Synx"=[], "Freq"=0.0, "ROCOF"=0.0, "ID"=0}] ("Aggregated Out") -> [w1719]
              tunnel: w1702 -> [w1718]
              tunnel: w1701 -> [w1717]
              tunnel: [w1715] -> w1700
              n690 = Unbundle By Name(w1726) -> ("PmuImpairModuleID"=w1729:i32)
              n691 = call "GetImpairReportsRequest.vi"("error in (no error)"=w1717, "ModuleID"=w1729) -> ("error out"=w1730:errorcluster)  [unwired: 9 in]
              n692 = event shown="[1] <ImpairBroadcast.ErrorReport>: User Event" {
                selector: w1718 -> [_ _ _]
                dyn-events: [_ _ _] -> w1715
                timeout: 10000 -> [_ _ _]
                tunnel: w1730 -> [w1734 _ w1740]
                tunnel: [w1732 _ _] -> w1721
                tunnel: [w1733 w1736 w1741] -> w1716
                tunnel: w1727 -> [_ _ w1742]
                event User Event {
                  n693 = event-data() -> ("Data"=w1735:variant)  [unwired: 1 in]
                  n694 = Variant To Data(error in=w1734, type=T4 [] ("clEvtReportArray"), Variant=w1735) -> (data=w1732:T4, error out=w1733:errorcluster)
                }
                event User Event {
                  n695 = event-data() -> ("Data"=w1737:variant)  [unwired: 1 in]
                  n696 = Variant To Data(type=T14 {"error"={"status"=FALSE, "code"=0, "source"=""}, "AdditionalInfo"=""} ("Cluster"), Variant=w1737) -> (data=w1738:T14)  [unwired: 1 in, 1 out]
                  n697 = Unbundle By Name(w1738) -> ("error"=w1736:errorcluster)
                }
                event Timeout {
                  n698 = event-data() -> ()  [unwired: 1 in, 1 out]
                  n699 = xnode "Error Ring"("parameter 0"=w1742) -> ("error out"=w1743:errorcluster)
                  n700 = Merge Errors(w1740, w1743) -> (w1741:errorcluster)
                }
              }
              n701 = call "AggregateReports.vi"("Additional In"=w1721, "Aggregated In"=w1719) -> ("Aggregated Out"=w1720:T4)  [unwired: 9 in]
              n702 = call <userlib>:"AddError.vi"("Severity"="Abort" ("String"), "Priority"=u8 3, "ErrorArray"=w1722, "error in (no error)"=w1716) -> ("ErrorArray"=w1723:errorcluster[])  [unwired: 6 in, 1 out]
            }
            n703 = Unregister For Events(event registration refnum=w1700) -> (error out=w1695:errorcluster)  [unwired: 1 in]
            n704 = Array Size(array=w1707) -> (size(s)=w1705:i32)
            n705 = Decrement(x=w1705) -> (x-1=w1704:i32)
            n706 = Delete From Array(array=w1707, index=w1704) -> (array with subset deleted=w1706:T4)  [unwired: 1 in, 1 out]
            n707 = call <userlib>:"AddError.vi"("Severity"="Abort" ("String"), "Priority"=u8 3, "ErrorArray"=w1697, "error in (no error)"=w1695) -> ("ErrorArray"=w1696:errorcluster[])  [unwired: 6 in, 1 out]
            n708 = Bundle By Name(cluster=w1709, "ImpairReportArray"=w1706) -> (w1708:T1)
          }
          frame "GetNetPktLoss - unused" {
            n709 = Unbundle By Name(w1766) -> ("NetworkImpairModuleID"=w1753:i32)
            n710 = call "ObtainBroadcastForRegistration.vi"() -> ("error out"=w1759:errorcluster, "NetImpBroadcast"=w1765:T18)  [unwired: 10 in]
            n711 = register-events(error in=w1759, w1765) -> (reference out=w1754:refnum<event-registration>, error out=w1758:errorcluster)  [unwired: 1 in]
            n712 = call "GetPktLossRequest.vi"("error in (no error)"=w1758, "ModuleID"=w1753) -> ("error out"=w1755:errorcluster)  [unwired: 9 in]
            n713 = case shown="No Error" w1755 {
              selector: w1755 -> [w1771 w1779]
              tunnel: [w1774 w1778] -> w1756
              tunnel: [w1771 w1779] -> w1752
              tunnel: w1757 -> [w1770 w1778]
              tunnel: w1753 -> [w1769 _]
              tunnel: w1751 -> [w1768 _]
              tunnel: w1754 -> [w1767 _]
              frame No Error {
                n714 = Bundle By Name(cluster=T12 {"ModuleType"=enum."PMU", "ModuleID"=0, "UsrEvtRef"=variant, "ScriptCmd"=""} ("GetBdcstData"), "UsrEvtRef"=w1767, "ModuleID"=w1769, "ModuleType"=ModuleType."Network", "ScriptCmd"=w1768) -> (w1775:T12)
                n715 = call "Enqueue.vi"("Priority (f)"=TRUE, "ErrorArray"=w1770, "Data"=w1775, "Msg"="GetBroadcast") -> ("ErrorArray"=w1774:errorcluster[])  [unwired: 7 in]
              }
              frame Error {
              }
            }
            n716 = call <userlib>:"AddError.vi"("Severity"="Abort" ("String"), "Priority"=u8 3, "ErrorArray"=w1756, "error in (no error)"=w1752) -> ("ErrorArray"=w1761:errorcluster[], "error out"=w1762:errorcluster)  [unwired: 6 in]
            n717 = call <vilib>:"Clear Errors.vi"("error in (no error)"=w1762) -> ()  [unwired: 5 in, 2 out]
          }
        }
        n718 = call "EnqueueError.vi"("ErrorArray"=w36) -> ("ErrorArray"=w37:errorcluster[])  [unwired: 10 in]
      }
    }
  }
  "ErrorArray Out" <- w13
  "Data out" <- w10
  "Bus" <- "Bus"
